vi "Main_Marvin Remake --.vi"() -> ()   [LabVIEW 2017]
uses:
  PCAN_Driver/ControlCAN.llb/DevType.ctl
  Marvin ATP Remake 1.5.18/PCAN_Driver/ControlCAN.llb/CAN Channel.ctl
  PCAN_Driver/ControlCAN.llb/VCI_INIT_CONFIG.ctl
  PCAN_Driver/ControlCAN.llb/InitFlag.ctl
  PCAN_Driver/ControlCAN.llb/Fliter.ctl
  PCAN_Driver/ControlCAN.llb/Mode.ctl
  <vilib>/Utility/miscctls.llb/LVRowAndColumnTypeDef.ctl
  <vilib>/Utility/sysdir.llb/System Directory Type.ctl
  <vilib>/Utility/config.llb/Read Key (String).vi
  <vilib>/Utility/config.llb/Write Key (String).vi
  <vilib>/Utility/cursorutil.llb/Set Cursor (Icon Pict).vi
  PCAN_Driver/ControlCAN.lvlib
  <vilib>/Utility/config.llb/NI_LVConfig.lvlib
panel:
  out "DSP Board S/N":string
  out "POWER Board S/N":string caption="DRIVER Board S/N"
  out "BurnInSpeed":u16
  out "SpeedCommandSpeed":u16
  out "VenableSpeed":u16
  out "CurrentTest":T1(ring)
  out "TesterVersion":string
  out "ClosePanel":bool=TRUE
  out "UUT SN Report":string
  out "Automation":bool
  out "Test Failed":bool
  out "AuxiOFFResult":bool
  out "AuxiONResult":bool
  out "SensCalResult":bool
  out "VisualInspectionResult":bool
  out "BurnResult":bool
  out "BurnSpeed":bool
  out "BurnTemp":bool
  out "BurnDC":bool
  out "TempControlResult":bool
  out "MotorTempResult":bool
  out "StopTimeResult":bool
  out "SpeedResult":bool=TRUE
  out "VenableDirectionResult":bool
  out "VenableResult":bool
  out "ComTestResult":bool=TRUE
  out "UUT SoftwareVer":string
  out "Next SN":i32
  in  "SetSN":bool
  out "Current SN":i32
  out "Cal":dbl
  out "AO[1]Meas":dbl
  out "FullSpeed2 Speed":dbl
  out "FullSpeed2 Current":dbl
  out "FullSpeed1 Current":dbl
  out "FullSpeed1 Speed":dbl
  out "MaxBurnInTempVal":dbl
  in  "Stop Burn-in":bool
  out "VISA Tester":refnum<visa-resource-name>
  out "UUT":u8
  out "CAN Status":bool
  in  "Channel 2":T2 caption="Channel" items=["Channel 1", "Channel 2"]
  out "Config_CANAT":T8 {"DevType" items=["USB-CAN"=3, "USB-CAN2"=4]; "CanIndex" items=["通道1", "通道2"]; "VCI_INIT_CONFIG"."Fliter" items=["接收所有类型"=3, "只接收标准帧"=4, "只接收扩展帧"=7]; "VCI_INIT_CONFIG"."Mode" items=["正常工作", "自测模式（环回）", "仅侦听模式"]; "VCI_INIT_CONFIG"."InitFlag" items=["使用Flash参数", "使用界面设置参数"]}
  out "Array":u64[][](array[numeric]) format="%016x"
  out "Motor Phase Current RMS":dbl
  out "Ambient Temperature":dbl
  out "Speed error":bool
  out "Commutation err":bool
  out "Under voltage/Over voltage":bool
  out "Derated drive temp":bool
  out "Motor Over temperature":bool
  out "Motor Sensor temp Fauilre":bool
  out "Drive Over temperature":bool
  out "Drive Sensor temp Failure":bool
  out "Ambient Over temp":bool
  out "Ambient Sensor temp":bool
  out "DC Voltage":dbl
  out "DC Current":dbl
  out "Power transistor Heat sink Temp.":dbl
  out "Motor Stator Temp.":dbl
  out "Motor Speed RPM":dbl
  out "ECS State":u16
  out "UUT":string="EBAY"
  in  "Logger Path":path
  in  "Report":bool
  in  "Start":bool
  in  "ATR":string[][](table)=[["Test Communication", "-", "-", "-", "-", ""], ["Set S/N", "-", "-", "-", "-", ""], ["Set Board Number", "-", "-", "-", "-", ""], [" ", "", "", "", "", ""], ["Test Communication", "-", "-", "-", "-", ""], ["Get S/N", "-", "-", "-", "", ""], ["Get Board Number", "-", "-", "-", "", ""], ["Get FW", "-", "-", "-", "", ""], ["Enable Motor", "", "", "", "", ""], ["Small position command", "", "", "", "", ""], ["Measure delta", "", "", "", "", ""], ["Velocity command", "", "", "", "", ""]]
  in  "Settings":bool
  in  "Refresh Button":bool
  out "Status":bool
  in  "VISA Marvin":refnum<visa-resource-name>="COM6"
  in  "Serial Com":bool
  in  "Help Button":bool
  out "Pannel User Message":string
  in  "Stop Button":bool
  # "Marvin"
  # "REDLER TECHNOLOGIES LTD"
  # "ver 1.2p"
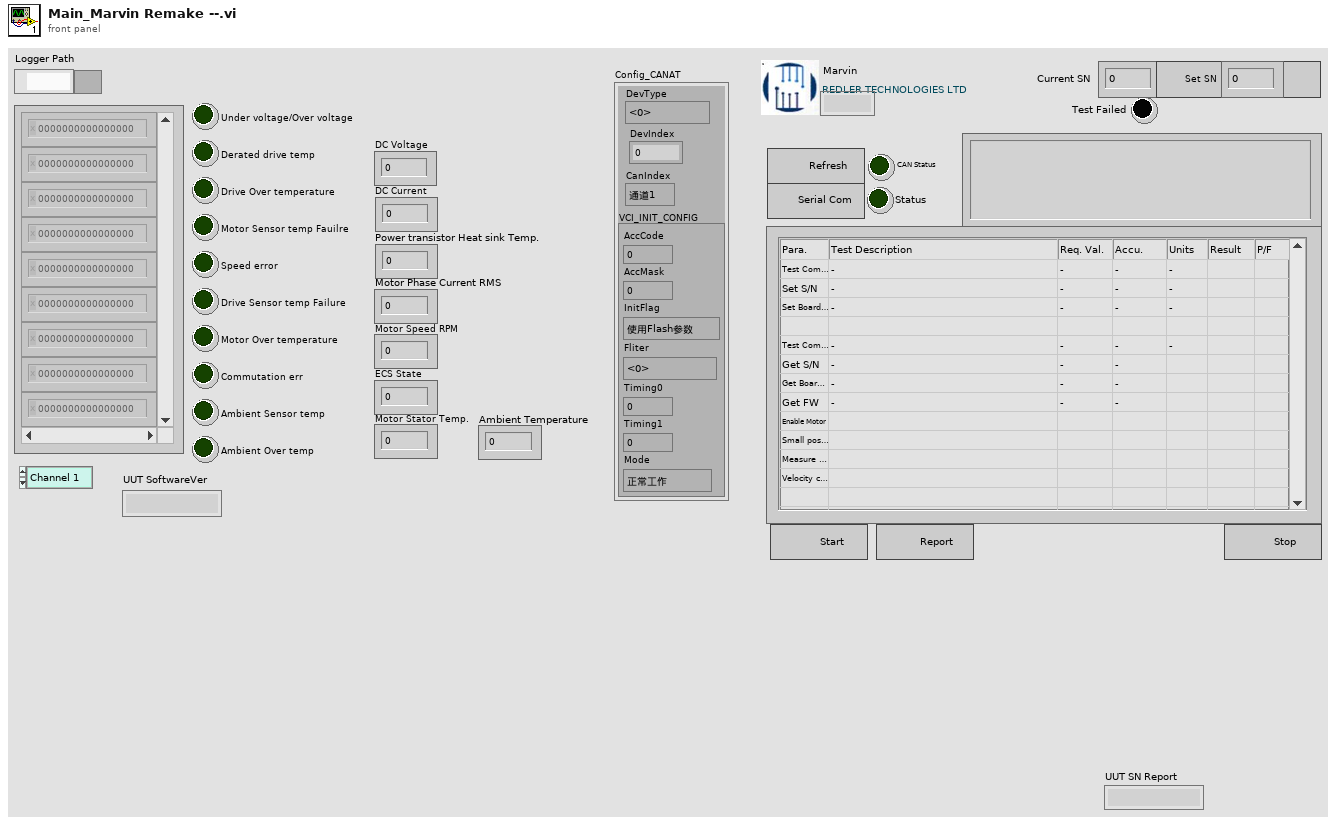
[diagram p1: front panel]
types:
  T1 = enum16{"Auxiliary", "Temp Sens Cal", "Com Test", "Enable Test", "Speed Command", "Stop Time", "Temp Control", "Burn in", "Visual Inspec", "Empty"}
  T2 = typedef "ControlCAN.lvlib/CAN Channel.ctl" = u32
  T3 = typedef "ControlCAN.lvlib/DevType.ctl" = u32
  T4 = typedef "ControlCAN.lvlib/VCI_INIT_CONFIG.ctl" = cluster{"AccCode":u32, "AccMask":u32, "InitFlag":T5, "Fliter":T6, "Timing0":u8, "Timing1":u8, "Mode":T7}
  T5 = typedef "ControlCAN.lvlib/InitFlag.ctl" = u32
  T6 = typedef "ControlCAN.lvlib/Fliter.ctl" = u8
  T7 = typedef "ControlCAN.lvlib/Mode.ctl" = u8
  T8 = cluster{"DevType":T3, "DevIndex":u32, "CanIndex":T2, "VCI_INIT_CONFIG":T4}
  T9 = cluster{"VISA":refnum<visa-resource-name>, "Array Test":enum16{"Auxiliary", "Temp Sens Cal", "Com Test", "Enable Test", "Speed Command", "Stop Time", "Temp Control", "Burn in", "Visual Inspec", "Empty"}[]}
  T10 = cluster{"ID":u32, "MSGTYPE":u8, "LEN":u8, "aDATA":u8[]}[]
  T11 = enum16{"Erase ATR Table", "Stop", "MainProgram", "Initialize"}
  T12 = typedef "NI_LVConfig.lvlib/Config Data RefNum.ctl" = refnum<k1>
  T13 = enum16{"K15", "K16", "K17", "Venable", "Firmeware", "Fan", "Power", "120C", "110C", "100C", "90C", "80C", "70C", "60C", "50C", "40C", "30C", "25C", "20C", "10C", "0C"}
  T14 = enum16{"Stop", "Result", "FullSpeed2", "MD[1]=1", "FullSpeed1", "MD[1]=0"}
  T15 = enum8{"Term1", "Term2", "Current", "Fan", "TempCPU"}
  T16 = enum16{"Stop", "AO[1]=Meas.", "TA[5]", "AO[1]=0", "Start"}
  T17 = enum16{"Stop", "BurnIn", "Ambient Temp", "MotorSpeed", "DC Current Measure", "Start"}
  T18 = enum16{"Auxiliary", "Temp Sens Cal", "Com Test", "Enable Test", "Speed Command", "Stop Time", "Temp Control", "Burn in", "Visual Inspec", "Empty"}[]
  T19 = enum16{"K15", "K16", "K17", "Venable", "Firmeware", "Fan", "Power", "120C", "110C", "100C", "90C", "80C", "70C", "60C", "50C", "40C", "30C", "25C", "20C", "10C", "0C"}[]
  T20 = enum32{"6000", "11500", "15100", "11500-2", "6000-2"}[]
  T21 = enum8{"Enabled", "Disabled", "Disabled and Grayed Out"}
  T22 = typedef "LVRowAndColumnTypeDef.ctl" = cluster{"Row":i32, "Column":i32}
  T23 = enum32{"Invalid", "Standard", "Closed", "Hidden", "Minimized", "Maximized"}
  T24 = cluster{"ID":u32, "MSGTYPE":u8, "LEN":u8, "aDATA":u8[]}
  T25 = enum16{"open", "replace", "create", "open or create", "replace or create", "replace or create with confirmation"}
  T26 = typedef "ControlCAN.lvlib/VCI_CAN_OBJ.ctl" = cluster{"ID":u32, "TimeStamp":u32, "TimeFlag":u8, "SendType":u8, "RemoteFlag":u8, "ExternFlag":u8, "DataLen":u8, "Data":u8[], "Reserved":u8[]}
  T27 = cluster{"Type":enum16{"接收", "发送"}, "Channel":T2, "Time":timestamp, "VCI_CAN_OBJ":T26}[]
  T28 = cluster{"Type":enum16{"接收", "发送"}, "Channel":T2, "Time":timestamp, "VCI_CAN_OBJ":T26}
  T29 = typedef "LVPoint32TypeDef.ctl" = cluster{"Horizontal":i32, "Vertical":i32}
  T30 = enum8{"Term1", "Term2", "Current", "Fan", "TempCPU"}[]
  T31 = typedef "System Directory Type.ctl" = i32
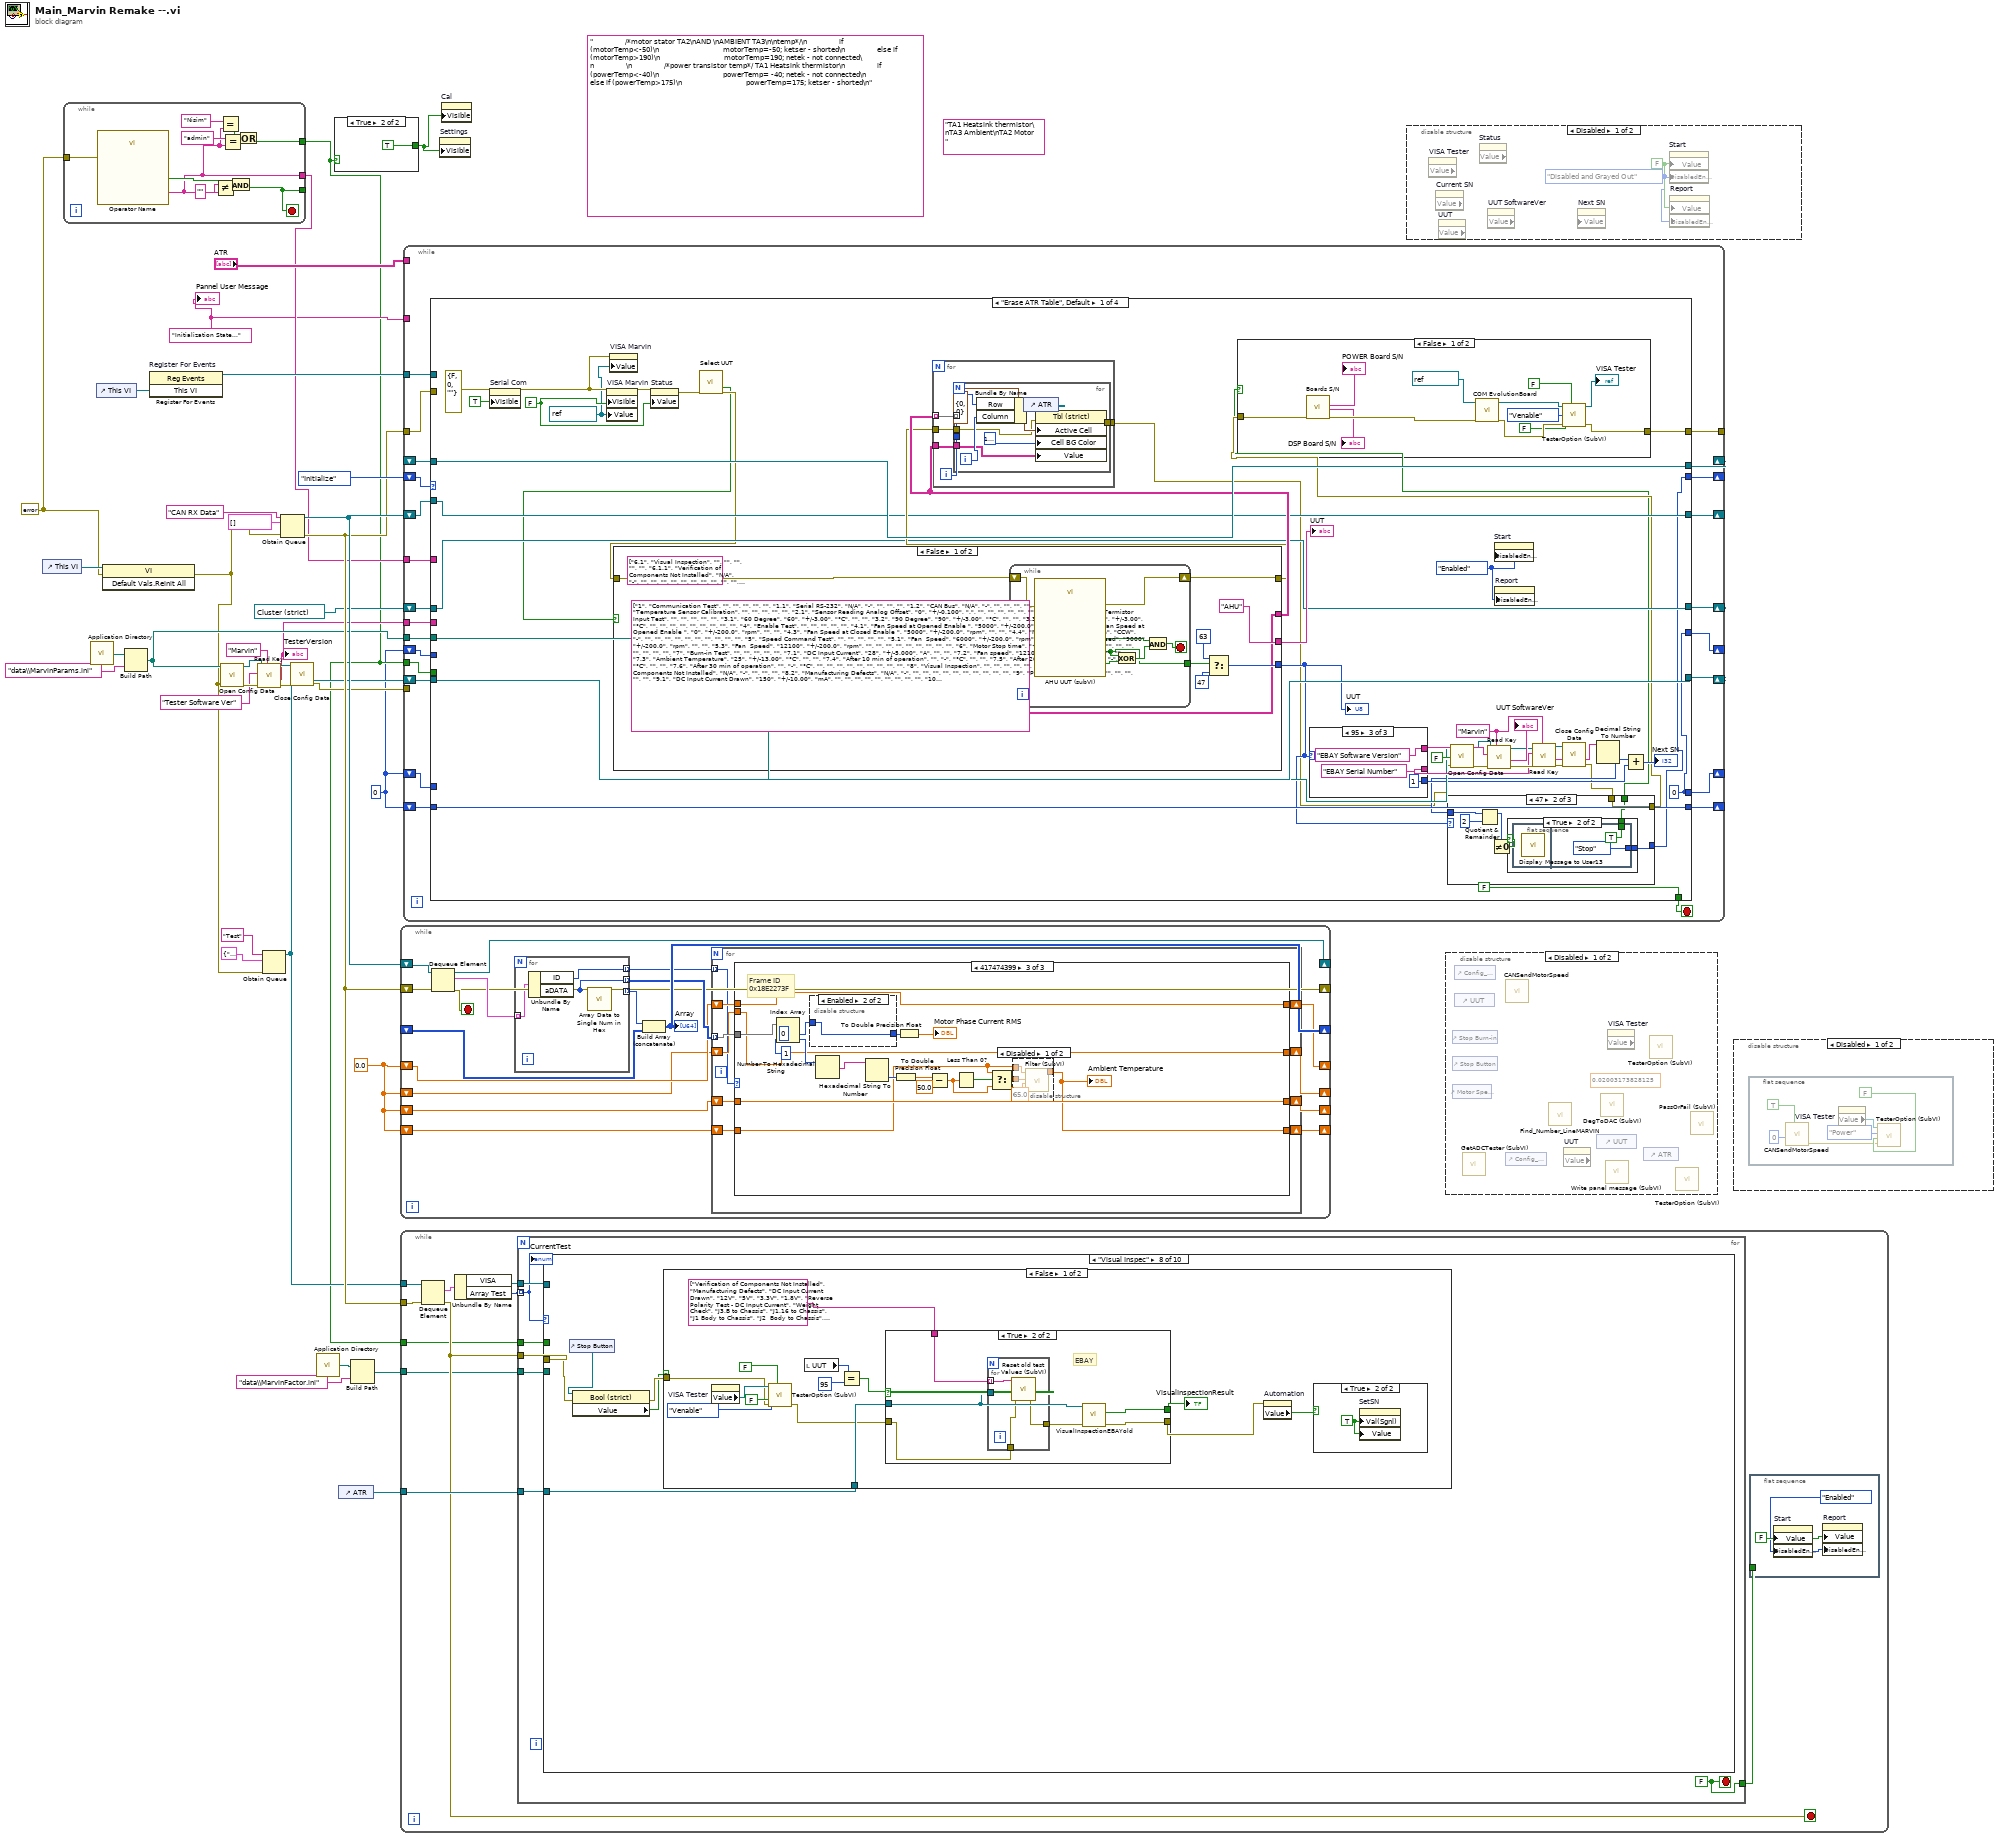
[diagram p0: block diagram]
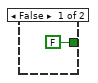
[diagram p2: hidden frame]
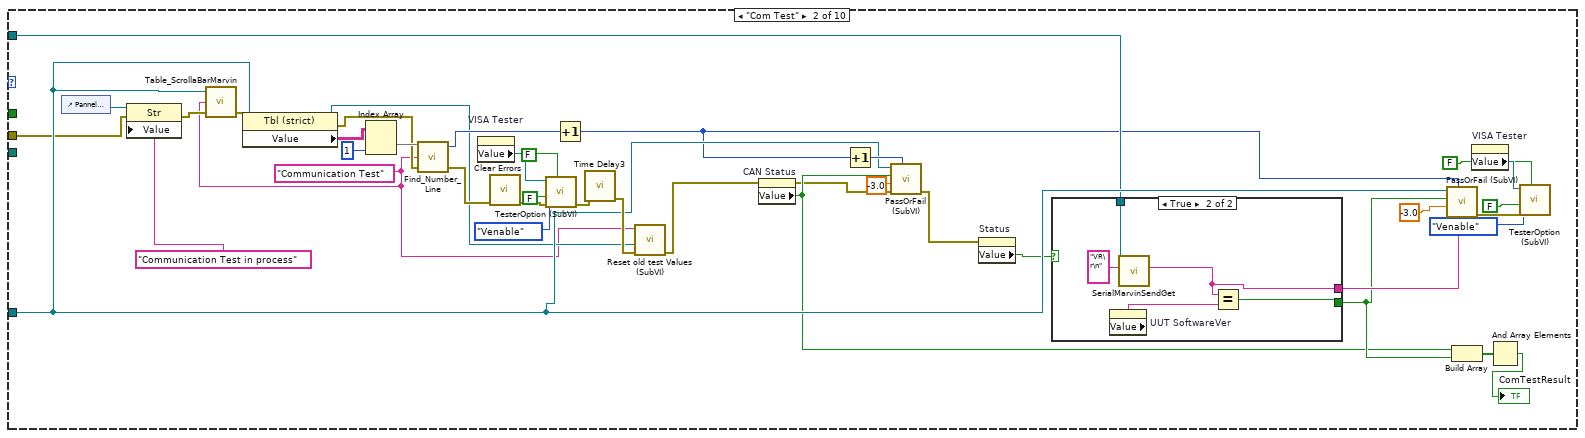
[diagram p7: hidden frame]
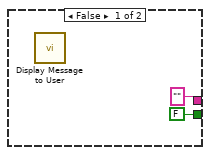
[diagram p8: hidden frame]
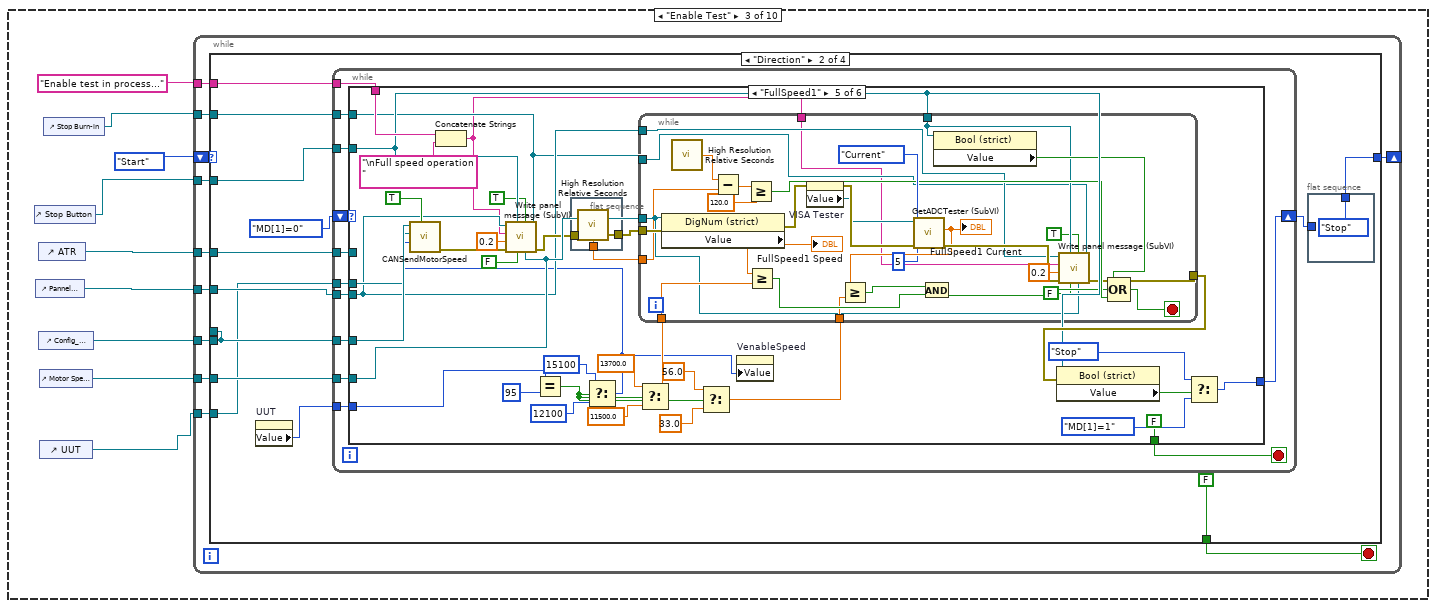
[diagram p9: hidden frame]
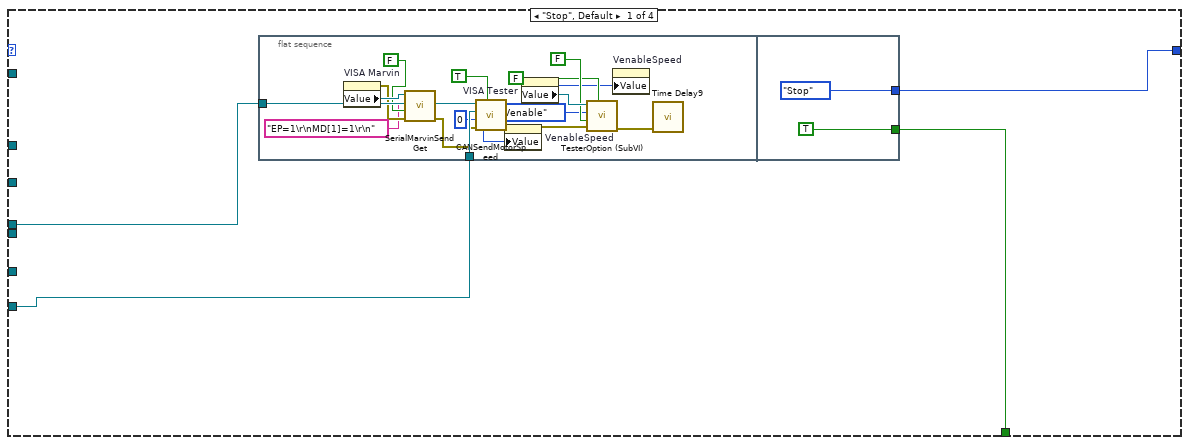
[diagram p10: hidden frame]
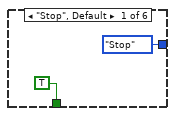
[diagram p11: hidden frame]
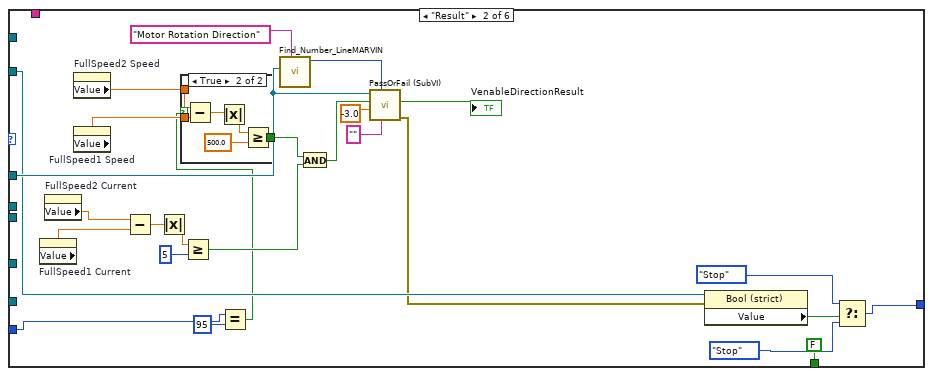
[diagram p12: hidden frame]
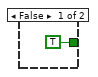
[diagram p13: hidden frame]
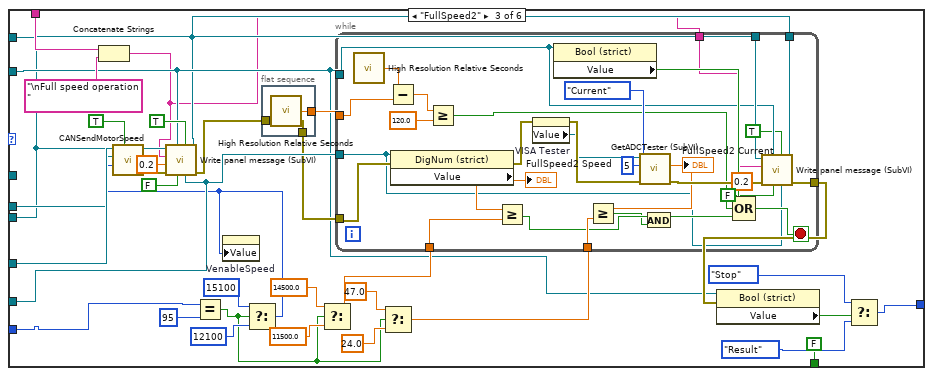
[diagram p14: hidden frame]
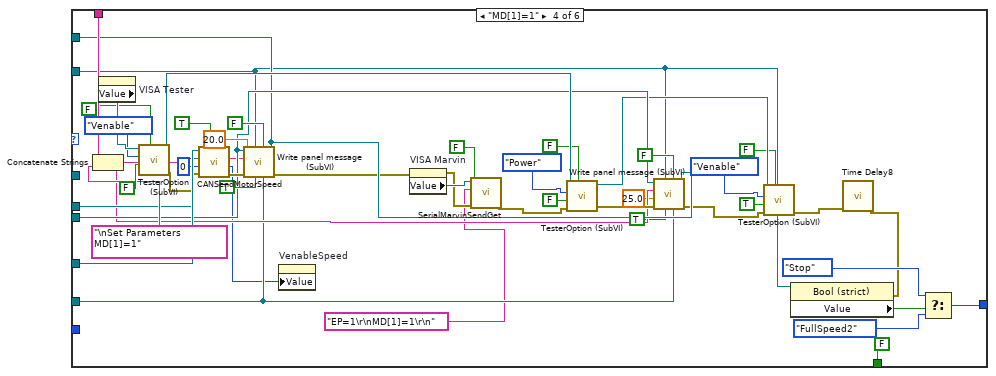
[diagram p15: hidden frame]
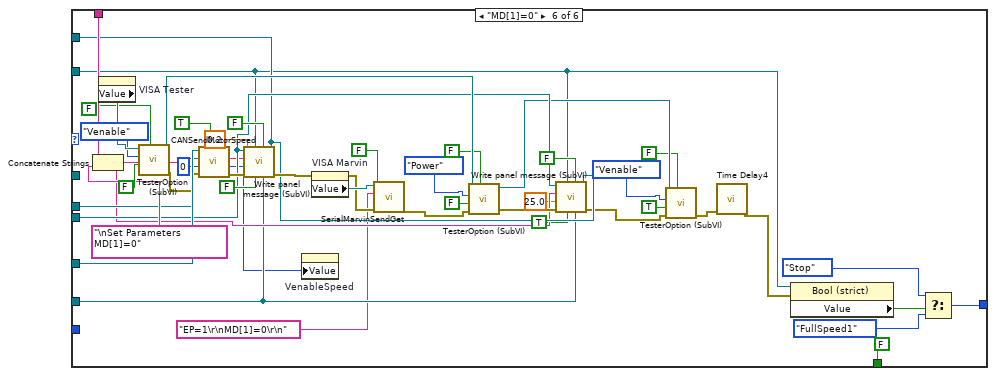
[diagram p16: hidden frame]
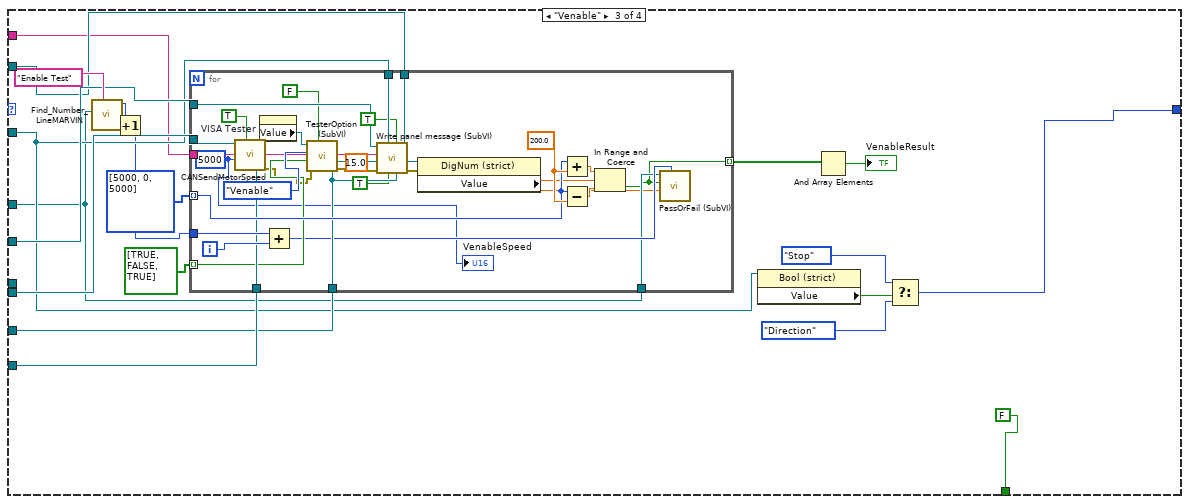
[diagram p17: hidden frame]
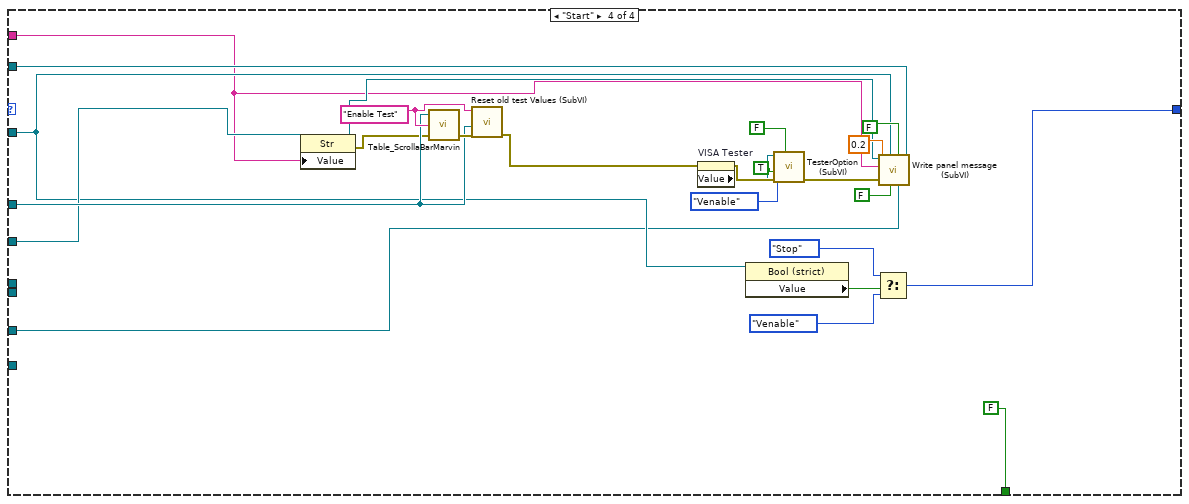
[diagram p18: hidden frame]
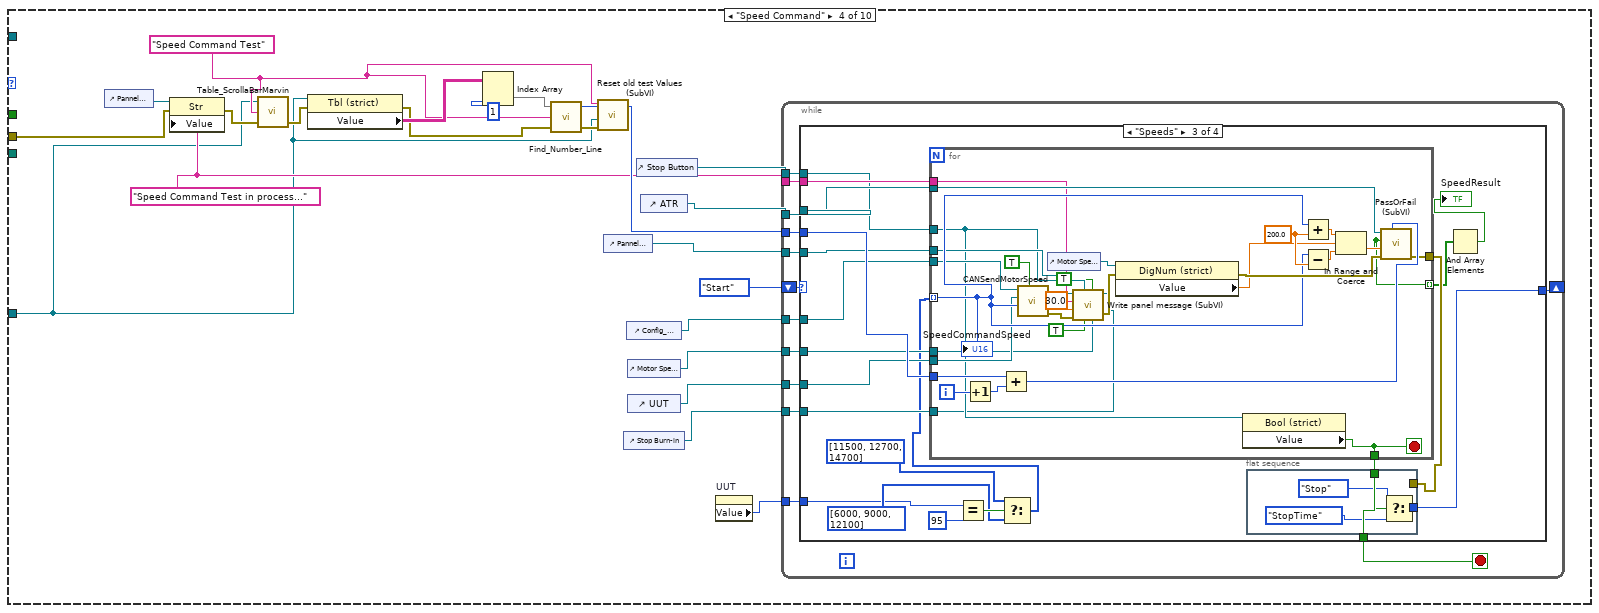
[diagram p19: hidden frame]
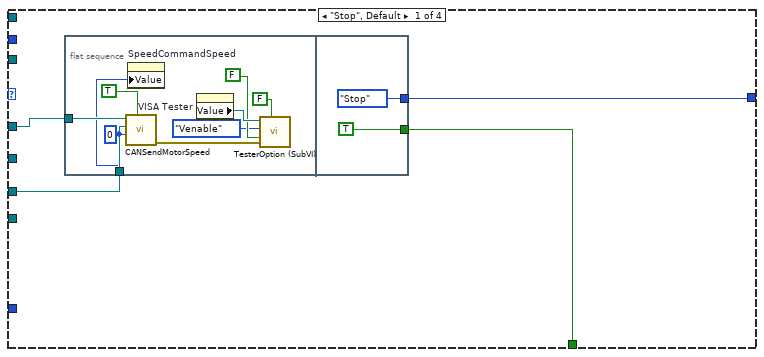
[diagram p20: hidden frame]
diagram:
  (unwired) "TA1 Heatsink thermistor\nTA3 Ambient\nTA2 Motor "
  (unwired) "                /*motor stator TA2\nAND \nAMBIENT TA3\n\ntemp*/\n                if (motorTemp<-50)\n                                motorTemp=-50; ketser - shorted\n                else if (motorTemp>190)\n                                motorTemp=190; netek - not connected\n                \n                /*power transistor temp*/ TA1 Heatsink thermistor\n                if (powerTemp<-40)\n                                powerTemp= -40; netek - not connected\n                else if (powerTemp>175)\n                                powerTemp=175; ketser - shorted\n"
  w19 = "Initialization State..."
  w1 = 0
  w26 = 0.0
  w4 = errorcluster {"status"=FALSE, "code"=0, "source"=""} ("error in (no error)")
  n1 = control-ref of="This VI"() -> (w5:refnum<vi>)
  n2 = while {
    tunnel: [w44] -> _
    tunnel: [w40] -> w21
    tunnel: [w41] -> w2
    tunnel: w4 -> [w37]
    stop <- w44 stop-if-true
    n3 = call "Operator Name"("error in (no error)"=w37) -> ("Operator Name"=w40:string, "OK"=w45:bool)  [unwired: 16 in, 1 out]
    n4 = Not Equal?(x=w40, y="") -> (x != y?=w46:bool)
    n5 = Equal?(x="Nisim", y=w40) -> (x = y?=w38:bool)
    n6 = Equal?(x="admin", y=w40) -> (x = y?=w42:bool)
    n7 = And(x=w45, y=w46) -> (x .and. y?=w44:bool)
    n8 = Or(x=w38, y=w42) -> (x .or. y?=w41:bool)
  }
  n9 = call <vilib>:"Application Directory.vi"() -> ("Application Directory"=w25:path)
  n10 = control-ref of="This VI"() -> (w23:refnum<vi>)
  n11 = invoke class="VI" method="Default Vals.Reinit All"(reference=w5, error in=w4) -> (error out=w3:errorcluster)  [unwired: 1 in, 2 out]
  n12 = Build Path(base path=w25, name or relative path="data\\MarvinParams.ini") -> (appended path=w8:path)
  n13 = register-events "Register For Events"(w23) -> (reference out=w22:refnum<event-registration>)  [unwired: 2 in, 1 out]
  n14 = call <vilib>:"Open Config Data.vi"("error in (no error)"=w3, "configuration file path"=w8) -> ("error out"=w14:errorcluster, "refnum"=w13:T12)  [unwired: 1 in, 7 out]
  n15 = call-poly <vilib>:"Read Key.vi"("section"="Marvin", "error in (no error)"=w14, "key"="Tester Software Ver", "refnum"=w13) -> ("error out"=w11:errorcluster, "value"=w6:string, "refnum out"=w10:T12)  [unwired: 2 in, 3 out]
  "TesterVersion" <- w6
  n16 = Obtain Queue(name (unnamed)="Test", element data type=T9 {"VISA"="COM1", "Array Test"=[]}, error in (no error)=w3) -> (queue out=w30:refnum<queue>)  [unwired: 2 in, 2 out]
  n17 = Obtain Queue(name (unnamed)="CAN RX Data", element data type=T10 [], error in (no error)=w3) -> (queue out=w33:refnum<queue>, error out=w31:errorcluster)  [unwired: 2 in, 1 out]
  n18 = call <vilib>:"Close Config Data.vi"("error in (no error)"=w11, "refnum"=w10) -> ("error out"=w9:errorcluster)  [unwired: 8 in, 1 out]
  n19 = call <vilib>:"Application Directory.vi"() -> ("Application Directory"=w16:path)
  n20 = case shown="True" w2 {
    tunnel: [FALSE TRUE] -> w20
    frame False {
    }
    frame True {
    }
  }
  n21 = control-ref of="ATR"() -> (w18:refnum<vi>)
  n22 = Build Path(base path=w16, name or relative path="data\\MarvinFactor.ini") -> (appended path=w15:path)
  n23 = while {
    shift-right: [w65] -> _
    shift-left: w33 -> [w67]
    shift-right: [w63] -> _
    shift-left: _ -> [w64]
    shift-right: [w59] -> _
    shift-left: w31 -> [w59]
    shift-right: [w57] -> _
    shift-left: w26 -> [w58]
    shift-right: [w56] -> _
    shift-left: w26 -> [w55]
    shift-right: [w54] -> _
    shift-left: w26 -> [w53]
    shift-right: [w52] -> _
    shift-left: w26 -> [w51]
    stop <- w66 stop-if-true
    n24 = Dequeue Element(queue=w67, error in (no error)=w59) -> (queue out=w65:refnum<queue>, element=w60:T10, error out=w66:errorcluster)  [unwired: 1 in, 1 out]
    n25 = for {
      tunnel: [w213] -> w62 mode=indexing
      tunnel: w60 -> [w212] mode=indexing
      tunnel: [w211] -> w61 mode=indexing
      tunnel: [w210] -> w50 mode=indexing
      n26 = Unbundle By Name(w212) -> ("ID"=w210:u32, "aDATA"=w211:u8[])
      n27 = call "Array Data to Single Num in Hex.vi"("aDATA"=w211) -> ("Numeric"=w213:u64)  [unwired: 10 in]
    }
    n28 = Build Array (concatenate)(w62, w64) -> (w63:u64[][])
    "Array" <- w63
    n29 = for {
      tunnel: w61 -> [w77] mode=indexing
      shift-right: [w75] -> w57
      shift-left: w58 -> [w76]
      shift-right: [w74] -> w56
      shift-left: w55 -> [w73]
      shift-right: [w72] -> w54
      shift-left: w53 -> [w71]
      shift-right: [w70] -> w52
      shift-left: w51 -> [w69]
      tunnel: w50 -> [w68] mode=indexing
      n30 = case shown="417474399" w68 {
        tunnel: w77 -> [w114 w162 w200]
        tunnel: w76 -> [w88 w151 w189]
        tunnel: [w87 w151 w189] -> w75
        tunnel: [w84 w150 w188] -> w74
        tunnel: w73 -> [w83 w150 w188]
        tunnel: [w80 w149 w187] -> w72
        tunnel: w71 -> [w79 w149 w187]
        tunnel: [w78 w148 w183] -> w70
        tunnel: w69 -> [w78 w148 w182]
        frame 417408863, Default {
          # "Frame ID\n0x18E1273F"
          n31 = Index Array(array=w114, index #1=0 ("index"), index #2=1 ("index"), index #3=2 ("index"), index #4=3 ("index"), index #5=4 ("index"), index #6=5 ("index"), index #7=6 ("index"), index #8=7 ("index")) -> (element #1=w98:u8, element #2=w100:u8, element #3=w101:u8, element #4=w105:u8, element #5=w108:u8, element #6=w112:u8, element #7=w113:u8, element #8=w111:u8)
          n32 = Number To Hexadecimal String(2:w111) -> (0:w125:string)  [unwired: 1 in]
          n33 = Join Numbers(hi=w113, lo=w112) -> ((hi.lo)=w132:u16)
          n34 = Join Numbers(hi=w101, lo=w100) -> ((hi.lo)=w102:u16)
          n35 = Number To Hexadecimal String(2:w108) -> (0:w109:string)  [unwired: 1 in]
          n36 = Number To Hexadecimal String(2:w132) -> (0:w131:string)  [unwired: 1 in]
          n37 = Number To Hexadecimal String(2:w98) -> (0:w99:string)  [unwired: 1 in]
          n38 = Number To Hexadecimal String(2:w102) -> (0:w103:string)  [unwired: 1 in]
          n39 = Number To Hexadecimal String(2:w105) -> (0:w106:string)  [unwired: 1 in]
          n40 = Hexadecimal String To Number(string=w125) -> (number=w124:u32)  [unwired: 2 in, 1 out]
          n41 = To Double Precision Float(number=w124) -> (double precision float=→"DC Current":dbl)
          n42 = Hexadecimal String To Number(string=w109) -> (number=w110:u32)  [unwired: 2 in, 1 out]
          n43 = Hexadecimal String To Number(string=w131) -> (number=w130:u32)  [unwired: 2 in, 1 out]
          n44 = Hexadecimal String To Number(string=w99) -> (number=w96:u32)  [unwired: 2 in, 1 out]
          n45 = Hexadecimal String To Number(string=w103) -> (number=w104:u32)  [unwired: 2 in, 1 out]
          n46 = Hexadecimal String To Number(string=w106) -> (number=w107:u32)  [unwired: 2 in, 1 out]
          n47 = To Double Precision Float(number=u32 10 ("y")) -> (double precision float=w128:dbl)
          n48 = To Double Precision Float(number=w130) -> (double precision float=w127:dbl)
          n49 = To Double Precision Float(number=w110) -> (double precision float=w93:dbl)
          n50 = To Double Precision Float(number=w104) -> (double precision float=w89:dbl)
          n51 = To Double Precision Float(number=w107) -> (double precision float=w95:dbl)
          n52 = Divide(x=w127, y=w128) -> (x/y=→"DC Voltage":dbl)
          n53 = To Unsigned Word Integer(number=w96) -> (unsigned 16bit integer=→"ECS State":u16)
          n54 = disable-structure shown="Enabled" {
            disable-tunnel: w89 -> [w146 w147]
            disable-tunnel: w88 -> [w145 _]
            disable-tunnel: [w143 w147] -> w87
            frame Disabled {
              n55 = call "Filter (SubVI).vi"("Delta"=5000.0, "NewVal"=w146, "OldVal"=w145) -> ("Val"=w143:dbl)  [unwired: 8 in]
            }
            frame Enabled {
            }
          }
          "Motor Speed RPM" <- w87
          n56 = Subtract(x=w93, y=50.0 ("x")) -> (x-y=w82:dbl)
          n57 = Subtract(x=w95, y=50.0 ("x")) -> (x-y=w85:dbl)
          n58 = Less Than 0?(x=w85) -> (x < 0?=w91:bool)
          n59 = Less Than 0?(x=w82) -> (x < 0?=w90:bool)
          n60 = Select(t=w83, s=w91, f=w85) -> (s? t:f=w86:dbl)
          n61 = Select(t=w79, s=w90, f=w82) -> (s? t:f=w81:dbl)
          n62 = disable-structure shown="Enabled" {
            disable-tunnel: w86 -> [w141 w142]
            disable-tunnel: [w140 w142] -> w84
            disable-tunnel: w83 -> [w139 _]
            frame Disabled {
              n63 = call "Filter (SubVI).vi"("Delta"=130.0, "NewVal"=w141, "OldVal"=w139) -> ("Val"=w140:dbl)  [unwired: 8 in]
            }
            frame Enabled {
            }
          }
          "Motor Stator Temp." <- w84
          n64 = disable-structure shown="Enabled" {
            disable-tunnel: w81 -> [w136 w137]
            disable-tunnel: [w134 w137] -> w80
            disable-tunnel: w79 -> [w133 _]
            frame Disabled {
              n65 = call "Filter (SubVI).vi"("Delta"=100.0, "NewVal"=w136, "OldVal"=w133) -> ("Val"=w134:dbl)  [unwired: 8 in]
            }
            frame Enabled {
            }
          }
          "Power transistor Heat sink Temp." <- w80
        }
        frame 417539935 {
          # "Framde ID\n0x18E3273F"
          n66 = control-ref of="UUT"() -> (w152:refnum<vi>)
          n67 = property on="Property Node" class="DigNum (strict)"(reference=w152) -> ("Value"=w153:u8)  [unwired: 1 in, 2 out]
          n68 = Index Array(array=w162, index #1=0 ("index"), index #2=1 ("index")) -> (element #1=w160:u8, element #2=w155:u8)
          n69 = Number To Boolean Array(number=w160) -> (Boolean array=w159:bool[])
          n70 = Number To Boolean Array(number=w155) -> (Boolean array=w157:bool[])
          n71 = Boolean To (0,1)(Boolean=w157) -> (0, 1=w154:i16[])
          n72 = Boolean To (0,1)(Boolean=w159) -> (0, 1=w158:i16[])
          n73 = case shown="95" w153 {
            tunnel: w154 -> [_ w163]
            frame 0, Default {
            }
            frame 95 {
              n74 = for {
                tunnel: w163 -> [w168] mode=indexing
                i -> [w164]
                stop <- w166 stop-if-true
                n75 = Not Equal To 0?(x=w168) -> (x != 0?=w167:bool)
                n76 = case shown="0, Default" w164 {
                  tunnel: w167 -> [w169 w170]
                  frame 0, Default {
                    "Ambient Sensor temp" <- w169
                  }
                  frame 1 {
                    "Ambient Over temp" <- w170
                  }
                }
                n77 = Equal?(x=w164, y=1.0) -> (x = y?=w166:bool)
              }
            }
          }
          n78 = for {
            tunnel: w158 -> [w172] mode=indexing
            i -> [w173]
            n79 = Not Equal To 0?(x=w172) -> (x != 0?=w171:bool)
            n80 = case shown="1" w173 {
              tunnel: w171 -> [w174 w175 w176 w177 w178 w179 w180 w181]
              frame 0, Default {
                "Drive Sensor temp Failure" <- w174
              }
              frame 1 {
                "Drive Over temperature" <- w175
              }
              frame 2 {
                "Motor Sensor temp Fauilre" <- w176
              }
              frame 3 {
                "Motor Over temperature" <- w177
              }
              frame 4 {
                "Derated drive temp" <- w178
              }
              frame 5 {
                "Under voltage/Over voltage" <- w179
              }
              frame 6 {
                "Commutation err" <- w180
              }
              frame 7 {
                "Speed error" <- w181
              }
            }
          }
        }
        frame 417474399 {
          # "Frame ID\n0x18E2273F"
          n81 = Index Array(array=w200, index #1=0 ("index"), index #2=1 ("index")) -> (element #1=w197:u8, element #2=w194:u8)
          n82 = disable-structure shown="Enabled" {
            disable-tunnel: [w208 w209] -> w198
            disable-tunnel: w197 -> [w207 w209]
            frame Disabled {
              n83 = Number To Hexadecimal String(2:w207) -> (0:w206:string)  [unwired: 1 in]
              n84 = Hexadecimal String To Number(string=w206) -> (number=w208:u32)  [unwired: 2 in, 1 out]
            }
            frame Enabled {
            }
          }
          n85 = Number To Hexadecimal String(2:w194) -> (0:w192:string)  [unwired: 1 in]
          n86 = Hexadecimal String To Number(string=w192) -> (number=w193:u32)  [unwired: 2 in, 1 out]
          n87 = To Double Precision Float(number=w193) -> (double precision float=w191:dbl)
          n88 = To Double Precision Float(number=w198) -> (double precision float=→"Motor Phase Current RMS":dbl)
          n89 = Subtract(x=w191, y=50.0) -> (x-y=w185:dbl)
          n90 = Less Than 0?(x=w185) -> (x < 0?=w186:bool)
          n91 = Select(t=w182, s=w186, f=w185) -> (s? t:f=w184:dbl)
          n92 = disable-structure shown="Disabled" {
            disable-tunnel: w184 -> [w204 w205]
            disable-tunnel: [w202 w205] -> w183
            disable-tunnel: w182 -> [w201 _]
            frame Disabled {
              n93 = call "Filter (SubVI).vi"("Delta"=65.0, "NewVal"=w204, "OldVal"=w201) -> ("Val"=w202:dbl)  [unwired: 8 in]
            }
            frame Enabled {
            }
          }
          "Ambient Temperature" <- w183
        }
      }
    }
  }
  n94 = while {
    tunnel: w18 -> [w223]
    tunnel: w31 -> [w221]
    tunnel: w30 -> [w222]
    tunnel: w15 -> [w215]
    tunnel: w2 -> [w214]
    stop <- w217 stop-if-true
    n95 = Dequeue Element(queue=w222, error in (no error)=w221) -> (element=w220:T9, error out=w217:errorcluster)  [unwired: 1 in, 2 out]
    n96 = Unbundle By Name(w220) -> ("VISA"=w219:refnum<visa-resource-name>, "Array Test"=w218:T18)
    n97 = for {
      tunnel: w218 -> [w229] mode=indexing
      tunnel: w219 -> [w232]
      tunnel: w223 -> [w231]
      tunnel: w217 -> [w230]
      tunnel: [w228] -> w216
      tunnel: w215 -> [w227]
      tunnel: w214 -> [w226]
      stop <- w228 stop-if-true
      w228 = FALSE
      n98 = case shown="\"Visual Inspec\"" w229 {
        tunnel: w232 -> [_ w257 _ _ w846 _ _ _ w1453 w1660]
        tunnel: w231 -> [_ w264 _ w681 w842 w1019 _ w1413 w1460 w1673]
        tunnel: w230 -> [_ w261 _ w696 w852 w1001 _ w1411 w1458 w1672]
        tunnel: w227 -> [_ _ _ _ _ w1003 _ _ _ _]
        tunnel: w226 -> [_ _ _ _ _ _ w1171 _ _ _]
        frame "Empty", Default {
        }
        frame "Com Test" {
          w240 = "Communication Test" ("Test Paragraph")
          n99 = control-ref of="Pannel User Message"() -> (w262:refnum<vi>)
          n100 = property class="Str"(reference=w262, error in=w261, "Value"="Communication Test in process") -> (error out=w260:errorcluster)  [unwired: 1 out]
          n101 = call "Table_ScrollaBarMarvin.vi"("error in"=w260, "Line to focus"=w240, "reference in"=w264) -> ("error out"=w263:errorcluster)  [unwired: 2 out]
          n102 = property class="Tbl (strict)"(reference=w264, error in=w263) -> (reference out=w241:refnum<vi>, error out=w270:errorcluster, "Value"=w271:string[][])
          n103 = Index Array(array=w271, index (col)=1 ("disabled index (col)")) -> (element=w272:string[])  [unwired: 1 in]
          n104 = call "Find_Number_Line.vi"("error in"=w270, "Test Paragraph"=w240, "Row Headers[]"=w272) -> ("error out"=w268:errorcluster, "Line number"=w267:i32)  [unwired: 1 out]
          n105 = property on="VISA Tester" class="VISAName"() -> ("Value"=w251:refnum<visa-resource-name>)  [unwired: 2 in, 2 out]
          n106 = call <vilib>:"Clear Errors.vi"("error in (no error)"=w268) -> ("error out"=w253:errorcluster)  [unwired: 5 in, 1 out]
          n107 = call "TesterOption (SubVI).vi"("2 Options"=FALSE, "error in (no error)"=w253, "On/Off"=FALSE, "Tester Option"=T13."Venable", "VISA Refnum in"=w251) -> ("error out"=w252:errorcluster)  [unwired: 5 in, 1 out]
          n108 = Increment(x=w267) -> (x+1=w233:i32)
          n109 = call "Time Delay3"("error in (no error)"=w252) -> ("error out"=w265:errorcluster)  [unwired: 10 in]
          n110 = call "Reset old test Values (SubVI).vi"("error in"=w265, "Atr in"=w241, "Test Paragraph"=w240) -> ("error out"=w235:errorcluster)  [unwired: 8 in]
          n111 = property on="CAN Status" class="Bool (strict)"(error in=w235) -> (error out=w234:errorcluster, "Value"=w236:bool)  [unwired: 1 in, 1 out]
          n112 = Increment(x=w233) -> (x+1=w266:i32)
          n113 = call "PassOrFail (SubVI).vi"("index (row)"=w266, "error in (no error)"=w234, "Data in"=-3.0, "Pass?Fail"=w236, "Table in"=w264) -> ("error out"=w256:errorcluster)  [unwired: 6 in]
          n114 = property on="Status" class="Bool (strict)"(error in=w256) -> ("Value"=w258:bool)  [unwired: 1 in, 2 out]
          n115 = case shown="True" w258 {
            tunnel: w257 -> [_ w279]
            tunnel: [FALSE w276] -> w238
            tunnel: ["" ("read buffer") w275] -> w255
            frame False {
              n116 = call "Display Message to User"() -> ()  [unwired: 10 in, 2 out]
            }
            frame True {
              n117 = property on="UUT SoftwareVer" class="Str"() -> ("Value"=w277:string)  [unwired: 2 in, 2 out]
              n118 = call "SerialMarvinSendGet.vi"("write buffer"="VR\r\n", "VISA resource name"=w279) -> ("read buffer"=w275:string)  [unwired: 8 in, 1 out]
              n119 = Equal?(x=w275, y=w277) -> (x = y?=w276:bool)
            }
          }
          n120 = call "PassOrFail (SubVI).vi"("String Res"=w255, "index (row)"=w233, "Data in"=-3.0, "Pass?Fail"=w238, "Table in"=w264) -> ("error out"=w247:errorcluster)  [unwired: 6 in]
          n121 = Build Array(w236, w238) -> (w239:bool[])
          n122 = property on="VISA Tester" class="VISAName"() -> ("Value"=w246:refnum<visa-resource-name>)  [unwired: 2 in, 2 out]
          n123 = And Array Elements(Boolean array=w239) -> (logical AND=→"ComTestResult":bool)
          n124 = call "TesterOption (SubVI).vi"("2 Options"=FALSE, "error in (no error)"=w247, "On/Off"=FALSE, "Tester Option"=T13."Venable", "VISA Refnum in"=w246) -> ()  [unwired: 5 in, 2 out]
        }
        frame "Enable Test" {
          n125 = control-ref of="Stop Button"() -> (w282:refnum<vi>)
          n126 = control-ref of="Pannel User Message"() -> (w284:refnum<vi>)
          n127 = control-ref of="ATR"() -> (w283:refnum<vi>)
          n128 = control-ref of="Config_CANAT"() -> (w285:refnum<vi>)
          n129 = control-ref of="Motor Speed RPM"() -> (w286:refnum<vi>)
          n130 = control-ref of="UUT"() -> (w287:refnum<vi>)
          n131 = control-ref of="Stop Burn-in"() -> (w288:refnum<vi>)
          n132 = while {
            shift-right: [w293] -> _
            shift-left: enum16{"Stop", "Direction", "Venable", "Start"}."Start" -> [w299]
            tunnel: w282 -> [w298]
            tunnel: w283 -> [w297]
            tunnel: w284 -> [w296]
            tunnel: w285 -> [w289]
            tunnel: w286 -> [w295]
            tunnel: w287 -> [w290]
            tunnel: w288 -> [w292]
            tunnel: "Enable test in process..." ("Strin") -> [w291]
            stop <- w294 stop-if-true
            n133 = case shown="\"Direction\"" w299 {
              tunnel: w298 -> [_ w331 w613 w660]
              tunnel: w297 -> [_ w326 w611 w667]
              tunnel: w296 -> [_ w329 w615 w666]
              tunnel: w289 -> [_ w332 w618 _]
              tunnel: w295 -> [_ w328 w616 w658]
              tunnel: w290 -> [w300 w322 w617 _]
              tunnel: [w303 FALSE FALSE FALSE] -> w294
              tunnel: [w301 w325 w612 w664] -> w293
              tunnel: w292 -> [_ w330 w614 w659]
              tunnel: w291 -> [_ w327 w610 w657]
              tunnel: w289 -> [w302 _ _ _]
              frame "Stop", Default {
                n134 = flat-sequence {
                  tunnel: w300 -> [w315]
                  tunnel: w302 -> [w314]
                  tunnel: [TRUE] -> w303
                  tunnel: [enum16{"Stop", "Direction", "Venable", "Start"}."Stop"] -> w301
                  frame #0 {
                    w304 = u16 0 ("Motor Speed RPM")
                    n135 = property on="VISA Marvin" class="VISAName"() -> (error out=w308:errorcluster, "Value"=w309:refnum<visa-resource-name>)  [unwired: 2 in, 1 out]
                    n136 = call "SerialMarvinSendGet.vi"("error in (no error)"=w308, "Clear Log"=FALSE, "write buffer"="EP=1\r\nMD[1]=1\r\n", "VISA resource name"=w309) -> ("error out"=w305:errorcluster)  [unwired: 6 in, 1 out]
                    n137 = call "CANSendMotorSpeed.vi"("Remote"=TRUE, "error in (no error)"=w305, "Motor Speed RPM"=w304, "UUT"=w315, "CAN Cluster in"=w314) -> ("error out"=w317:errorcluster)  [unwired: 6 in]
                    n138 = property on="VenableSpeed" class="DigNum (strict)"("Value"=w304) -> ()  [unwired: 2 in, 2 out]
                    n139 = property on="VISA Tester" class="VISAName"() -> ("Value"=w318:refnum<visa-resource-name>)  [unwired: 2 in, 2 out]
                    n140 = call "TesterOption (SubVI).vi"("2 Options"=FALSE, "error in (no error)"=w317, "On/Off"=FALSE, "Tester Option"=T13."Venable", "VISA Refnum in"=w318) -> ("error out"=w310:errorcluster)  [unwired: 5 in, 1 out]
                    n141 = property on="VenableSpeed" class="DigNum (strict)"("Value"=w304) -> ()  [unwired: 2 in, 2 out]
                    n142 = call "Time Delay9"("error in (no error)"=w310) -> ()  [unwired: 10 in, 1 out]
                  }
                  frame #1 {
                  }
                }
              }
              frame "Direction" {
                n143 = property on="UUT" class="DigNum (strict)"() -> ("Value"=w321:u8)  [unwired: 2 in, 2 out]
                n144 = while {
                  shift-right: [w345] -> w324
                  shift-left: T14."MD[1]=0" -> [w346]
                  tunnel: w332 -> [w343]
                  tunnel: w322 -> [w342]
                  tunnel: w331 -> [w341]
                  tunnel: w330 -> [w340]
                  tunnel: w329 -> [w339]
                  tunnel: w328 -> [w338]
                  tunnel: w327 -> [w337]
                  tunnel: w326 -> [w336]
                  tunnel: w321 -> [w335]
                  stop <- w344 stop-if-true
                  n145 = case shown="\"FullSpeed1\"" w346 {
                    tunnel: [T14."Stop" w370 w412 w492 w525 w605] -> w345
                    tunnel: [TRUE FALSE FALSE FALSE FALSE FALSE] -> w344
                    tunnel: w343 -> [_ _ w410 w486 w523 w599]
                    tunnel: w342 -> [_ _ w406 w466 w519 w578]
                    tunnel: w341 -> [_ w357 w386 w457 w502 w568]
                    tunnel: w340 -> [_ _ w384 w467 w500 w579]
                    tunnel: w339 -> [_ _ w385 w468 w501 w580]
                    tunnel: w338 -> [_ _ w402 w455 w516 w574]
                    tunnel: w337 -> [_ _ w397 w476 w514 w588]
                    tunnel: w336 -> [_ w361 _ _ _ _]
                    tunnel: w335 -> [_ w349 w382 _ w495 _]
                    frame "Stop", Default {
                    }
                    frame "Result" {
                      n146 = property on="FullSpeed1 Current" class="DigNum (strict)"() -> ("Value"=w365:dbl)  [unwired: 2 in, 2 out]
                      n147 = property on="FullSpeed2 Current" class="DigNum (strict)"() -> ("Value"=w366:dbl)  [unwired: 2 in, 2 out]
                      n148 = property on="FullSpeed2 Speed" class="DigNum (strict)"() -> ("Value"=w368:dbl)  [unwired: 2 in, 2 out]
                      n149 = property on="FullSpeed1 Speed" class="DigNum (strict)"() -> ("Value"=w367:dbl)  [unwired: 2 in, 2 out]
                      n150 = Subtract(x=w366, y=w365) -> (x-y=w364:dbl)
                      n151 = Absolute Value(x=w364) -> (abs(x)=w353:dbl)
                      n152 = Greater Or Equal?(x=w353, y=u32 5) -> (x >= y?=w359:bool)
                      n153 = Equal?(x=w349, y=u8 95) -> (x = y?=w351:bool)
                      n154 = case shown="True" w351 {
                        tunnel: w368 -> [_ w379]
                        tunnel: w367 -> [_ w378]
                        tunnel: [TRUE w375] -> w360
                        frame False {
                        }
                        frame True {
                          n155 = Subtract(x=w379, y=w378) -> (x-y=w380:dbl)
                          n156 = Absolute Value(x=w380) -> (abs(x)=w377:dbl)
                          n157 = Greater Or Equal?(x=w377, y=500.0) -> (x >= y?=w375:bool)
                        }
                      }
                      n158 = call "Find_Number_LineMARVIN.vi"("Test Paragraph"="Motor Rotation Direction", "TableIn"=w361) -> ("Line number"=w358:i32)  [unwired: 3 in, 3 out]
                      n159 = And(x=w360, y=w359) -> (x .and. y?=w350:bool)
                      "VenableDirectionResult" <- w350
                      n160 = call "PassOrFail (SubVI).vi"("String Res"="", "index (row)"=w358, "Data in"=-3.0, "Pass?Fail"=w350, "Table in"=w361) -> ("error out"=w356:errorcluster)  [unwired: 6 in]
                      n161 = property class="Bool (strict)"(reference=w357, error in=w356) -> ("Value"=w373:bool)  [unwired: 2 out]
                      n162 = Select(t=T14."Stop", s=w373, f=T14."Stop") -> (s? t:f=w370:T14)
                    }
                    frame "FullSpeed2" {
                      n163 = Concatenate Strings(w397, "\nFull speed operation " ("string")) -> (w383:string)
                      n164 = Equal?(x=w382, y=u8 95) -> (x = y?=w392:bool)
                      n165 = Select(t=u16 15100, s=w392, f=u16 12100 ("y")) -> (s? t:f=w381:u16)
                      n166 = call "CANSendMotorSpeed.vi"("Remote"=TRUE, "Motor Speed RPM"=w381, "UUT"=w406, "CAN Cluster in"=w410) -> ("error out"=w404:errorcluster)  [unwired: 7 in]
                      n167 = call "Write panel message (SubVI).vi"("Stop BurnIn"=w384, 4:"rpm"=w402, 5:"rpm"=TRUE ("rpm"), "PrintTime"=FALSE, "Stop"=w386, "error in (no error)"=w404, "Time to wait"=0.2, "Strin"=w383, "String in"=w385) -> ("error out"=w389:errorcluster)  [unwired: 2 in]
                      n168 = property on="VenableSpeed" class="DigNum (strict)"("Value"=w381) -> ()  [unwired: 2 in, 2 out]
                      n169 = flat-sequence {
                        tunnel: w389 -> [w417]
                        tunnel: [w417] -> w388
                        tunnel: [w416] -> w387
                        frame #0 {
                          n170 = call <vilib>:"High Resolution Relative Seconds.vi"() -> ("relative seconds"=w416:dbl)
                        }
                      }
                      n171 = Select(t=14500.0, s=w392, f=11500.0) -> (s? t:f=w391:dbl)
                      n172 = Select(t=47.0, s=w392, f=24.0) -> (s? t:f=w390:dbl)
                      n173 = while {
                        tunnel: w402 -> [w419]
                        tunnel: w388 -> [w447]
                        tunnel: [w427] -> w399
                        tunnel: w391 -> [w440]
                        tunnel: w390 -> [w439]
                        tunnel: w387 -> [w435]
                        tunnel: w386 -> [w425]
                        tunnel: w385 -> [w426]
                        tunnel: w384 -> [w423]
                        tunnel: w383 -> [w422]
                        stop <- w437 stop-if-true
                        n174 = call <vilib>:"High Resolution Relative Seconds.vi"() -> ("relative seconds"=w436:dbl)
                        n175 = Subtract(x=w436, y=w435) -> (x-y=w434:dbl)
                        n176 = property class="DigNum (strict)"(reference=w419, error in=w447) -> (error out=w446:errorcluster, "Value"=w441:dbl)  [unwired: 1 out]
                        "FullSpeed2 Speed" <- w441
                        n177 = Greater Or Equal?(x=w434, y=120.0) -> (x >= y?=w432:bool)
                        n178 = Greater Or Equal?(x=w441, y=w440) -> (x >= y?=w431:bool)
                        n179 = property on="VISA Tester" class="VISAName"(error in=w446) -> (error out=w445:errorcluster, "Value"=w444:refnum<visa-resource-name>)  [unwired: 1 in, 1 out]
                        n180 = property class="Bool (strict)"(reference=w425) -> ("Value"=w430:bool)  [unwired: 1 in, 2 out]
                        n181 = call "GetADCTester (SubVI).vi"("error in (no error)"=w445, "GetADCTester"=T15."Current", "TimeToGet"=5, "VISA Refnum in"=w444) -> ("error out"=w442:errorcluster, "ADCValOutput Single"=w438:dbl)  [unwired: 5 in, 1 out]
                        "FullSpeed2 Current" <- w438
                        n182 = Greater Or Equal?(x=w438, y=w439) -> (x >= y?=w428:bool)
                        n183 = And(x=w431, y=w428) -> (x .and. y?=w429:bool)
                        n184 = Compound Arithmetic op=OR(w430, w432, w429) -> (w437:bool)
                        n185 = call "Write panel message (SubVI).vi"("Stop BurnIn"=w423, 4:"rpm"=w419, 5:"rpm"=TRUE ("rpm"), "PrintTime"=FALSE, "Stop"=w425, "error in (no error)"=w442, "Time to wait"=0.2, "Strin"=w422, "String in"=w426) -> ("error out"=w427:errorcluster)  [unwired: 2 in]
                      }
                      n186 = property class="Bool (strict)"(reference=w386, error in=w399) -> ("Value"=w415:bool)  [unwired: 2 out]
                      n187 = Select(t=T14."Stop", s=w415, f=T14."Result") -> (s? t:f=w412:T14)
                    }
                    frame "MD[1]=1" {
                      w448 = u16 0 ("Motor Speed RPM")
                      n188 = Concatenate Strings(w476, "\nSet Parameters MD[1]=1" ("Strin")) -> (w465:string)
                      n189 = property on="VISA Tester" class="VISAName"() -> ("Value"=w481:refnum<visa-resource-name>)  [unwired: 2 in, 2 out]
                      n190 = call "TesterOption (SubVI).vi"("2 Options"=FALSE, "On/Off"=FALSE, "Tester Option"=T13."Venable", "VISA Refnum in"=w481) -> ("error out"=w482:errorcluster, "VISA Refnum out"=w472:refnum<visa-resource-name>)  [unwired: 6 in]
                      n191 = call "CANSendMotorSpeed.vi"("Remote"=TRUE, "error in (no error)"=w482, "Motor Speed RPM"=w448, "UUT"=w466, "CAN Cluster in"=w486) -> ("error out"=w484:errorcluster)  [unwired: 6 in]
                      n192 = call "Write panel message (SubVI).vi"("Stop BurnIn"=w467, 4:"rpm"=w455, 5:"rpm"=FALSE ("rpm"), "PrintTime"=TRUE, "Stop"=w457, "error in (no error)"=w484, "Time to wait"=20.0, "Strin"=w465, "String in"=w468) -> ("error out"=w454:errorcluster)  [unwired: 2 in]
                      n193 = property on="VenableSpeed" class="DigNum (strict)"("Value"=w448) -> ()  [unwired: 2 in, 2 out]
                      n194 = property on="VISA Marvin" class="VISAName"(error in=w454) -> (error out=w483:errorcluster, "Value"=w488:refnum<visa-resource-name>)  [unwired: 1 in, 1 out]
                      n195 = call "SerialMarvinSendGet.vi"("error in (no error)"=w483, "Clear Log"=FALSE, "write buffer"="EP=1\r\nMD[1]=1\r\n", "VISA resource name"=w488) -> ("error out"=w471:errorcluster)  [unwired: 6 in, 1 out]
                      n196 = call "TesterOption (SubVI).vi"("2 Options"=FALSE, "error in (no error)"=w471, "On/Off"=FALSE, "Tester Option"=T13."Power", "VISA Refnum in"=w472) -> ("error out"=w469:errorcluster, "VISA Refnum out"=w458:refnum<visa-resource-name>)  [unwired: 5 in]
                      n197 = call "Write panel message (SubVI).vi"("Stop BurnIn"=w467, 4:"rpm"=w455, 5:"rpm"=FALSE ("rpm"), "PrintTime"=TRUE, "Stop"=w457, "error in (no error)"=w469, "Time to wait"=25.0, "Strin"=w465, "String in"=w468) -> ("error out"=w459:errorcluster)  [unwired: 2 in]
                      n198 = call "TesterOption (SubVI).vi"("2 Options"=FALSE, "error in (no error)"=w459, "On/Off"=TRUE, "Tester Option"=T13."Venable", "VISA Refnum in"=w458) -> ("error out"=w456:errorcluster)  [unwired: 5 in, 1 out]
                      n199 = call "Time Delay8"("error in (no error)"=w456) -> ("error out"=w452:errorcluster)  [unwired: 10 in]
                      n200 = property class="Bool (strict)"(reference=w457, error in=w452) -> ("Value"=w493:bool)  [unwired: 2 out]
                      n201 = Select(t=T14."Stop", s=w493, f=T14."FullSpeed2") -> (s? t:f=w492:T14)
                    }
                    frame "FullSpeed1" {
                      n202 = Concatenate Strings(w514, "\nFull speed operation " ("string")) -> (w499:string)
                      n203 = Equal?(x=w495, y=u8 95) -> (x = y?=w512:bool)
                      n204 = flat-sequence {
                        tunnel: w505 -> [w530]
                        tunnel: [w530] -> w504
                        tunnel: [w529] -> w503
                        frame #0 {
                          n205 = call <vilib>:"High Resolution Relative Seconds.vi"() -> ("relative seconds"=w529:dbl)
                        }
                      }
                      n206 = Select(t=u16 15100, s=w512, f=u16 12100 ("y")) -> (s? t:f=w494:u16)
                      n207 = call "CANSendMotorSpeed.vi"("Remote"=TRUE, "Motor Speed RPM"=w494, "UUT"=w519, "CAN Cluster in"=w523) -> ("error out"=w517:errorcluster)  [unwired: 7 in]
                      n208 = call "Write panel message (SubVI).vi"("Stop BurnIn"=w500, 4:"rpm"=w516, 5:"rpm"=TRUE ("rpm"), "PrintTime"=FALSE, "Stop"=w502, "error in (no error)"=w517, "Time to wait"=0.2, "Strin"=w499, "String in"=w501) -> ("error out"=w505:errorcluster)  [unwired: 2 in]
                      n209 = Select(t=13700.0, s=w512, f=11500.0) -> (s? t:f=w507:dbl)
                      n210 = Select(t=56.0, s=w512, f=33.0) -> (s? t:f=w506:dbl)
                      n211 = while {
                        tunnel: w516 -> [w532]
                        tunnel: w504 -> [w560]
                        tunnel: [w540] -> w515
                        tunnel: w507 -> [w552]
                        tunnel: w506 -> [w549]
                        tunnel: w503 -> [w547]
                        tunnel: w502 -> [w538]
                        tunnel: w501 -> [w539]
                        tunnel: w500 -> [w536]
                        tunnel: w499 -> [w535]
                        stop <- w554 stop-if-true
                        n212 = property class="DigNum (strict)"(reference=w532, error in=w560) -> (error out=w559:errorcluster, "Value"=w553:dbl)  [unwired: 1 out]
                        "FullSpeed1 Speed" <- w553
                        n213 = call <vilib>:"High Resolution Relative Seconds.vi"() -> ("relative seconds"=w548:dbl)
                        n214 = Subtract(x=w548, y=w547) -> (x-y=w546:dbl)
                        n215 = Greater Or Equal?(x=w546, y=120.0) -> (x >= y?=w544:bool)
                        n216 = Greater Or Equal?(x=w553, y=w552) -> (x >= y?=w551:bool)
                        n217 = property on="VISA Tester" class="VISAName"(error in=w559) -> (error out=w558:errorcluster, "Value"=w557:refnum<visa-resource-name>)  [unwired: 1 in, 1 out]
                        n218 = call "GetADCTester (SubVI).vi"("error in (no error)"=w558, "GetADCTester"=T15."Current", "TimeToGet"=5, "VISA Refnum in"=w557) -> ("error out"=w555:errorcluster, "ADCValOutput Single"=w550:dbl)  [unwired: 5 in, 1 out]
                        "FullSpeed1 Current" <- w550
                        n219 = Greater Or Equal?(x=w550, y=w549) -> (x >= y?=w541:bool)
                        n220 = And(x=w541, y=w551) -> (x .and. y?=w542:bool)
                        n221 = property class="Bool (strict)"(reference=w538) -> ("Value"=w543:bool)  [unwired: 1 in, 2 out]
                        n222 = call "Write panel message (SubVI).vi"("Stop BurnIn"=w536, 4:"rpm"=w532, 5:"rpm"=TRUE ("rpm"), "PrintTime"=FALSE, "Stop"=w538, "error in (no error)"=w555, "Time to wait"=0.2, "Strin"=w535, "String in"=w539) -> ("error out"=w540:errorcluster)  [unwired: 2 in]
                        n223 = Compound Arithmetic op=OR(w543, w542, w544) -> (w554:bool)
                      }
                      n224 = property on="VenableSpeed" class="DigNum (strict)"("Value"=w494) -> ()  [unwired: 2 in, 2 out]
                      n225 = property class="Bool (strict)"(reference=w502, error in=w515) -> ("Value"=w528:bool)  [unwired: 2 out]
                      n226 = Select(t=T14."Stop", s=w528, f=T14."MD[1]=1") -> (s? t:f=w525:T14)
                    }
                    frame "MD[1]=0" {
                      w561 = u16 0 ("Motor Speed RPM")
                      n227 = Concatenate Strings(w588, "\nSet Parameters MD[1]=0" ("Strin")) -> (w577:string)
                      n228 = property on="VISA Tester" class="VISAName"() -> ("Value"=w594:refnum<visa-resource-name>)  [unwired: 2 in, 2 out]
                      n229 = call "TesterOption (SubVI).vi"("2 Options"=FALSE, "On/Off"=FALSE, "Tester Option"=T13."Venable", "VISA Refnum in"=w594) -> ("error out"=w595:errorcluster, "VISA Refnum out"=w584:refnum<visa-resource-name>)  [unwired: 6 in]
                      n230 = call "CANSendMotorSpeed.vi"("Remote"=TRUE, "error in (no error)"=w595, "Motor Speed RPM"=w561, "UUT"=w578, "CAN Cluster in"=w599) -> ("error out"=w597:errorcluster)  [unwired: 6 in]
                      n231 = call "Write panel message (SubVI).vi"("Stop BurnIn"=w579, 4:"rpm"=w574, 5:"rpm"=FALSE ("rpm"), "PrintTime"=FALSE, "Stop"=w568, "error in (no error)"=w597, "Time to wait"=0.2, "Strin"=w577, "String in"=w580) -> ("error out"=w591:errorcluster)  [unwired: 2 in]
                      n232 = property on="VenableSpeed" class="DigNum (strict)"("Value"=w561) -> ()  [unwired: 2 in, 2 out]
                      n233 = property on="VISA Marvin" class="VISAName"(error in=w591) -> (error out=w596:errorcluster, "Value"=w601:refnum<visa-resource-name>)  [unwired: 1 in, 1 out]
                      n234 = call "SerialMarvinSendGet.vi"("error in (no error)"=w596, "Clear Log"=FALSE, "write buffer"="EP=1\r\nMD[1]=0\r\n", "VISA resource name"=w601) -> ("error out"=w583:errorcluster)  [unwired: 6 in, 1 out]
                      n235 = call "TesterOption (SubVI).vi"("2 Options"=FALSE, "error in (no error)"=w583, "On/Off"=FALSE, "Tester Option"=T13."Power", "VISA Refnum in"=w584) -> ("error out"=w581:errorcluster, "VISA Refnum out"=w569:refnum<visa-resource-name>)  [unwired: 5 in]
                      n236 = call "Write panel message (SubVI).vi"("Stop BurnIn"=w579, 4:"rpm"=w574, 5:"rpm"=FALSE ("rpm"), "PrintTime"=TRUE, "Stop"=w568, "error in (no error)"=w581, "Time to wait"=25.0, "Strin"=w577, "String in"=w580) -> ("error out"=w570:errorcluster)  [unwired: 2 in]
                      n237 = call "TesterOption (SubVI).vi"("2 Options"=FALSE, "error in (no error)"=w570, "On/Off"=TRUE, "Tester Option"=T13."Venable", "VISA Refnum in"=w569) -> ("error out"=w567:errorcluster)  [unwired: 5 in, 1 out]
                      n238 = call "Time Delay4"("error in (no error)"=w567) -> ("error out"=w563:errorcluster)  [unwired: 10 in]
                      n239 = property class="Bool (strict)"(reference=w568, error in=w563) -> ("Value"=w606:bool)  [unwired: 2 out]
                      n240 = Select(t=T14."Stop", s=w606, f=T14."FullSpeed1") -> (s? t:f=w605:T14)
                    }
                  }
                }
                n241 = flat-sequence {
                  tunnel: [enum16{"Stop", "Direction", "Venable", "Start"}."Stop"] -> w325
                  tunnel: w324 -> [_]
                  frame #0 {
                  }
                }
              }
              frame "Venable" {
                n242 = call "Find_Number_LineMARVIN.vi"("Test Paragraph"="Enable Test", "TableIn"=w611) -> ("Line number"=w619:i32)  [unwired: 3 in, 3 out]
                n243 = Increment(x=w619) -> (x+1=w607:i32)
                n244 = for {
                  tunnel: u16[] [5000, 0, 5000] -> [w649] mode=indexing
                  tunnel: bool[] [TRUE, FALSE, TRUE] -> [w645] mode=indexing
                  tunnel: w607 -> [w650]
                  tunnel: w618 -> [w648]
                  tunnel: w617 -> [w647]
                  tunnel: w616 -> [w636]
                  tunnel: w615 -> [w640]
                  tunnel: w613 -> [w639]
                  tunnel: w614 -> [w638]
                  tunnel: w611 -> [w632]
                  tunnel: w610 -> [w630]
                  tunnel: [w629] -> w609 mode=indexing
                  i -> [w651]
                  w627 = u16 5000 ("Motor Speed RPM")
                  w653 = 200.0 ("y")
                  n245 = call "CANSendMotorSpeed.vi"("Remote"=TRUE, "Motor Speed RPM"=w627, "UUT"=w647, "CAN Cluster in"=w648) -> ("error out"=w644:errorcluster)  [unwired: 7 in]
                  n246 = property on="VISA Tester" class="VISAName"() -> ("Value"=w643:refnum<visa-resource-name>)  [unwired: 2 in, 2 out]
                  n247 = Add(x=w650, y=w651) -> (x+y=w633:i32)
                  n248 = call "TesterOption (SubVI).vi"("2 Options"=FALSE, "error in (no error)"=w644, "On/Off"=w645, "Tester Option"=T13."Venable", "VISA Refnum in"=w643) -> ("error out"=w642:errorcluster)  [unwired: 5 in, 1 out]
                  n249 = call "Write panel message (SubVI).vi"("Stop BurnIn"=w638, 4:"rpm"=w636, 5:"rpm"=TRUE ("rpm"), "PrintTime"=TRUE, "Stop"=w639, "error in (no error)"=w642, "Time to wait"=15.0, "Strin"=w630, "String in"=w640) -> ("error out"=w641:errorcluster)  [unwired: 2 in]
                  n250 = property class="DigNum (strict)"(reference=w636, error in=w641) -> ("Value"=w631:dbl)  [unwired: 2 out]
                  n251 = Add(x=w649, y=w653) -> (x+y=w655:dbl)
                  n252 = Subtract(x=w649, y=w653) -> (x-y=w654:dbl)
                  n253 = In Range and Coerce(upper limit=w655, x=w631, lower limit=w654) -> (In Range?=w629:bool)  [unwired: 1 out]
                  n254 = call "PassOrFail (SubVI).vi"("index (row)"=w633, "Data in"=w631, "Pass?Fail"=w629, "Table in"=w632) -> ()  [unwired: 7 in, 1 out]
                  "VenableSpeed" <- w627
                }
                n255 = property class="Bool (strict)"(reference=w613) -> ("Value"=w626:bool)  [unwired: 1 in, 2 out]
                n256 = And Array Elements(Boolean array=w609) -> (logical AND=→"VenableResult":bool)
                n257 = Select(t=enum16{"Stop", "Direction", "Venable", "Start"}."Stop", s=w626, f=enum16{"Stop", "Direction", "Venable", "Start"}."Direction") -> (s? t:f=w612:enum16{"Stop", "Direction", "Venable", "Start"})
              }
              frame "Start" {
                w675 = "Enable Test" ("Test Paragraph")
                n258 = property class="Str"(reference=w666, "Value"=w657) -> (reference out=w676:refnum<vi>, error out=w663:errorcluster)  [unwired: 1 in]
                n259 = call "Table_ScrollaBarMarvin.vi"("error in"=w663, "Line to focus"=w675, "reference in"=w667) -> ("error out"=w672:errorcluster)  [unwired: 2 out]
                n260 = call "Reset old test Values (SubVI).vi"("error in"=w672, "Atr in"=w667, "Test Paragraph"=w675) -> ("error out"=w671:errorcluster)  [unwired: 8 in]
                n261 = property on="VISA Tester" class="VISAName"(error in=w671) -> (error out=w670:errorcluster, "Value"=w669:refnum<visa-resource-name>)  [unwired: 1 in, 1 out]
                n262 = property class="Bool (strict)"(reference=w660) -> ("Value"=w680:bool)  [unwired: 1 in, 2 out]
                n263 = call "TesterOption (SubVI).vi"("2 Options"=FALSE, "error in (no error)"=w670, "On/Off"=TRUE, "Tester Option"=T13."Venable", "VISA Refnum in"=w669) -> ("error out"=w668:errorcluster)  [unwired: 5 in, 1 out]
                n264 = Select(t=enum16{"Stop", "Direction", "Venable", "Start"}."Stop", s=w680, f=enum16{"Stop", "Direction", "Venable", "Start"}."Venable") -> (s? t:f=w664:enum16{"Stop", "Direction", "Venable", "Start"})
                n265 = call "Write panel message (SubVI).vi"("Stop BurnIn"=w659, 4:"rpm"=w658, 5:"rpm"=FALSE ("rpm"), "PrintTime"=FALSE, "Stop"=w660, "error in (no error)"=w668, "Time to wait"=0.2, "Strin"=w657, "String in"=w676) -> ()  [unwired: 2 in, 1 out]
              }
            }
          }
        }
        frame "Speed Command" {
          w685 = "Speed Command Test in process..." ("Value")
          w682 = "Speed Command Test" ("Test Paragraph")
          n266 = control-ref of="Pannel User Message"() -> (w697:refnum<vi>)
          n267 = property class="Str"(reference=w697, error in=w696, "Value"=w685) -> (error out=w695:errorcluster)  [unwired: 1 out]
          n268 = call "Table_ScrollaBarMarvin.vi"("error in"=w695, "Line to focus"=w682, "reference in"=w681) -> ("error out"=w698:errorcluster)  [unwired: 2 out]
          n269 = property class="Tbl (strict)"(reference=w681, error in=w698) -> (error out=w700:errorcluster, "Value"=w701:string[][])  [unwired: 1 out]
          n270 = Index Array(array=w701, index (col)=1 ("disabled index (col)")) -> (element=w702:string[])  [unwired: 1 in]
          n271 = call "Find_Number_Line.vi"("error in"=w700, "Test Paragraph"=w682, "Row Headers[]"=w702) -> ("error out"=w683:errorcluster, "Line number"=w686:i32)  [unwired: 1 out]
          n272 = call "Reset old test Values (SubVI).vi"("error in"=w683, "Atr in"=w681, "Test Paragraph"=w682) -> ()  [unwired: 8 in, 1 out]
          n273 = control-ref of="Pannel User Message"() -> (w690:refnum<vi>)
          n274 = control-ref of="Stop Burn-in"() -> (w694:refnum<vi>)
          n275 = control-ref of="Config_CANAT"() -> (w691:refnum<vi>)
          n276 = control-ref of="Motor Speed RPM"() -> (w692:refnum<vi>)
          n277 = control-ref of="UUT"() -> (w693:refnum<vi>)
          n278 = control-ref of="Stop Button"() -> (w688:refnum<vi>)
          n279 = control-ref of="ATR"() -> (w689:refnum<vi>)
          n280 = property on="UUT" class="DigNum (strict)"() -> ("Value"=w684:u8)  [unwired: 2 in, 2 out]
          n281 = while {
            shift-right: [w714] -> _
            shift-left: enum16{"Stop", "StopTime", "Speeds", "Start"}."Start" -> [w715]
            tunnel: w688 -> [w713]
            tunnel: w689 -> [w712]
            tunnel: w690 -> [w711]
            tunnel: w691 -> [w710]
            tunnel: w692 -> [w709]
            tunnel: w693 -> [w708]
            tunnel: w694 -> [w707]
            tunnel: w686 -> [w706]
            tunnel: w685 -> [w705]
            tunnel: w684 -> [w703]
            stop <- w704 stop-if-true
            n282 = case shown="\"Speeds\"" w715 {
              tunnel: [w719 w749 w789 w833] -> w714
              tunnel: w713 -> [_ w744 w793 w831]
              tunnel: w712 -> [_ w734 w797 _]
              tunnel: w711 -> [_ w745 w794 _]
              tunnel: w710 -> [w717 w747 w796 _]
              tunnel: w709 -> [_ w742 w791 _]
              tunnel: w708 -> [w718 w746 w788 _]
              tunnel: w707 -> [_ w743 w792 _]
              tunnel: w706 -> [_ _ w798 _]
              tunnel: w705 -> [_ _ w795 _]
              tunnel: [w716 w748 w790 FALSE ("Value")] -> w704
              tunnel: w703 -> [_ _ w781 _]
              frame "Stop", Default {
                n283 = flat-sequence {
                  tunnel: w718 -> [w723]
                  tunnel: w717 -> [w722]
                  tunnel: [enum16{"Stop", "StopTime", "Speeds", "Start"}."Stop"] -> w719
                  tunnel: [TRUE] -> w716
                  frame #0 {
                    w720 = u16 0 ("Motor Speed RPM")
                    n284 = call "CANSendMotorSpeed.vi"("Remote"=TRUE, "Motor Speed RPM"=w720, "UUT"=w723, "CAN Cluster in"=w722) -> ("error out"=w727:errorcluster)  [unwired: 7 in]
                    n285 = property on="SpeedCommandSpeed" class="DigNum (strict)"("Value"=w720) -> ()  [unwired: 2 in, 2 out]
                    n286 = property on="VISA Tester" class="VISAName"() -> ("Value"=w728:refnum<visa-resource-name>)  [unwired: 2 in, 2 out]
                    n287 = call "TesterOption (SubVI).vi"("2 Options"=FALSE, "error in (no error)"=w727, "On/Off"=FALSE, "Tester Option"=T13."Venable", "VISA Refnum in"=w728) -> ()  [unwired: 5 in, 2 out]
                  }
                  frame #1 {
                  }
                }
              }
              frame "StopTime" {
                w731 = u16 0 ("Motor Speed RPM")
                n288 = call "Table_ScrollaBarMarvin.vi"("Line to focus"="Motor Stop time", "reference in"=w734) -> ("error out"=w735:errorcluster)  [unwired: 1 in, 2 out]
                n289 = property on="SpeedCommandSpeed" class="DigNum (strict)"("Value"=w731) -> ()  [unwired: 2 in, 2 out]
                n290 = call "CANSendMotorSpeed.vi"("Remote"=TRUE, "error in (no error)"=w735, "Motor Speed RPM"=w731, "UUT"=w746, "CAN Cluster in"=w747) -> ("error out"=w752:errorcluster)  [unwired: 6 in]
                n291 = flat-sequence {
                  tunnel: [w778] -> w751
                  tunnel: w752 -> [w777]
                  tunnel: [w777] -> w753
                  frame #0 {
                    n292 = call <vilib>:"High Resolution Relative Seconds.vi"() -> ("relative seconds"=w778:dbl)
                  }
                }
                n293 = while {
                  tunnel: [w773] -> w748
                  tunnel: w745 -> [w771]
                  tunnel: w744 -> [w770]
                  tunnel: w743 -> [w768]
                  tunnel: w742 -> [w767]
                  tunnel: "Stop Time Test in process..." ("Value") -> [w755]
                  tunnel: [w763] -> w732
                  tunnel: w753 -> [w775]
                  tunnel: [w764] -> w740
                  tunnel: w751 -> [w774]
                  tunnel: [w762] -> w736
                  stop <- w754 stop-if-true
                  n294 = call "Write panel message (SubVI).vi"("Stop BurnIn"=w768, 4:"rpm"=w767, 5:"rpm"=TRUE ("rpm"), "PrintTime"=FALSE, "Stop"=w770, "error in (no error)"=w775, "Time to wait"=0.1, "Strin"=w755, "String in"=w771) -> ("error out"=w772:errorcluster)  [unwired: 2 in]
                  n295 = control-ref of="Motor Speed RPM"() -> (w761:refnum<vi>)
                  n296 = property class="DigNum (strict)"(reference=w761, error in=w772) -> (error out=w764:errorcluster, "Value"=w760:dbl)  [unwired: 1 out]
                  n297 = call <vilib>:"High Resolution Relative Seconds.vi"() -> ("relative seconds"=w758:dbl)
                  n298 = property class="Bool (strict)"(reference=w770) -> ("Value"=w773:bool)  [unwired: 1 in, 2 out]
                  n299 = Subtract(x=w758, y=w774) -> (x-y=w762:dbl)
                  n300 = Greater Or Equal?(x=w762, y=50.0) -> (x >= y?=w756:bool)
                  n301 = Less Or Equal?(x=w760, y=0.0) -> (x <= y?=w763:bool)
                  n302 = Compound Arithmetic op=OR(w763, w756, w773) -> (w754:bool)
                }
                "StopTimeResult" <- w732
                n303 = call "Find_Number_LineMARVIN.vi"("Test Paragraph"="Motor Stop time", "TableIn"=w734) -> ("Line number"=w737:i32)  [unwired: 3 in, 3 out]
                n304 = call "PassOrFail (SubVI).vi"("index (row)"=w737, "error in (no error)"=w740, "Data in"=w736, "Pass?Fail"=w732, "Table in"=w734) -> ("error out"=w739:errorcluster)  [unwired: 6 in]
                n305 = flat-sequence {
                  tunnel: [enum16{"Stop", "StopTime", "Speeds", "Start"}."Stop"] -> w749
                  tunnel: w739 -> [_]
                  frame #0 {
                  }
                }
              }
              frame "Speeds" {
                n306 = Equal?(x=w781, y=u8 95) -> (x = y?=w786:bool)
                n307 = Select(t=u16[] [11500, 12700, 14700], s=w786, f=u16[] [6000, 9000, 12100]) -> (s? t:f=w783:u16[])
                n308 = for {
                  tunnel: w783 -> [w824] mode=indexing
                  tunnel: w798 -> [w817]
                  tunnel: w797 -> [w816]
                  tunnel: w788 -> [w815]
                  tunnel: w796 -> [w814]
                  tunnel: w795 -> [w813]
                  tunnel: w794 -> [w812]
                  tunnel: w793 -> [w811]
                  tunnel: w792 -> [w809]
                  tunnel: w791 -> [w807]
                  tunnel: [w805] -> w790
                  tunnel: [w804] -> w782
                  tunnel: [w803] -> w780 mode=indexing
                  i -> [w823]
                  stop <- w805 stop-if-true
                  w825 = 200.0 ("y")
                  n309 = Increment(x=w823) -> (x+1=w822:i32)
                  n310 = Add(x=w817, y=w822) -> (x+y=w818:i32)
                  n311 = call "CANSendMotorSpeed.vi"("Remote"=TRUE, "Motor Speed RPM"=w824, "UUT"=w815, "CAN Cluster in"=w814) -> ("error out"=w829:errorcluster)  [unwired: 7 in]
                  n312 = control-ref of="Motor Speed RPM"() -> (w830:refnum<vi>)
                  n313 = call "Write panel message (SubVI).vi"("Stop BurnIn"=w809, 4:"rpm"=w807, 5:"rpm"=TRUE ("rpm"), "PrintTime"=TRUE, "Stop"=w811, "error in (no error)"=w829, "Time to wait"=30.0 ("Delay Time (sec)"), "Strin"=w813, "String in"=w812) -> ("error out"=w821:errorcluster)  [unwired: 2 in]
                  n314 = property class="DigNum (strict)"(reference=w830, error in=w821) -> (error out=w828:errorcluster, "Value"=w806:dbl)  [unwired: 1 out]
                  n315 = property class="Bool (strict)"(reference=w811) -> ("Value"=w805:bool)  [unwired: 1 in, 2 out]
                  n316 = Add(x=w824, y=w825) -> (x+y=w827:dbl)
                  n317 = Subtract(x=w824, y=w825) -> (x-y=w826:dbl)
                  n318 = In Range and Coerce(upper limit=w827, x=w806, lower limit=w826) -> (In Range?=w803:bool)  [unwired: 1 out]
                  n319 = call "PassOrFail (SubVI).vi"("index (row)"=w818, "error in (no error)"=w828, "Data in"=w806, "Pass?Fail"=w803, "Table in"=w816) -> ("error out"=w804:errorcluster)  [unwired: 6 in]
                  "SpeedCommandSpeed" <- w824
                }
                n320 = flat-sequence {
                  tunnel: w790 -> [w802]
                  tunnel: [w800] -> w789
                  tunnel: w782 -> [_]
                  frame #0 {
                    n321 = Select(t=enum16{"Stop", "StopTime", "Speeds", "Start"}."Stop", s=w802, f=enum16{"Stop", "StopTime", "Speeds", "Start"}."StopTime") -> (s? t:f=w800:enum16{"Stop", "StopTime", "Speeds", "Start"})
                  }
                }
                n322 = And Array Elements(Boolean array=w780) -> (logical AND=→"SpeedResult":bool)
              }
              frame "Start" {
                n323 = property on="VISA Tester" class="VISAName"() -> ("Value"=w841:refnum<visa-resource-name>)  [unwired: 2 in, 2 out]
                n324 = call "TesterOption (SubVI).vi"("2 Options"=FALSE, "On/Off"=TRUE, "Tester Option"=T13."Venable", "VISA Refnum in"=w841) -> ("error out"=w832:errorcluster)  [unwired: 6 in, 1 out]
                n325 = property class="Bool (strict)"(reference=w831, error in=w832) -> ("Value"=w837:bool)  [unwired: 2 out]
                n326 = Select(t=enum16{"Stop", "StopTime", "Speeds", "Start"}."Stop", s=w837, f=enum16{"Stop", "StopTime", "Speeds", "Start"}."Speeds") -> (s? t:f=w833:enum16{"Stop", "StopTime", "Speeds", "Start"})
              }
            }
          }
        }
        frame "Stop Time" {
          w845 = "Motor Temperature test in process..." ("Value")
          w843 = "Motor Termistor Input Test" ("Test Paragraph")
          n327 = control-ref of="Pannel User Message"() -> (w853:refnum<vi>)
          n328 = property class="Str"(reference=w853, error in=w852, "Value"=w845) -> (error out=w851:errorcluster)  [unwired: 1 out]
          n329 = call "Table_ScrollaBarMarvin.vi"("error in"=w851, "Line to focus"=w843, "reference in"=w842) -> ("error out"=w855:errorcluster)  [unwired: 2 out]
          n330 = property class="Tbl (strict)"(reference=w842, error in=w855) -> (reference out=w848:refnum<vi>, error out=w857:errorcluster, "Value"=w858:string[][])
          n331 = Index Array(array=w858, index (col)=1 ("disabled index (col)")) -> (element=w859:string[])  [unwired: 1 in]
          n332 = call "Find_Number_LineMARVIN.vi"("Test Paragraph"=w843, "error in"=w857, "TableIn"=w842, "Row Headers[]"=w859) -> ("error out"=w854:errorcluster, "Line number"=w847:i32)  [unwired: 1 in, 2 out]
          n333 = call "Reset old test Values (SubVI).vi"("error in"=w854, "Atr in"=w842, "Test Paragraph"=w843) -> ("error out"=w844:errorcluster)  [unwired: 8 in]
          n334 = property on="Status" class="Bool (strict)"(error in=w844) -> (error out=w849:errorcluster, "Value"=w850:bool)  [unwired: 1 in, 1 out]
          n335 = case shown="True" w850 {
            selector: w850 -> [w863 _]
            tunnel: w849 -> [w865 _]
            tunnel: w848 -> [w862 _]
            tunnel: w847 -> [w861 w868]
            tunnel: w846 -> [_ w873]
            tunnel: w845 -> [_ w869]
            frame False {
              n336 = flat-sequence {
                tunnel: w865 -> [w866]
                tunnel: [w866] -> w864
                frame #0 {
                  n337 = One Button Dialog(message="Please establish RS connection.") -> ()  [unwired: 1 in, 1 out]
                }
              }
              n338 = Increment(x=w861) -> (x+1=w860:i32)
              n339 = call "PassOrFail (SubVI).vi"("index (row)"=w860, "error in (no error)"=w864, "Pass?Fail"=w863, "Table in"=w862) -> ()  [unwired: 7 in, 1 out]
            }
            frame True {
              n340 = control-ref of="Stop Burn-in"() -> (w875:refnum<vi>)
              n341 = control-ref of="Pannel User Message"() -> (w877:refnum<vi>)
              n342 = control-ref of="Config_CANAT"() -> (w871:refnum<vi>)
              n343 = control-ref of="ATR"() -> (w878:refnum<vi>)
              n344 = control-ref of="Motor Speed RPM"() -> (w879:refnum<vi>)
              n345 = control-ref of="UUT"() -> (w870:refnum<vi>)
              n346 = control-ref of="Stop Button"() -> (w876:refnum<vi>)
              n347 = property on="VISA Tester" class="VISAName"() -> ("Value"=w872:refnum<visa-resource-name>)  [unwired: 2 in, 2 out]
              n348 = while {
                shift-right: [w883] -> _
                shift-left: T16."Start" -> [w893]
                tunnel: w875 -> [w892]
                tunnel: w876 -> [w891]
                tunnel: w877 -> [w890]
                tunnel: w878 -> [w889]
                tunnel: w879 -> [w888]
                tunnel: w873 -> [w887]
                tunnel: w872 -> [w886]
                tunnel: w871 -> [w885]
                tunnel: w870 -> [w884]
                tunnel: w869 -> [w881]
                tunnel: w868 -> [w880]
                stop <- w882 stop-if-true
                n349 = case shown="\"Start\"" w893 {
                  tunnel: w892 -> [_ w916 w975]
                  tunnel: w891 -> [_ w908 w977]
                  tunnel: w890 -> [_ w917 w979]
                  tunnel: w889 -> [_ w906 _]
                  tunnel: w888 -> [_ w915 w974]
                  tunnel: w887 -> [_ w920 _]
                  tunnel: w886 -> [w896 w919 w968]
                  tunnel: w885 -> [_ _ w985]
                  tunnel: w884 -> [_ _ w984]
                  tunnel: [w894 w909 w970] -> w883
                  tunnel: [w895 FALSE FALSE] -> w882
                  tunnel: w881 -> [_ w918 _]
                  tunnel: w880 -> [_ w905 _]
                  frame "Stop", Default {
                    n350 = flat-sequence {
                      tunnel: w896 -> [w897]
                      tunnel: [TRUE] -> w895
                      tunnel: [T16."Stop"] -> w894
                      frame #0 {
                        n351 = call "TesterOption (SubVI).vi"("2 Options"=FALSE, "On/Off"=FALSE, "Tester Option"=T13."Venable", "VISA Refnum in"=w897) -> ()  [unwired: 6 in, 2 out]
                      }
                      frame #1 {
                      }
                    }
                  }
                  frame "TA[5]" {
                    w921 = T19 [enum."60C", enum."90C", enum."120C"] items=["K15", "K16", "K17", "Venable", "Firmeware", "Fan", "Power", "120C", "110C", "100C", "90C", "80C", "70C", "60C", "50C", "40C", "30C", "25C", "20C", "10C", "0C"]
                    n352 = for {
                      tunnel: w921 -> [w945] mode=indexing
                      tunnel: w920 -> [w944]
                      tunnel: w919 -> [w943]
                      tunnel: w918 -> [w942]
                      tunnel: w917 -> [w941]
                      tunnel: w908 -> [w940]
                      tunnel: w916 -> [w939]
                      tunnel: w915 -> [w938]
                      tunnel: dbl[] [60.0, 90.0, 120.0] -> [w928] mode=indexing
                      tunnel: [w927] -> w907
                      tunnel: w906 -> [w934]
                      tunnel: w905 -> [w933]
                      tunnel: [w922] -> w904 mode=indexing
                      i -> [w931]
                      w926 = 3.0 ("y")
                      n353 = for {
                        N: 5 -> [_]
                        tunnel: w945 -> [w947]
                        tunnel: w944 -> [w963]
                        tunnel: w943 -> [w959]
                        tunnel: w942 -> [w957]
                        tunnel: w941 -> [w956]
                        tunnel: w940 -> [w955]
                        tunnel: w939 -> [w953]
                        tunnel: w938 -> [w950]
                        tunnel: [w949] -> w937 mode=indexing
                        tunnel: [w948] -> w935
                        n354 = call "TesterOption (SubVI).vi"("2 Options"=FALSE, "On/Off"=TRUE, "Tester Option"=w947, "VISA Refnum in"=w959) -> ("error out"=w960:errorcluster)  [unwired: 6 in, 1 out]
                        n355 = call "Write panel message (SubVI).vi"("Stop BurnIn"=w953, 4:"rpm"=w950, 5:"rpm"=FALSE ("rpm"), "PrintTime"=FALSE, "Stop"=w955, "error in (no error)"=w960, "Time to wait"=1.0, "Strin"=w957, "String in"=w956) -> ("error out"=w958:errorcluster)  [unwired: 2 in]
                        n356 = call "SerialMarvinSendGet.vi"("error in (no error)"=w958, "write buffer"="TA[2]\r\n", "VISA resource name"=w963) -> ("error out"=w948:errorcluster, "read buffer"=w961:string)  [unwired: 7 in]
                        n357 = Fract/Exp String To Number(string=w961) -> (number=w949:dbl)  [unwired: 3 in, 1 out]
                      }
                      n358 = Increment(x=w931) -> (x+1=w930:i32)
                      n359 = Add Array Elements(numeric array=w937) -> (sum=w936:dbl)
                      n360 = Add(x=w928, y=w926) -> (x+y=w925:dbl)
                      n361 = Subtract(x=w928, y=w926) -> (x-y=w924:dbl)
                      n362 = Divide(x=w936, y=5.0) -> (x/y=w923:dbl)
                      n363 = In Range and Coerce(upper limit=w925, x=w923, lower limit=w924) -> (In Range?=w922:bool)  [unwired: 1 out]
                      n364 = Add(x=w933, y=w930) -> (x+y=w932:i32)
                      n365 = call "PassOrFail (SubVI).vi"("index (row)"=w932, "error in (no error)"=w935, "Data in"=w923, "Pass?Fail"=w922, "Table in"=w934) -> ("error out"=w927:errorcluster)  [unwired: 6 in]
                    }
                    n366 = property class="Bool (strict)"(reference=w908, error in=w907) -> ("Value"=w913:bool)  [unwired: 2 out]
                    n367 = Select(t=T16."Stop", s=w913, f=T16."Stop") -> (s? t:f=w909:T16)
                    n368 = And Array Elements(Boolean array=w904) -> (logical AND=→"MotorTempResult":bool)
                  }
                  frame "Start" {
                    n369 = call "Write panel message (SubVI).vi"("Stop BurnIn"=w975, 4:"rpm"=w974, 5:"rpm"=FALSE ("rpm"), "PrintTime"=FALSE, "Stop"=w977, "Time to wait"=0.1, "Strin"="Motor Temperature test in process...\nInitialization state...", "String in"=w979) -> ("error out"=w980:errorcluster)  [unwired: 3 in]
                    n370 = call "TesterOption (SubVI).vi"("2 Options"=FALSE, "error in (no error)"=w980, "On/Off"=FALSE, "Tester Option"=T13."Venable", "VISA Refnum in"=w968) -> ("error out"=w982:errorcluster)  [unwired: 5 in, 1 out]
                    n371 = call "CANSendMotorSpeed.vi"("Remote"=TRUE, "error in (no error)"=w982, "Motor Speed RPM"=u16 0, "UUT"=w984, "CAN Cluster in"=w985) -> ("error out"=w967:errorcluster)  [unwired: 6 in]
                    n372 = property class="Bool (strict)"(reference=w977, error in=w967) -> ("Value"=w989:bool)  [unwired: 2 out]
                    n373 = Select(t=T16."Stop", s=w989, f=T16."TA[5]") -> (s? t:f=w970:T16)
                  }
                }
              }
            }
          }
        }
        frame "Temp Control" {
          w1007 = "Temperature control test in process..." ("Value")
          w1005 = "Temperature Control Algorithm Test" ("Test Paragraph")
          n374 = control-ref of="Pannel User Message"() -> (w1018:refnum<vi>)
          n375 = call <vilib>:"Open Config Data.vi"("error in (no error)"=w1001, "create file if necessary (T)"=FALSE, "configuration file path"=w1003) -> ("error out"=w1004:errorcluster, "refnum"=w1000:T12)  [unwired: 7 out]
          n376 = property class="Str"(reference=w1018, error in=w1001, "Value"=w1007) -> (error out=w1017:errorcluster)  [unwired: 1 out]
          n377 = call-poly <vilib>:"Read Key.vi"("section"="Marvin", "error in (no error)"=w1004, "default value"="10", "key"="Temp Algorithm", "refnum"=w1000) -> ("error out"=w996:errorcluster, "value"=w994:string, "refnum out"=w995:T12)  [unwired: 1 in, 3 out]
          n378 = Decimal String To Number(string=w994) -> (number=w992:i32)  [unwired: 2 in, 1 out]
          n379 = Less Or Equal To 0?(x=w992) -> (x <= 0?=w993:bool)
          n380 = Select(t=10, s=w993, f=w992) -> (s? t:f=w991:i32)
          n381 = call <vilib>:"Close Config Data.vi"("error in (no error)"=w996, "refnum"=w995) -> ()  [unwired: 8 in, 2 out]
          n382 = control-ref of="Pannel User Message"() -> (w1012:refnum<vi>)
          n383 = control-ref of="Motor Speed RPM"() -> (w1010:refnum<vi>)
          n384 = control-ref of="Stop Button"() -> (w1014:refnum<vi>)
          n385 = control-ref of="ATR"() -> (w1013:refnum<vi>)
          n386 = control-ref of="Config_CANAT"() -> (w1011:refnum<vi>)
          n387 = control-ref of="UUT"() -> (w1009:refnum<vi>)
          n388 = control-ref of="Stop Burn-in"() -> (w1008:refnum<vi>)
          n389 = call "Table_ScrollaBarMarvin.vi"("error in"=w1017, "Line to focus"=w1005, "reference in"=w1019) -> ("error out"=w1016:errorcluster)  [unwired: 2 out]
          n390 = call "Reset old test Values (SubVI).vi"("error in"=w1016, "Atr in"=w1019, "Test Paragraph"=w1005) -> ("error out"=w1006:errorcluster)  [unwired: 8 in]
          n391 = while {
            tunnel: w1006 -> [w1032]
            shift-right: [w1030] -> _
            shift-left: enum16{"Stop", "Algorithm", "Start"}."Start" -> [w1031]
            tunnel: w1014 -> [w1029]
            tunnel: w1013 -> [w1028]
            tunnel: w1012 -> [w1027]
            tunnel: w1011 -> [w1026]
            tunnel: w1010 -> [w1025]
            tunnel: w1009 -> [w1024]
            tunnel: w1008 -> [w1022]
            tunnel: w1007 -> [w1021]
            tunnel: w991 -> [w1020]
            stop <- w1023 stop-if-true
            n392 = case shown="\"Algorithm\"" w1031 {
              tunnel: w1032 -> [_ _ w1169]
              tunnel: [w1033 w1054 w1158] -> w1030
              tunnel: w1029 -> [_ w1065 w1162]
              tunnel: w1028 -> [_ w1061 _]
              tunnel: w1027 -> [_ w1066 _]
              tunnel: w1026 -> [w1036 _ w1143]
              tunnel: w1025 -> [_ w1062 _]
              tunnel: w1024 -> [w1035 _ w1142]
              tunnel: [w1034 FALSE FALSE] -> w1023
              tunnel: w1022 -> [_ w1064 _]
              tunnel: w1021 -> [_ w1063 _]
              tunnel: w1020 -> [_ w1048 _]
              frame "Stop", Default {
                n393 = flat-sequence {
                  tunnel: w1036 -> [w1041]
                  tunnel: w1035 -> [w1039]
                  tunnel: [TRUE] -> w1034
                  tunnel: [enum16{"Stop", "Algorithm", "Start"}."Stop"] -> w1033
                  frame #0 {
                    n394 = call "CANSendMotorSpeed.vi"("Remote"=TRUE, "Motor Speed RPM"=u16 0, "UUT"=w1039, "CAN Cluster in"=w1041) -> ("error out"=w1037:errorcluster)  [unwired: 7 in]
                    n395 = property on="VISA Tester" class="VISAName"() -> ("Value"=w1045:refnum<visa-resource-name>)  [unwired: 2 in, 2 out]
                    n396 = call "TesterOption (SubVI).vi"("2 Options"=FALSE, "error in (no error)"=w1037, "On/Off"=FALSE, "Tester Option"=T13."Venable", "VISA Refnum in"=w1045) -> ()  [unwired: 5 in, 2 out]
                  }
                  frame #1 {
                  }
                  frame #2 {
                  }
                }
              }
              frame "Algorithm" {
                w1049 = T20 [enum."6000", enum."11500", enum."15100", enum."11500-2", enum."6000-2"] items=["6000", "11500", "15100", "11500-2", "6000-2"]
                # "Speed Goal"
                # "Speed Ind"
                # "Temp Goal"
                # "50 Deg"
                n397 = for {
                  tunnel: w1066 -> [w1094]
                  tunnel: w1065 -> [w1093]
                  tunnel: w1064 -> [w1092]
                  tunnel: w1063 -> [w1091]
                  tunnel: w1062 -> [w1090]
                  tunnel: w1061 -> [w1077]
                  tunnel: string[] ["Tair <   67 ± 3 °C", "Tair >= 67 ± 3 °C", "Tair >= 83 ± 3 °C", "Tair <= 80 ± 3 °C", "Tair <= 64 ± 3 °C"] -> [w1075] mode=indexing
                  shift-right: [w1087] -> _
                  shift-left: 1202.0 ("Rt") -> [w1088]
                  tunnel: dbl[] [67.0, 67.0, 83.0, 80.0, 64.0] -> [w1086] mode=indexing
                  tunnel: dbl[] [11500.0, 12700.0, 14700.0, 12700.0, 11500.0] -> [w1085] mode=indexing
                  tunnel: dbl[] [11500.0, 11900.0, 13000.0, 13900.0, 12200.0] -> [w1084] mode=indexing
                  tunnel: [w1073] -> w1055
                  tunnel: [w1072] -> w1051 mode=indexing
                  tunnel: [w1071] -> w1052 mode=indexing
                  tunnel: w1049 -> [w1070] mode=indexing
                  tunnel: w1048 -> [w1069]
                  stop <- w1089 stop-if-true
                  n398 = call <vilib>:"High Resolution Relative Seconds.vi"() -> ("relative seconds"=w1083:dbl)
                  n399 = while {
                    tunnel: w1094 -> [w1123]
                    tunnel: w1093 -> [w1115]
                    tunnel: w1092 -> [w1122]
                    tunnel: w1091 -> [w1101]
                    tunnel: w1090 -> [w1124]
                    shift-right: [w1120] -> w1087
                    shift-left: w1088 -> [w1119]
                    tunnel: w1070 -> [w1121]
                    tunnel: w1086 -> [w1118]
                    tunnel: w1085 -> [w1117]
                    tunnel: w1084 -> [w1116]
                    tunnel: w1083 -> [w1112]
                    tunnel: [w1107] -> w1078
                    tunnel: [w1106] -> w1071
                    tunnel: [w1105] -> w1076
                    tunnel: [w1104] -> w1072
                    tunnel: [w1103] -> w1074
                    tunnel: w1069 -> [w1095]
                    stop <- w1113 stop-if-true
                    n400 = call "DegToDAC (SubVI).vi"("R2"=0.0, "Rt"=w1119) -> ("error out"=w1131:errorcluster, "output array"=w1132:u8[])  [unwired: 8 in]
                    n401 = call <vilib>:"High Resolution Relative Seconds.vi"() -> ("relative seconds"=w1111:dbl)
                    n402 = property on="VISA Tester" class="VISAName"() -> ("Value"=w1134:refnum<visa-resource-name>)  [unwired: 2 in, 2 out]
                    n403 = Byte Array To String(unsigned byte array=w1132) -> (string=w1133:string)
                    n404 = Subtract(x=w1112, y=w1111) -> (x-y=w1110:dbl)
                    n405 = VISA Write(VISA resource name=w1134, write buffer=w1133, error in (no error)=w1131) -> (error out=w1130:errorcluster)  [unwired: 2 out]
                    n406 = Greater Or Equal?(x=w1110, y=120.0) -> (x >= y?=w1108:bool)
                    n407 = call <vilib>:"Clear Errors.vi"("error in (no error)"=w1130) -> ("error out"=w1129:errorcluster)  [unwired: 5 in, 1 out]
                    n408 = control-ref of="Ambient Temperature"() -> (w1102:refnum<vi>)
                    n409 = property class="DigNum (strict)"(reference=w1102) -> ("Value"=w1100:dbl)  [unwired: 1 in, 2 out]
                    n410 = property class="Bool (strict)"(reference=w1115) -> ("Value"=w1114:bool)  [unwired: 1 in, 2 out]
                    n411 = Number To Fractional String(number=w1100, precision (6)=i16 2) -> (F-format string=w1097:string)  [unwired: 2 in]
                    n412 = Concatenate Strings(w1101, "\nAmbient  Temp. [C]: " ("string"), w1097) -> (w1096:string)
                    n413 = call "Write panel message (SubVI).vi"("Stop BurnIn"=w1122, 4:"rpm"=w1124, 5:"rpm"=TRUE ("rpm"), "PrintTime"=TRUE, "Stop"=w1115, "error in (no error)"=w1129, "Time to wait"=5.0, "Strin"=w1096, "String in"=w1123) -> ("error out"=w1128:errorcluster)  [unwired: 2 in]
                    n414 = call "TempAlgoTest (SubVI).vi"("Temp"=w1102, "Speed Ind"=w1116, "Motor Speed RPM"=w1124, "Round"=w1121, "Temp Up In"=w1119, "error in (no error)"=w1128, "String in"=w1123, "Temp Goal"=w1118, "Stop"=w1115, "Speed Goal"=w1117, "Stop BurnIn"=w1122, "AD Resistor Step"=w1095, "Strin"=w1096) -> (14:"Speed Pass/Fail"=w1106:bool, "Temp  Pass/Fail"=w1105:dbl, "Temp Up Out"=w1120:dbl, 17:"Speed Pass/Fail"=w1107:dbl, "Temp Pass/Fail"=w1104:bool, "error out"=w1103:errorcluster)  [unwired: 1 in]
                    n415 = Compound Arithmetic op=OR(w1108, w1106, w1114) -> (w1113:bool)
                  }
                  n416 = property class="Bool (strict)"(reference=w1093) -> ("Value"=w1089:bool)  [unwired: 1 in, 2 out]
                  n417 = call "Find_Number_LineMARVIN.vi"("Test Paragraph"=w1075, "error in"=w1074, "TableIn"=w1077) -> ("error out"=w1079:errorcluster, "Line number"=w1082:i32)  [unwired: 2 in, 2 out]
                  n418 = Increment(x=w1082) -> (x+1=w1081:i32)
                  n419 = call "PassOrFail (SubVI).vi"("index (row)"=w1081, "error in (no error)"=w1079, "Data in"=w1076, "Pass?Fail"=w1072, "Table in"=w1077) -> ("error out"=w1080:errorcluster)  [unwired: 6 in]
                  n420 = call "PassOrFail (SubVI).vi"("index (row)"=w1082, "error in (no error)"=w1080, "Data in"=w1078, "Pass?Fail"=w1071, "Table in"=w1077) -> ("error out"=w1073:errorcluster)  [unwired: 6 in]
                }
                n421 = Build Array (concatenate)(w1052, w1051) -> (w1053:bool[])
                n422 = flat-sequence {
                  tunnel: w1055 -> [_]
                  tunnel: [enum16{"Stop", "Algorithm", "Start"}."Stop"] -> w1054
                  frame #0 {
                  }
                }
                n423 = And Array Elements(Boolean array=w1053) -> (logical AND=→"TempControlResult":bool)
              }
              frame "Start" {
                n424 = call <vilib>:"Clear Errors.vi"("error in (no error)"=w1169) -> ("error out"=w1144:errorcluster)  [unwired: 5 in, 1 out]
                n425 = call "CANSendMotorSpeed.vi"("Remote"=TRUE, "error in (no error)"=w1144, "Motor Speed RPM"=u16 0, "UUT"=w1142, "CAN Cluster in"=w1143) -> ("error out"=w1139:errorcluster)  [unwired: 6 in]
                n426 = call "Time Delay15"("error in (no error)"=w1139) -> ("error out"=w1138:errorcluster)  [unwired: 10 in]
                n427 = call "DegToDAC (SubVI).vi"("error in (no error)"=w1138, "R2"=0.0, "Rt"=1202.0) -> ("error out"=w1149:errorcluster, "output array"=w1150:u8[])  [unwired: 7 in]
                n428 = property on="VISA Tester" class="VISAName"() -> ("Value"=w1152:refnum<visa-resource-name>)  [unwired: 2 in, 2 out]
                n429 = Byte Array To String(unsigned byte array=w1150) -> (string=w1151:string)
                n430 = VISA Write(VISA resource name=w1152, write buffer=w1151, error in (no error)=w1149) -> (error out=w1141:errorcluster)  [unwired: 2 out]
                n431 = call "Time Delay16"("error in (no error)"=w1141) -> ("error out"=w1140:errorcluster)  [unwired: 10 in]
                n432 = property on="VISA Tester" class="VISAName"() -> ("Value"=w1168:refnum<visa-resource-name>)  [unwired: 2 in, 2 out]
                n433 = call "TesterOption (SubVI).vi"("On/Off 2"=TRUE, "Tester Option 2"=T13."Venable", "2 Options"=TRUE, "error in (no error)"=w1140, "On/Off"=TRUE, "Tester Option"=T13."K16", "VISA Refnum in"=w1168) -> ("error out"=w1154:errorcluster)  [unwired: 3 in, 1 out]
                n434 = call "Time Delay12"("error in (no error)"=w1154) -> ("error out"=w1153:errorcluster)  [unwired: 10 in]
                n435 = call "CANSendMotorSpeed.vi"("Remote"=FALSE, "error in (no error)"=w1153, "Motor Speed RPM"=u16 0, "UUT"=w1142, "CAN Cluster in"=w1143) -> ("error out"=w1137:errorcluster)  [unwired: 6 in]
                n436 = call "Time Delay17"("error in (no error)"=w1137) -> ("error out"=w1136:errorcluster)  [unwired: 10 in]
                n437 = property class="Bool (strict)"(reference=w1162, error in=w1136) -> ("Value"=w1161:bool)  [unwired: 2 out]
                n438 = Select(t=enum16{"Stop", "Algorithm", "Start"}."Stop", s=w1161, f=enum16{"Stop", "Algorithm", "Start"}."Algorithm") -> (s? t:f=w1158:enum16{"Stop", "Algorithm", "Start"})
              }
            }
          }
        }
        frame "Burn in" {
          n439 = control-ref of="Stop Button"() -> (w1175:refnum<vi>)
          n440 = control-ref of="Pannel User Message"() -> (w1178:refnum<vi>)
          n441 = control-ref of="ATR"() -> (w1174:refnum<vi>)
          n442 = control-ref of="Config_CANAT"() -> (w1177:refnum<vi>)
          n443 = control-ref of="UUT"() -> (w1176:refnum<vi>)
          n444 = control-ref of="Stop Burn-in"() -> (w1173:refnum<vi>)
          n445 = property on="UUT" class="DigNum (strict)"() -> ("Value"=w1172:u8)  [unwired: 2 in, 2 out]
          n446 = while {
            tunnel: w1178 -> [w1192]
            tunnel: w1174 -> [w1191]
            tunnel: w1177 -> [w1190]
            tunnel: w1176 -> [w1189]
            tunnel: w1175 -> [w1188]
            shift-right: [w1187] -> _
            shift-left: T17."Start" -> [w1194]
            shift-right: [w1193] -> _
            shift-left: _ -> [w1185]
            tunnel: w1173 -> [w1184]
            tunnel: w1172 -> [w1183]
            tunnel: w1171 -> [w1182]
            shift-right: [w1181] -> _
            shift-left: FALSE -> [w1180]
            stop <- w1186 stop-if-true
            n447 = case shown="\"DC Current Measure\"" w1194 {
              tunnel: [w1200 w1236 w1304 w1331 w1361 w1395] -> w1193
              tunnel: w1192 -> [_ w1228 _ _ _ w1394]
              tunnel: w1191 -> [_ w1231 w1277 w1318 w1347 w1381]
              tunnel: w1190 -> [w1196 w1227 _ _ _ w1393]
              tunnel: w1189 -> [w1195 w1224 _ _ _ w1374]
              tunnel: w1188 -> [_ _ w1306 w1333 w1365 w1387]
              tunnel: [w1198 T17."Stop" w1307 w1334 w1366 w1383] -> w1187
              tunnel: [w1199 FALSE FALSE FALSE FALSE FALSE] -> w1186
              tunnel: w1185 -> [w1200 w1236 w1304 w1331 w1361 _]
              tunnel: w1184 -> [_ _ _ _ _ w1377]
              tunnel: w1183 -> [_ w1220 w1271 w1313 w1342 w1373]
              tunnel: w1182 -> [_ w1216 _ _ _ _]
              tunnel: [FALSE ("Stop Burn-in") w1215 FALSE w1311 w1339 FALSE ("Stop Burn-in")] -> w1181
              tunnel: w1180 -> [_ _ w1266 _ _ _]
              frame "Stop", Default {
                n448 = flat-sequence {
                  tunnel: w1196 -> [w1203]
                  tunnel: w1195 -> [w1202]
                  tunnel: [TRUE] -> w1199
                  tunnel: [T17."Stop"] -> w1198
                  frame #0 {
                    w1201 = u16 0 ("Motor Speed RPM")
                    n449 = call "CANSendMotorSpeed.vi"("Remote"=TRUE, "Motor Speed RPM"=w1201, "UUT"=w1202, "CAN Cluster in"=w1203) -> ("error out"=w1205:errorcluster)  [unwired: 7 in]
                    n450 = property on="BurnInSpeed" class="DigNum (strict)"("Value"=w1201) -> ()  [unwired: 2 in, 2 out]
                    n451 = property on="VISA Tester" class="VISAName"() -> ("Value"=w1210:refnum<visa-resource-name>)  [unwired: 2 in, 2 out]
                    n452 = call "TesterOption (SubVI).vi"("2 Options"=FALSE, "error in (no error)"=w1205, "On/Off"=FALSE, "Tester Option"=T13."Venable", "VISA Refnum in"=w1210) -> ("error out"=w1207:errorcluster)  [unwired: 5 in, 1 out]
                    n453 = property on="Stop Burn-in" class="Bool (strict)"(error in=w1207, "Visible"=FALSE) -> ()  [unwired: 1 in, 2 out]
                  }
                  frame #1 {
                  }
                }
              }
              frame "BurnIn" {
                w1215 = FALSE ("Stop Burn-in")
                n454 = control-ref of="Motor Speed RPM"() -> (w1230:refnum<vi>)
                n455 = control-ref of="Stop Button"() -> (w1229:refnum<vi>)
                n456 = property on="Stop Burn-in" class="Bool (strict)"("Visible"=w1216) -> (error out=w1232:errorcluster)  [unwired: 2 in, 1 out]
                n457 = Equal?(x=w1220, y=u8 95) -> (x = y?=w1219:bool)
                n458 = call "Find_Number_LineMARVIN.vi"("Test Paragraph"="After 10 min of operation", "error in"=w1232, "TableIn"=w1231) -> ("error out"=w1234:errorcluster, "Line number"=w1235:i32)  [unwired: 2 in, 2 out]
                n459 = Select(t=u16 14700, s=w1219, f=u16 12100 ("y")) -> (s? t:f=w1222:u16)
                n460 = for {
                  tunnel: w1234 -> [w1253]
                  tunnel: dbl[] [600.0, 600.0, 600.0] -> [w1257] mode=indexing
                  tunnel: w1235 -> [w1262]
                  tunnel: w1231 -> [w1252]
                  tunnel: w1230 -> [w1251]
                  tunnel: w1229 -> [w1250]
                  tunnel: w1228 -> [w1249]
                  tunnel: w1227 -> [w1245]
                  tunnel: w1224 -> [w1244]
                  tunnel: w1222 -> [w1240]
                  tunnel: [w1242] -> w1221
                  tunnel: [w1241] -> w1218 mode=indexing
                  i -> [w1259]
                  n461 = call "CANSendMotorSpeed.vi"("Remote"=TRUE, "error in (no error)"=w1253, "Motor Speed RPM"=w1240, "UUT"=w1244, "CAN Cluster in"=w1245) -> ("error out"=w1247:errorcluster)  [unwired: 6 in]
                  n462 = control-ref of="Stop Burn-in"() -> (w1248:refnum<vi>)
                  n463 = Add(x=w1262, y=w1259) -> (x+y=w1258:i32)
                  n464 = call "Write panel message (SubVI).vi"("Stop BurnIn"=w1248, 4:"rpm"=w1251, 5:"rpm"=TRUE ("rpm"), "PrintTime"=TRUE, "Stop"=w1250, "error in (no error)"=w1247, "Time to wait"=w1257, "Strin"="Burn-in test in process...", "String in"=w1249) -> ("error out"=w1254:errorcluster)  [unwired: 2 in]
                  n465 = control-ref of="Power transistor Heat sink Temp."() -> (w1263:refnum<vi>)
                  n466 = property on="MaxBurnInTempVal" class="DigNum (strict)"() -> ("Value"=w1261:dbl)  [unwired: 2 in, 2 out]
                  n467 = property class="DigNum (strict)"(reference=w1263, error in=w1254) -> (error out=w1243:errorcluster, "Value"=w1260:dbl)  [unwired: 1 out]
                  n468 = property on="BurnInSpeed" class="DigNum (strict)"("Value"=w1240) -> ()  [unwired: 2 in, 2 out]
                  n469 = Less Or Equal?(x=w1260, y=w1261) -> (x <= y?=w1241:bool)
                  n470 = call "PassOrFail (SubVI).vi"("index (row)"=w1258, "error in (no error)"=w1243, "Data in"=w1260, "Pass?Fail"=w1241, "Table in"=w1252) -> ("error out"=w1242:errorcluster)  [unwired: 6 in]
                }
                n471 = And Array Elements(Boolean array=w1218) -> (logical AND=→"BurnResult":bool)
                n472 = property on="Stop Burn-in" class="Bool (strict)"(error in=w1221, "Value"=w1215, "Visible"=w1215) -> ()  [unwired: 1 in, 2 out]
              }
              frame "Ambient Temp" {
                w1282 = 2 ("disabled index (col)")
                n473 = control-ref of="Power transistor Heat sink Temp."() -> (w1292:refnum<vi>)
                n474 = call "Find_Number_LineMARVIN.vi"("Test Paragraph"="Ambient Temperature", "TableIn"=w1277) -> ("error out"=w1303:errorcluster, "Line number"=w1283:i32)  [unwired: 3 in, 2 out]
                n475 = Equal?(x=w1271, y=u8 95) -> (x = y?=w1272:bool)
                n476 = property class="DigNum (strict)"(reference=w1292, error in=w1303) -> (error out=w1294:errorcluster, "Value"=w1284:dbl)  [unwired: 1 out]
                n477 = Select(t=25.0 ("y"), s=w1272, f=25.0 ("y")) -> (s? t:f=w1293:dbl)
                n478 = Select(t=13.0 ("y"), s=w1272, f=13.0) -> (s? t:f=w1295:dbl)
                n479 = Add(x=w1293, y=w1295) -> (x+y=w1302:dbl)
                n480 = Subtract(x=w1293, y=w1295) -> (x-y=w1301:dbl)
                n481 = In Range and Coerce(upper limit=w1302, x=w1284, lower limit=w1301) -> (In Range?=w1268:bool)  [unwired: 1 out]
                "BurnTemp" <- w1268
                n482 = call "PassOrFail (SubVI).vi"("index (row)"=w1283, "error in (no error)"=w1294, "Data in"=w1284, "Pass?Fail"=w1268, "Table in"=w1277) -> ("error out"=w1274:errorcluster)  [unwired: 6 in]
                n483 = property class="Tbl (strict)"(reference=w1277, error in=w1274) -> (reference out=w1276:refnum<vi>, error out=w1291:errorcluster, "Value"=w1290:string[][])
                n484 = Add(x=w1284, y=25.0) -> (x+y=w1275:dbl)
                "MaxBurnInTempVal" <- w1275
                n485 = Number To Fractional String(number=w1275, precision (6)=i16 0) -> (F-format string=w1289:string)  [unwired: 2 in]
                n486 = Concatenate Strings("< " ("string"), w1289) -> (w1278:string)
                n487 = Increment(x=w1283) -> (x+1=w1281:i32)
                n488 = Increment(x=w1281) -> (x+1=w1280:i32)
                n489 = Increment(x=w1280) -> (x+1=w1279:i32)
                n490 = Replace Array Subset(array=w1290, new element #1=w1278, index (row) #1=w1281, index (col) #1=w1282, new element #2=w1278, index (row) #2=w1280, index (col) #2=w1282, new element #3=w1278, index (row) #3=w1279, index (col) #3=w1282) -> (w1288:string[][])
                n491 = Not(x=w1268) -> (.not. x?=w1267:bool)
                n492 = property class="Tbl (strict)"(reference=w1276, error in=w1291, "Value"=w1288) -> (error out=w1273:errorcluster)  [unwired: 1 out]
                n493 = property class="Bool (strict)"(reference=w1306, error in=w1273) -> ("Value"=w1269:bool)  [unwired: 2 out]
                n494 = Compound Arithmetic op=OR(w1267, w1266, w1269) -> (w1270:bool)
                n495 = Select(t=T17."Stop", s=w1270, f=T17."BurnIn") -> (s? t:f=w1307:T17)
              }
              frame "MotorSpeed" {
                n496 = control-ref of="Motor Speed RPM"() -> (w1316:refnum<vi>)
                n497 = Equal?(x=w1313, y=u8 95) -> (x = y?=w1314:bool)
                n498 = call "Find_Number_LineMARVIN.vi"("Test Paragraph"="Fan speed", "TableIn"=w1318) -> ("error out"=w1330:errorcluster, "Line number"=w1321:i32)  [unwired: 3 in, 2 out]
                n499 = property class="DigNum (strict)"(reference=w1316, error in=w1330) -> (error out=w1319:errorcluster, "Value"=w1320:dbl)  [unwired: 1 out]
                n500 = Select(t=14700.0 ("y"), s=w1314, f=12100.0 ("y")) -> (s? t:f=w1317:dbl)
                n501 = Select(t=200.0 ("y"), s=w1314, f=200.0) -> (s? t:f=w1322:dbl)
                n502 = Add(x=w1317, y=w1322) -> (x+y=w1329:dbl)
                n503 = Subtract(x=w1317, y=w1322) -> (x-y=w1328:dbl)
                n504 = In Range and Coerce(upper limit=w1329, x=w1320, lower limit=w1328) -> (In Range?=w1312:bool)  [unwired: 1 out]
                "BurnSpeed" <- w1312
                n505 = call "PassOrFail (SubVI).vi"("index (row)"=w1321, "error in (no error)"=w1319, "Data in"=w1320, "Pass?Fail"=w1312, "Table in"=w1318) -> ("error out"=w1315:errorcluster)  [unwired: 6 in]
                n506 = property class="Bool (strict)"(reference=w1333, error in=w1315) -> ("Value"=w1337:bool)  [unwired: 2 out]
                n507 = Select(t=T17."Stop", s=w1337, f=T17."Ambient Temp") -> (s? t:f=w1334:T17)
                n508 = Not(x=w1312) -> (.not. x?=w1311:bool)
              }
              frame "DC Current Measure" {
                n509 = property on="VISA Tester" class="VISAName"() -> (error out=w1359:errorcluster, "Value"=w1363:refnum<visa-resource-name>)  [unwired: 2 in, 1 out]
                n510 = call "GetADCTester (SubVI).vi"("error in (no error)"=w1359, "GetADCTester"=T15."Current", "TimeToGet"=10, "VISA Refnum in"=w1363) -> ("error out"=w1360:errorcluster, "ADCValOutput Single"=w1346:dbl)  [unwired: 5 in, 1 out]
                n511 = Equal?(x=w1342, y=u8 95) -> (x = y?=w1343:bool)
                n512 = call "Find_Number_LineMARVIN.vi"("Test Paragraph"="DC Input Current", "error in"=w1360, "TableIn"=w1347) -> ("error out"=w1358:errorcluster, "Line number"=w1348:i32)  [unwired: 2 in, 2 out]
                n513 = Select(t=45.0 ("y"), s=w1343, f=28.0 ("y")) -> (s? t:f=w1350:dbl)
                n514 = Select(t=5.0 ("y"), s=w1343, f=3.0) -> (s? t:f=w1349:dbl)
                n515 = Add(x=w1350, y=w1349) -> (x+y=w1357:dbl)
                n516 = Subtract(x=w1350, y=w1349) -> (x-y=w1356:dbl)
                n517 = In Range and Coerce(upper limit=w1357, x=w1346, lower limit=w1356) -> (In Range?=w1341:bool)  [unwired: 1 out]
                "BurnDC" <- w1341
                n518 = call "PassOrFail (SubVI).vi"("index (row)"=w1348, "error in (no error)"=w1358, "Data in"=w1346, "Pass?Fail"=w1341, "Table in"=w1347) -> ("error out"=w1345:errorcluster)  [unwired: 6 in]
                n519 = property class="Bool (strict)"(reference=w1365, error in=w1345) -> ("Value"=w1340:bool)  [unwired: 2 out]
                n520 = Not(x=w1341) -> (.not. x?=w1339:bool)
                n521 = Select(t=T17."Stop", s=w1340, f=T17."MotorSpeed") -> (s? t:f=w1366:T17)
              }
              frame "Start" {
                w1369 = "Burn-in Test" ("Line to focus")
                w1371 = "Burn-in test in process...\nFull Speed Operation" ("Value")
                n522 = Equal?(x=w1373, y=u8 95) -> (x = y?=w1375:bool)
                n523 = property class="Str"(reference=w1394, "Value"=w1371) -> (reference out=w1391:refnum<vi>, error out=w1376:errorcluster)  [unwired: 1 in]
                n524 = call "Find_Number_LineMARVIN.vi"("Test Paragraph"=w1369, "error in"=w1376, "TableIn"=w1381) -> ("error out"=w1401:errorcluster, "Line number"=w1402:i32)  [unwired: 2 in, 2 out]
                n525 = Select(t=u16 14700 ("y"), s=w1375, f=u16 12100 ("y")) -> (s? t:f=w1408:u16)
                "BurnInSpeed" <- w1408
                n526 = call "Table_ScrollaBarMarvin.vi"("error in"=w1401, "Line to focus"=w1369, "reference in"=w1381) -> ("error out"=w1403:errorcluster)  [unwired: 2 out]
                n527 = call "Reset old test Values (SubVI).vi"("error in"=w1403, "Atr in"=w1381, "Test Paragraph"=w1369) -> ("error out"=w1404:errorcluster)  [unwired: 8 in]
                n528 = Increment(x=w1402) -> (x+1=w1395:i32)
                n529 = property on="VISA Tester" class="VISAName"(error in=w1404) -> (error out=w1405:errorcluster, "Value"=w1406:refnum<visa-resource-name>)  [unwired: 1 in, 1 out]
                n530 = call "TesterOption (SubVI).vi"("2 Options"=FALSE, "error in (no error)"=w1405, "On/Off"=TRUE, "Tester Option"=T13."Venable", "VISA Refnum in"=w1406) -> ("error out"=w1407:errorcluster)  [unwired: 5 in, 1 out]
                n531 = call "CANSendMotorSpeed.vi"("Remote"=TRUE, "error in (no error)"=w1407, "Motor Speed RPM"=w1408, "UUT"=w1374, "CAN Cluster in"=w1393) -> ("error out"=w1392:errorcluster)  [unwired: 6 in]
                n532 = control-ref of="Motor Speed RPM"() -> (w1380:refnum<vi>)
                n533 = call "Write panel message (SubVI).vi"("Stop BurnIn"=w1377, 4:"rpm"=w1380, 5:"rpm"=TRUE ("rpm"), "PrintTime"=TRUE, "Stop"=w1387, "error in (no error)"=w1392, "Time to wait"=50.0, "Strin"=w1371, "String in"=w1391) -> ("error out"=w1379:errorcluster)  [unwired: 2 in]
                n534 = property class="Bool (strict)"(reference=w1387, error in=w1379) -> ("Value"=w1386:bool)  [unwired: 2 out]
                n535 = Select(t=T17."Stop", s=w1386, f=T17."DC Current Measure") -> (s? t:f=w1383:T17)
              }
            }
          }
        }
        frame "Visual Inspec" {
          n536 = control-ref of="Stop Button"() -> (w1412:refnum<vi>)
          n537 = property class="Bool (strict)"(reference=w1412, error in=w1411) -> (error out=w1410:errorcluster, "Value"=w1409:bool)  [unwired: 1 out]
          n538 = case shown="False" w1409 {
            tunnel: w1413 -> [w1427 _]
            tunnel: w1410 -> [w1414 _]
            frame False {
              n539 = property on="VISA Tester" class="VISAName"() -> ("Value"=w1426:refnum<visa-resource-name>)  [unwired: 2 in, 2 out]
              n540 = call "TesterOption (SubVI).vi"("2 Options"=FALSE, "error in (no error)"=w1414, "On/Off"=FALSE, "Tester Option"=T13."Venable", "VISA Refnum in"=w1426) -> ("error out"=w1422:errorcluster)  [unwired: 5 in, 1 out]
              n541 = local read "UUT"() -> (w1418:u8)
              n542 = Equal?(x=w1418, y=u8 95) -> (x = y?=w1419:bool)
              n543 = case shown="True" w1419 {
                tunnel: w1427 -> [w1431 w1441]
                tunnel: w1422 -> [w1430 w1440]
                tunnel: [w1432 w1443] -> w1421
                tunnel: [w1433 w1442] -> w1417
                tunnel: string[] ["Verification of Components Not Installed", "Manufacturing Defects", "DC Input Current Drawn", "12V", "5V", "3.3V", "1.8V", "Reverse Polarity Test - DC Input Current", "Weight Check", "J3.B to Chassis", "J1.16 to Chassis", "J1 Body to Chassis", "J2  Body to Chassis", "J3  Body to Chassis", "J1.17 to J1.18", "Sealing Test", "Mounting Holes Test - Jig Fit"] ("deleted portion 3") -> [w1428 w1438]
                frame False {
                  # "AHU"
                  n544 = for {
                    tunnel: w1428 -> [w1437] mode=indexing
                    tunnel: w1431 -> [w1436]
                    tunnel: w1430 -> [w1435]
                    tunnel: [w1434] -> w1429
                    n545 = call "Reset old test Values (SubVI).vi"("error in"=w1435, "Atr in"=w1436, "Test Paragraph"=w1437) -> ("error out"=w1434:errorcluster)  [unwired: 8 in]
                  }
                  n546 = call "VisualInspectionAHUold.vi"("error in (no error)"=w1429, "TableRef"=w1431) -> ("error out"=w1433:errorcluster, "VisualInspectionResult"=w1432:bool)  [unwired: 8 in]
                }
                frame True {
                  # "EBAY"
                  n547 = for {
                    tunnel: w1441 -> [w1447]
                    tunnel: w1440 -> [w1446]
                    tunnel: [w1445] -> w1439
                    tunnel: w1438 -> [w1444] mode=indexing
                    n548 = call "Reset old test Values (SubVI).vi"("error in"=w1446, "Atr in"=w1447, "Test Paragraph"=w1444) -> ("error out"=w1445:errorcluster)  [unwired: 8 in]
                  }
                  n549 = call "VisualInspectionEBAYold.vi"("error in (no error)"=w1439, "TableRef"=w1441) -> ("error out"=w1442:errorcluster, "VisualInspectionResult"=w1443:bool)  [unwired: 8 in]
                }
              }
              "VisualInspectionResult" <- w1421
              n550 = property on="Automation" class="Bool (strict)"(error in=w1417) -> ("Value"=w1416:bool)  [unwired: 1 in, 2 out]
              n551 = case shown="True" w1416 {
                frame False {
                }
                frame True {
                  w1448 = TRUE ("Value (Signaling)")
                  n552 = property on="SetSN" class="Bool (strict)"("Val(Sgnl)"=w1448, "Value"=w1448) -> ()  [unwired: 2 in, 2 out]
                }
              }
            }
            frame True {
            }
          }
        }
        frame "Temp Sens Cal" {
          w1452 = "Temperature sensor calibration test in process..." ("Value")
          w1450 = "Temperature Sensor Calibration" ("Test Paragraph")
          n553 = control-ref of="Pannel User Message"() -> (w1459:refnum<vi>)
          n554 = property class="Str"(reference=w1459, error in=w1458, "Value"=w1452) -> (error out=w1457:errorcluster)  [unwired: 1 out]
          n555 = call "Table_ScrollaBarMarvin.vi"("error in"=w1457, "Line to focus"=w1450, "reference in"=w1460) -> ("error out"=w1462:errorcluster)  [unwired: 2 out]
          n556 = property class="Tbl (strict)"(reference=w1460, error in=w1462) -> (reference out=w1449:refnum<vi>, error out=w1464:errorcluster, "Value"=w1465:string[][])
          n557 = Index Array(array=w1465, index (col)=1 ("disabled index (col)")) -> (element=w1466:string[])  [unwired: 1 in]
          n558 = call "Find_Number_Line.vi"("error in"=w1464, "Test Paragraph"=w1450, "Row Headers[]"=w1466) -> ("error out"=w1461:errorcluster, "Line number"=w1454:i32)  [unwired: 1 out]
          n559 = property on="Status" class="Bool (strict)"(error in=w1461) -> (error out=w1455:errorcluster, "Value"=w1456:bool)  [unwired: 1 in, 1 out]
          n560 = call "Reset old test Values (SubVI).vi"("error in"=w1455, "Atr in"=w1449, "Test Paragraph"=w1450) -> ("error out"=w1451:errorcluster)  [unwired: 8 in]
          n561 = case shown="True" w1456 {
            selector: w1456 -> [w1470 _]
            tunnel: w1451 -> [w1472 _]
            tunnel: w1449 -> [w1469 _]
            tunnel: w1454 -> [w1468 _]
            tunnel: w1453 -> [_ w1479]
            tunnel: w1452 -> [_ w1475]
            frame False {
              n562 = flat-sequence {
                tunnel: w1472 -> [w1473]
                tunnel: [w1473] -> w1471
                frame #0 {
                  n563 = One Button Dialog(message="Please establish RS connection.") -> ()  [unwired: 1 in, 1 out]
                }
              }
              n564 = Increment(x=w1468) -> (x+1=w1467:i32)
              n565 = call "PassOrFail (SubVI).vi"("index (row)"=w1467, "error in (no error)"=w1471, "Pass?Fail"=w1470, "Table in"=w1469) -> ()  [unwired: 7 in, 1 out]
            }
            frame True {
              n566 = control-ref of="Stop Burn-in"() -> (w1481:refnum<vi>)
              n567 = control-ref of="Pannel User Message"() -> (w1483:refnum<vi>)
              n568 = control-ref of="Config_CANAT"() -> (w1477:refnum<vi>)
              n569 = control-ref of="ATR"() -> (w1484:refnum<vi>)
              n570 = control-ref of="Motor Speed RPM"() -> (w1485:refnum<vi>)
              n571 = control-ref of="UUT"() -> (w1476:refnum<vi>)
              n572 = control-ref of="Stop Button"() -> (w1482:refnum<vi>)
              n573 = property on="VISA Tester" class="VISAName"() -> ("Value"=w1478:refnum<visa-resource-name>)  [unwired: 2 in, 2 out]
              n574 = while {
                shift-right: [w1488] -> _
                shift-left: T16."Start" -> [w1498]
                tunnel: w1481 -> [w1497]
                tunnel: w1482 -> [w1496]
                tunnel: w1483 -> [w1495]
                tunnel: w1484 -> [w1494]
                tunnel: w1485 -> [w1493]
                tunnel: w1479 -> [w1492]
                tunnel: w1478 -> [w1491]
                tunnel: w1477 -> [w1490]
                tunnel: w1476 -> [w1489]
                tunnel: w1475 -> [w1486]
                stop <- w1487 stop-if-true
                n575 = case shown="\"Stop\", Default" w1498 {
                  tunnel: w1497 -> [_ w1533 w1560 w1615 w1645]
                  tunnel: w1496 -> [_ w1534 w1552 w1601 w1647]
                  tunnel: w1495 -> [_ w1531 w1561 w1613 w1649]
                  tunnel: w1494 -> [_ w1511 _ _ _]
                  tunnel: w1493 -> [_ w1535 w1559 w1616 w1644]
                  tunnel: w1492 -> [_ w1544 w1564 w1625 w1641]
                  tunnel: w1491 -> [w1501 w1540 w1563 w1621 w1629]
                  tunnel: w1490 -> [_ _ _ _ w1655]
                  tunnel: w1489 -> [_ _ _ _ w1654]
                  tunnel: [w1499 w1520 w1553 w1604 w1632] -> w1488
                  tunnel: [w1500 FALSE FALSE FALSE FALSE] -> w1487
                  tunnel: w1486 -> [_ _ w1562 _ _]
                  frame "Stop", Default {
                    n576 = flat-sequence {
                      tunnel: w1501 -> [w1502]
                      tunnel: [TRUE] -> w1500
                      tunnel: [T16."Stop"] -> w1499
                      frame #0 {
                        n577 = call "TesterOption (SubVI).vi"("2 Options"=FALSE, "On/Off"=FALSE, "Tester Option"=T13."Venable", "VISA Refnum in"=w1502) -> ()  [unwired: 6 in, 2 out]
                      }
                      frame #1 {
                      }
                    }
                  }
                  frame "AO[1]=Meas." {
                    n578 = property on="AO[1]Meas" class="DigNum (strict)"() -> ("Value"=w1514:dbl)  [unwired: 2 in, 2 out]
                    n579 = Number To Fractional String(number=w1514) -> (F-format string=w1522:string)  [unwired: 3 in]
                    n580 = Search and Replace String(input string="EP=1\r\nAO[1]=0\r\n" ("write buffer"), search string="0", replace string=w1522) -> (result string=w1521:string)  [unwired: 5 in, 3 out]
                    n581 = call "SerialMarvinSendGet.vi"("Clear Log"=FALSE, "write buffer"=w1521, "VISA resource name"=w1544) -> ("error out"=w1539:errorcluster)  [unwired: 7 in, 1 out]
                    n582 = call "TesterOption (SubVI).vi"("2 Options"=FALSE, "error in (no error)"=w1539, "On/Off"=FALSE, "Tester Option"=T13."Power", "VISA Refnum in"=w1540) -> ("error out"=w1538:errorcluster, "VISA Refnum out"=w1525:refnum<visa-resource-name>)  [unwired: 5 in]
                    n583 = call "Write panel message (SubVI).vi"("Stop BurnIn"=w1533, 4:"rpm"=w1535, 5:"rpm"=FALSE ("rpm"), "PrintTime"=TRUE, "Stop"=w1534, "error in (no error)"=w1538, "Time to wait"=20.0, "Strin"="Temperature sensor calibration test in process...\nSet Parameters...", "String in"=w1531) -> ("error out"=w1526:errorcluster)  [unwired: 2 in]
                    n584 = call "TesterOption (SubVI).vi"("2 Options"=FALSE, "error in (no error)"=w1526, "On/Off"=FALSE, "Tester Option"=T13."Venable", "VISA Refnum in"=w1525) -> ("error out"=w1519:errorcluster)  [unwired: 5 in, 1 out]
                    n585 = flat-sequence {
                      tunnel: [T16."Stop"] -> w1520
                      tunnel: w1512 -> [_]
                      frame #0 {
                      }
                    }
                    n586 = In Range and Coerce(upper limit=0.1, x=w1514, lower limit=-0.1) -> (In Range?=w1509:bool)  [unwired: 1 out]
                    "SensCalResult" <- w1509
                    n587 = call "Find_Number_LineMARVIN.vi"("Test Paragraph"="Sensor Reading Analog Offset", "error in"=w1519, "TableIn"=w1511) -> ("error out"=w1513:errorcluster, "Line number"=w1517:i32)  [unwired: 2 in, 2 out]
                    n588 = call "PassOrFail (SubVI).vi"("Test#"="2", "index (row)"=w1517, "error in (no error)"=w1513, "Data in"=w1514, "Pass?Fail"=w1509, "Table in"=w1511) -> ("error out"=w1512:errorcluster)  [unwired: 5 in]
                  }
                  frame "TA[5]" {
                    w1565 = T19 [enum."50C", enum."80C", enum."100C", enum."120C"] items=["K15", "K16", "K17", "Venable", "Firmeware", "Fan", "Power", "120C", "110C", "100C", "90C", "80C", "70C", "60C", "50C", "40C", "30C", "25C", "20C", "10C", "0C"]
                    n589 = for {
                      tunnel: w1565 -> [w1580] mode=indexing
                      tunnel: w1564 -> [w1579]
                      tunnel: w1563 -> [w1578]
                      tunnel: w1562 -> [w1577]
                      tunnel: w1561 -> [w1576]
                      tunnel: w1552 -> [w1575]
                      tunnel: w1560 -> [w1574]
                      tunnel: w1559 -> [w1573]
                      tunnel: dbl[] [0.59774, 0.65238, 0.68545, 0.71584] -> [w1568] mode=indexing
                      tunnel: [w1567] -> w1548 mode=indexing
                      tunnel: [w1566] -> w1551
                      n590 = for {
                        N: 5 -> [_]
                        tunnel: w1580 -> [w1598]
                        tunnel: w1579 -> [w1597]
                        tunnel: w1578 -> [w1593]
                        tunnel: w1577 -> [w1591]
                        tunnel: w1576 -> [w1590]
                        tunnel: w1575 -> [w1589]
                        tunnel: w1574 -> [w1587]
                        tunnel: w1573 -> [w1584]
                        tunnel: [w1583] -> w1572 mode=indexing
                        tunnel: [w1582] -> w1566
                        n591 = call "TesterOption (SubVI).vi"("2 Options"=FALSE, "On/Off"=TRUE, "Tester Option"=w1598, "VISA Refnum in"=w1593) -> ("error out"=w1594:errorcluster)  [unwired: 6 in, 1 out]
                        n592 = call "Write panel message (SubVI).vi"("Stop BurnIn"=w1587, 4:"rpm"=w1584, 5:"rpm"=FALSE ("rpm"), "PrintTime"=FALSE, "Stop"=w1589, "error in (no error)"=w1594, "Time to wait"=1.0, "Strin"=w1591, "String in"=w1590) -> ("error out"=w1592:errorcluster)  [unwired: 2 in]
                        n593 = call "SerialMarvinSendGet.vi"("error in (no error)"=w1592, "write buffer"="TA[5]\r\n", "VISA resource name"=w1597) -> ("error out"=w1582:errorcluster, "read buffer"=w1595:string)  [unwired: 7 in]
                        n594 = Fract/Exp String To Number(string=w1595) -> (number=w1583:dbl)  [unwired: 3 in, 1 out]
                      }
                      n595 = Add Array Elements(numeric array=w1572) -> (sum=w1571:dbl)
                      n596 = Divide(x=w1571, y=5.0) -> (x/y=w1569:dbl)
                      n597 = Subtract(x=w1569, y=w1568) -> (x-y=w1567:dbl)
                    }
                    n598 = property class="Bool (strict)"(reference=w1552, error in=w1551) -> ("Value"=w1557:bool)  [unwired: 2 out]
                    n599 = Select(t=T16."Stop", s=w1557, f=T16."AO[1]=Meas.") -> (s? t:f=w1553:T16)
                    n600 = Array Size(array=w1548) -> (size(s)=w1547:i32)
                    n601 = Add Array Elements(numeric array=w1548) -> (sum=w1550:dbl)
                    n602 = Divide(x=w1550, y=w1547) -> (x/y=→"AO[1]Meas":dbl)
                  }
                  frame "AO[1]=0" {
                    n603 = call "SerialMarvinSendGet.vi"("write buffer"="EP=1\r\nAO[1]=0\r\n", "VISA resource name"=w1625) -> ("error out"=w1620:errorcluster)  [unwired: 8 in, 1 out]
                    n604 = call "TesterOption (SubVI).vi"("2 Options"=FALSE, "error in (no error)"=w1620, "On/Off"=FALSE, "Tester Option"=T13."Power", "VISA Refnum in"=w1621) -> ("error out"=w1619:errorcluster, "VISA Refnum out"=w1607:refnum<visa-resource-name>)  [unwired: 5 in]
                    n605 = call "Write panel message (SubVI).vi"("Stop BurnIn"=w1615, 4:"rpm"=w1616, 5:"rpm"=FALSE ("rpm"), "PrintTime"=TRUE, "Stop"=w1601, "error in (no error)"=w1619, "Time to wait"=20.0, "Strin"="Temperature sensor calibration test in process...\nSet Parameters...", "String in"=w1613) -> ("error out"=w1608:errorcluster)  [unwired: 2 in]
                    n606 = call "TesterOption (SubVI).vi"("2 Options"=FALSE, "error in (no error)"=w1608, "On/Off"=FALSE, "Tester Option"=T13."Venable", "VISA Refnum in"=w1607) -> ("error out"=w1602:errorcluster)  [unwired: 5 in, 1 out]
                    n607 = property class="Bool (strict)"(reference=w1601, error in=w1602) -> ("Value"=w1606:bool)  [unwired: 2 out]
                    n608 = Select(t=T16."Stop", s=w1606, f=T16."TA[5]") -> (s? t:f=w1604:T16)
                  }
                  frame "Start" {
                    n609 = call "Write panel message (SubVI).vi"("Stop BurnIn"=w1645, 4:"rpm"=w1644, 5:"rpm"=FALSE ("rpm"), "PrintTime"=FALSE, "Stop"=w1647, "Time to wait"=0.1, "Strin"="Temperature sensor calibration test in process...\nInitialization state...", "String in"=w1649) -> ("error out"=w1650:errorcluster)  [unwired: 3 in]
                    n610 = call "TesterOption (SubVI).vi"("2 Options"=FALSE, "error in (no error)"=w1650, "On/Off"=FALSE, "Tester Option"=T13."Venable", "VISA Refnum in"=w1629) -> ("error out"=w1652:errorcluster)  [unwired: 5 in, 1 out]
                    n611 = call "CANSendMotorSpeed.vi"("Remote"=TRUE, "error in (no error)"=w1652, "Motor Speed RPM"=u16 0, "UUT"=w1654, "CAN Cluster in"=w1655) -> ("error out"=w1639:errorcluster)  [unwired: 6 in]
                    n612 = call "SerialMarvinSendGet.vi"("error in (no error)"=w1639, "write buffer"="AO[1]\r\n", "VISA resource name"=w1641) -> ("error out"=w1628:errorcluster, "read buffer"=w1638:string)  [unwired: 7 in]
                    n613 = Equal?(x=w1638, y="0.0") -> (x = y?=w1630:bool)
                    n614 = property class="Bool (strict)"(reference=w1647, error in=w1628) -> ("Value"=w1659:bool)  [unwired: 2 out]
                    n615 = Select(t=T16."TA[5]", s=w1630, f=T16."AO[1]=0") -> (s? t:f=w1634:T16)
                    n616 = Select(t=T16."Stop", s=w1659, f=w1634) -> (s? t:f=w1632:T16)
                  }
                }
              }
            }
          }
        }
        frame "Auxiliary" {
          w1664 = "Auxiliary test in process..." ("Value")
          w1676 = "Auxiliary Fan Test" ("Test Paragraph")
          n617 = control-ref of="Pannel User Message"() -> (w1675:refnum<vi>)
          n618 = property class="Str"(reference=w1675, error in=w1672, "Value"=w1664) -> (error out=w1674:errorcluster)  [unwired: 1 out]
          n619 = call "Table_ScrollaBarMarvin.vi"("error in"=w1674, "Line to focus"=w1676, "reference in"=w1673) -> ("error out"=w1682:errorcluster)  [unwired: 2 out]
          n620 = property class="Tbl (strict)"(reference=w1673, error in=w1682) -> (reference out=w1671:refnum<vi>, error out=w1681:errorcluster, "Value"=w1680:string[][])
          n621 = Index Array(array=w1680, index (col)=1 ("disabled index (col)")) -> (element=w1679:string[])  [unwired: 1 in]
          n622 = call "Find_Number_Line.vi"("error in"=w1681, "Test Paragraph"=w1676, "Row Headers[]"=w1679) -> ("error out"=w1677:errorcluster, "Line number"=w1662:i32)  [unwired: 1 out]
          n623 = call "Reset old test Values (SubVI).vi"("error in"=w1677, "Atr in"=w1671, "Test Paragraph"=w1676) -> ("error out"=w1669:errorcluster)  [unwired: 8 in]
          n624 = property on="VISA Tester" class="VISAName"() -> ("Value"=w1663:refnum<visa-resource-name>)  [unwired: 2 in, 2 out]
          n625 = control-ref of="Stop Burn-in"() -> (w1666:refnum<vi>)
          n626 = control-ref of="Stop Button"() -> (w1667:refnum<vi>)
          n627 = control-ref of="Pannel User Message"() -> (w1668:refnum<vi>)
          n628 = control-ref of="ATR"() -> (w1661:refnum<vi>)
          n629 = control-ref of="Config_CANAT"() -> ()  [unwired: 1 out]
          n630 = control-ref of="Motor Speed RPM"() -> (w1665:refnum<vi>)
          n631 = while {
            shift-right: [w1688] -> _
            shift-left: enum16{"Stop", "CoolingON", "HotGunON", "Start"}."Start" -> [w1695]
            tunnel: w1669 -> [w1686]
            tunnel: w1668 -> [w1694]
            tunnel: w1667 -> [w1693]
            tunnel: w1666 -> [w1692]
            tunnel: w1665 -> [w1691]
            tunnel: w1664 -> [w1690]
            tunnel: w1663 -> [w1689]
            tunnel: w1662 -> [w1685]
            tunnel: w1661 -> [w1684]
            tunnel: w1660 -> [w1683]
            stop <- w1687 stop-if-true
            n632 = case shown="\"Start\"" w1695 {
              tunnel: w1694 -> [_ w1740 w1835 w1887]
              tunnel: w1693 -> [_ w1735 w1830 w1885]
              tunnel: w1692 -> [_ w1739 w1834 w1886]
              tunnel: w1691 -> [_ w1738 w1833 w1883]
              tunnel: w1690 -> [_ w1729 w1824 w1884]
              tunnel: w1689 -> [_ w1730 w1825 w1881]
              tunnel: [w1697 w1732 w1827 w1876] -> w1688
              tunnel: [w1696 FALSE FALSE FALSE] -> w1687
              tunnel: w1686 -> [_ w1728 w1823 _]
              tunnel: w1685 -> [_ w1723 w1818 w1877]
              tunnel: w1684 -> [_ w1719 w1815 w1879]
              tunnel: w1683 -> [_ _ _ w1888]
              frame "Stop", Default {
                n633 = flat-sequence {
                  tunnel: [enum16{"Stop", "CoolingON", "HotGunON", "Start"}."Stop"] -> w1697
                  tunnel: [TRUE] -> w1696
                  frame #0 {
                    n634 = property on="VISA Tester" class="VISAName"() -> ("Value"=w1701:refnum<visa-resource-name>)  [unwired: 2 in, 2 out]
                    n635 = call "TesterOption (SubVI).vi"("2 Options"=FALSE, "On/Off"=FALSE, "Tester Option"=T13."Venable", "VISA Refnum in"=w1701) -> ()  [unwired: 6 in, 2 out]
                  }
                  frame #1 {
                  }
                }
              }
              frame "CoolingON" {
                n636 = while {
                  tunnel: w1740 -> [w1775]
                  tunnel: w1739 -> [w1774]
                  tunnel: w1738 -> [w1770]
                  tunnel: [w1767] -> w1708
                  tunnel: w1735 -> [w1758]
                  tunnel: w1730 -> [w1744]
                  tunnel: w1729 -> [w1762]
                  tunnel: w1728 -> [w1759]
                  shift-right: [w1751] -> _
                  shift-left: 0.0 -> [w1752]
                  shift-right: [w1747] -> w1707
                  shift-left: 0.0 ("Value") -> [w1749]
                  tunnel: [w1742] -> w1711
                  stop <- w1756 stop-if-true
                  n637 = control-ref of="Power transistor Heat sink Temp."() -> (w1768:refnum<vi>)
                  n638 = property class="DigNum (strict)"(reference=w1768, error in=w1759) -> (error out=w1765:errorcluster, "Value"=w1747:dbl)  [unwired: 1 out]
                  n639 = Equal?(x=w1747, y=w1749) -> (x = y?=w1748:bool)
                  n640 = Number To Fractional String(number=w1747, precision (6)=i16 2) -> (F-format string=w1761:string)  [unwired: 2 in]
                  n641 = case shown="True" w1748 {
                    tunnel: w1752 -> [_ w1795]
                    tunnel: [0.0 w1793] -> w1751
                    tunnel: [FALSE w1792] -> w1750
                    frame False {
                    }
                    frame True {
                      n642 = Increment(x=w1795) -> (x+1=w1793:dbl)
                      n643 = Greater Or Equal?(x=w1793, y=300.0) -> (x >= y?=w1792:bool)
                    }
                  }
                  n644 = Concatenate Strings(w1762, "\nPCB Temperature [C]: " ("string"), w1761) -> (w1760:string)
                  n645 = call "Write panel message (SubVI).vi"("Stop BurnIn"=w1774, 4:"rpm"=w1770, 5:"rpm"=FALSE ("rpm"), "PrintTime"=FALSE, "Stop"=w1758, "error in (no error)"=w1765, "Time to wait"=0.2, "Strin"=w1760, "String in"=w1775) -> ("error out"=w1764:errorcluster)  [unwired: 2 in]
                  n646 = property class="Bool (strict)"(reference=w1758) -> ("Value"=w1757:bool)  [unwired: 1 in, 2 out]
                  n647 = Less Or Equal?(x=w1747, y=52.0) -> (x <= y?=w1746:bool)
                  n648 = call "GetADCTester (SubVI).vi"("error in (no error)"=w1764, "GetADCTester"=T15."Fan", "VISA Refnum in"=w1744) -> ("error out"=w1767:errorcluster, "ADCValOutput Single"=w1754:dbl)  [unwired: 6 in, 1 out]
                  n649 = Greater?(x=w1754, y=u32 2400) -> (0:w1743:bool)
                  n650 = case shown="True" w1746 {
                    tunnel: [w1782 w1789] -> w1745
                    tunnel: w1746 -> [w1782 w1789]
                    tunnel: w1744 -> [w1780 w1787]
                    tunnel: [w1776 w1783] -> w1742
                    frame False {
                      n651 = call "Time Delay11"() -> ("error out"=w1779:errorcluster)  [unwired: 11 in]
                      n652 = call "GetADCTester (SubVI).vi"("error in (no error)"=w1779, "GetADCTester"=T15."Fan", "VISA Refnum in"=w1780) -> ("ADCValOutput Single"=w1778:dbl)  [unwired: 6 in, 2 out]
                      n653 = Greater?(x=w1778, y=2400.0) -> (0:w1776:bool)
                    }
                    frame True {
                      n654 = call "Time Delay10"() -> ("error out"=w1786:errorcluster)  [unwired: 11 in]
                      n655 = call "GetADCTester (SubVI).vi"("error in (no error)"=w1786, "GetADCTester"=T15."Fan", "VISA Refnum in"=w1787) -> ("ADCValOutput Single"=w1785:dbl)  [unwired: 6 in, 2 out]
                      n656 = Greater?(x=w1785, y=2400.0) -> (0:w1783:bool)
                    }
                  }
                  n657 = Compound Arithmetic op=OR(w1743, w1757, w1745, w1750) -> (w1756:bool)
                }
                n658 = In Range and Coerce(upper limit=58.0, x=w1707, lower limit=52.0) -> (In Range?=w1710:bool)  [unwired: 1 out]
                n659 = Build Array(w1711, w1710) -> (w1712:bool[])
                n660 = And Array Elements(Boolean array=w1712) -> (logical AND=→"AuxiOFFResult":bool)
                n661 = Add(x=w1723, y=3) -> (x+y=w1721:i32)
                n662 = call "PassOrFail (SubVI).vi"("index (row)"=w1721, "error in (no error)"=w1708, "Data in"=w1707, "Pass?Fail"=w1710, "Table in"=w1719) -> ("error out"=w1725:errorcluster)  [unwired: 6 in]
                n663 = Select(t="OFF", s=w1711, f="ON") -> (s? t:f=w1715:string)
                n664 = Increment(x=w1721) -> (x+1=w1720:i32)
                n665 = call "PassOrFail (SubVI).vi"("String Res"=w1715, "index (row)"=w1720, "error in (no error)"=w1725, "Data in"=-3.0, "Pass?Fail"=w1711, "Table in"=w1719) -> ("error out"=w1724:errorcluster)  [unwired: 5 in]
                n666 = call "TesterOption (SubVI).vi"("2 Options"=FALSE, "error in (no error)"=w1724, "On/Off"=FALSE, "Tester Option"=T13."Venable" ("Tester Option 2"), "VISA Refnum in"=w1730) -> ("error out"=w1705:errorcluster)  [unwired: 5 in, 1 out]
                n667 = call "Time Delay14"("error in (no error)"=w1705) -> ("error out"=w1704:errorcluster)  [unwired: 10 in]
                n668 = property class="Bool (strict)"(reference=w1735, error in=w1704) -> ("Value"=w1741:bool)  [unwired: 2 out]
                n669 = Select(t=enum16{"Stop", "CoolingON", "HotGunON", "Start"}."Stop", s=w1741, f=enum16{"Stop", "CoolingON", "HotGunON", "Start"}."Stop") -> (s? t:f=w1732:enum16{"Stop", "CoolingON", "HotGunON", "Start"})
              }
              frame "HotGunON" {
                n670 = while {
                  tunnel: w1835 -> [w1868]
                  tunnel: w1834 -> [w1867]
                  tunnel: w1833 -> [w1863]
                  tunnel: [w1859] -> w1805
                  tunnel: w1830 -> [w1850]
                  tunnel: w1825 -> [w1860]
                  tunnel: w1824 -> [w1854]
                  tunnel: w1823 -> [w1851]
                  shift-right: [w1843] -> _
                  shift-left: 0.0 -> [w1844]
                  shift-right: [w1840] -> _
                  shift-left: 0.0 ("Value") -> [w1841]
                  tunnel: [w1838] -> w1803
                  stop <- w1848 stop-if-true
                  n671 = control-ref of="Power transistor Heat sink Temp."() -> (w1861:refnum<vi>)
                  n672 = property class="DigNum (strict)"(reference=w1861, error in=w1851) -> (error out=w1857:errorcluster, "Value"=w1840:dbl)  [unwired: 1 out]
                  n673 = Equal?(x=w1840, y=w1841) -> (x = y?=w1839:bool)
                  n674 = Number To Fractional String(number=w1840, precision (6)=i16 2) -> (F-format string=w1853:string)  [unwired: 2 in]
                  n675 = case shown="True" w1839 {
                    tunnel: w1844 -> [_ w1874]
                    tunnel: [0.0 w1872] -> w1843
                    tunnel: [FALSE w1871] -> w1842
                    frame False {
                    }
                    frame True {
                      n676 = Increment(x=w1874) -> (x+1=w1872:dbl)
                      n677 = Greater Or Equal?(x=w1872, y=300.0) -> (x >= y?=w1871:bool)
                    }
                  }
                  n678 = Concatenate Strings(w1854, "\nPCB Temperature [C]: " ("string"), w1853) -> (w1852:string)
                  n679 = call "Write panel message (SubVI).vi"("Stop BurnIn"=w1867, 4:"rpm"=w1863, 5:"rpm"=FALSE ("rpm"), "PrintTime"=FALSE, "Stop"=w1850, "error in (no error)"=w1857, "Time to wait"=0.2, "Strin"=w1852, "String in"=w1868) -> ("error out"=w1856:errorcluster)  [unwired: 2 in]
                  n680 = property class="Bool (strict)"(reference=w1850) -> ("Value"=w1849:bool)  [unwired: 1 in, 2 out]
                  n681 = call "GetADCTester (SubVI).vi"("error in (no error)"=w1856, "GetADCTester"=T15."Fan", "VISA Refnum in"=w1860) -> ("error out"=w1859:errorcluster, "ADCValOutput Single"=w1846:dbl)  [unwired: 6 in, 1 out]
                  n682 = Greater Or Equal?(x=w1840, y=61.0) -> (x >= y?=w1837:bool)
                  n683 = Less?(x=w1846, y=u32 100) -> (x < y?=w1838:bool)
                  n684 = Compound Arithmetic op=OR(w1838, w1849, w1837, w1842) -> (w1848:bool)
                }
                n685 = control-ref of="Power transistor Heat sink Temp."() -> (w1808:refnum<vi>)
                n686 = property class="DigNum (strict)"(reference=w1808, error in=w1805) -> (error out=w1807:errorcluster, "Value"=w1806:dbl)  [unwired: 1 out]
                n687 = In Range and Coerce(upper limit=62.0, x=w1806, lower limit=58.0) -> (In Range?=w1802:bool)  [unwired: 1 out]
                n688 = Build Array(w1803, w1802) -> (w1804:bool[])
                n689 = Increment(x=w1818) -> (x+1=w1817:i32)
                n690 = call "PassOrFail (SubVI).vi"("index (row)"=w1817, "error in (no error)"=w1807, "Data in"=w1806, "Pass?Fail"=w1802, "Table in"=w1815) -> ("error out"=w1820:errorcluster)  [unwired: 6 in]
                n691 = And Array Elements(Boolean array=w1804) -> (logical AND=→"AuxiONResult":bool)
                n692 = Increment(x=w1817) -> (x+1=w1816:i32)
                n693 = Select(t="ON", s=w1803, f="OFF") -> (s? t:f=w1813:string)
                n694 = call "PassOrFail (SubVI).vi"("String Res"=w1813, "index (row)"=w1816, "error in (no error)"=w1820, "Data in"=-3.0, "Pass?Fail"=w1803, "Table in"=w1815) -> ("error out"=w1819:errorcluster)  [unwired: 5 in]
                n695 = call "TesterOption (SubVI).vi"("On/Off 2"=FALSE, "Tester Option 2"=T13."Venable", "2 Options"=TRUE, "error in (no error)"=w1819, "On/Off"=FALSE, "Tester Option"=T13."Fan", "VISA Refnum in"=w1825) -> ("error out"=w1797:errorcluster)  [unwired: 3 in, 1 out]
                n696 = call "Time Delay13"("error in (no error)"=w1797) -> ("error out"=w1796:errorcluster)  [unwired: 10 in]
                n697 = property class="Bool (strict)"(reference=w1830, error in=w1796) -> ("Value"=w1836:bool)  [unwired: 2 out]
                n698 = Select(t=enum16{"Stop", "CoolingON", "HotGunON", "Start"}."Stop", s=w1836, f=enum16{"Stop", "CoolingON", "HotGunON", "Start"}."CoolingON") -> (s? t:f=w1827:enum16{"Stop", "CoolingON", "HotGunON", "Start"})
              }
              frame "Start" {
                n699 = call "Write panel message (SubVI).vi"("Stop BurnIn"=w1886, 4:"rpm"=w1883, 5:"rpm"=FALSE ("rpm"), "PrintTime"=FALSE, "Stop"=w1885, "Time to wait"=1.0, "Strin"=w1884, "String in"=w1887) -> ("error out"=w1894:errorcluster)  [unwired: 3 in]
                n700 = call "TesterOption (SubVI).vi"("2 Options"=FALSE, "error in (no error)"=w1894, "On/Off"=FALSE, "Tester Option"=T13."Venable", "VISA Refnum in"=w1881) -> ("error out"=w1889:errorcluster)  [unwired: 5 in, 1 out]
                n701 = while {
                  tunnel: w1889 -> [w1915]
                  tunnel: w1888 -> [w1914]
                  tunnel: w1887 -> [w1913]
                  tunnel: w1886 -> [w1912]
                  tunnel: w1885 -> [w1911]
                  tunnel: w1884 -> [w1910]
                  tunnel: w1883 -> [w1909]
                  shift-right: [w1906] -> _
                  shift-left: enum16{"Wait", "OFF", "ON", "Start"}."Start" -> [w1908]
                  tunnel: w1881 -> [w1907]
                  shift-right: [w1904] -> _
                  shift-left: 0 -> [w1905]
                  tunnel: w1879 -> [w1902]
                  shift-right: [w1901] -> w1875
                  shift-left: TRUE -> [w1900]
                  tunnel: w1877 -> [w1899]
                  stop <- w1903 stop-if-true
                  n702 = case shown="\"Start\"" w1908 {
                    tunnel: w1915 -> [_ w1962 _ w2025]
                    tunnel: w1914 -> [w1930 w1961 _ w2024]
                    tunnel: w1913 -> [_ w1959 _ w2022]
                    tunnel: w1912 -> [_ w1958 _ w2021]
                    tunnel: w1911 -> [_ w1937 _ w2005]
                    tunnel: w1910 -> [_ w1957 _ w2020]
                    tunnel: w1909 -> [_ w1956 _ w2019]
                    tunnel: w1907 -> [_ w1949 _ w2012]
                    tunnel: [w1933 w1939 enum16{"Wait", "OFF", "ON", "Start"}."OFF" w2002] -> w1906
                    tunnel: w1905 -> [w1934 w1947 _ w2010]
                    tunnel: [w1934 w1946 0 w2009] -> w1904
                    tunnel: [w1932 FALSE FALSE FALSE] -> w1903
                    tunnel: w1902 -> [w1918 _ w1998 _]
                    tunnel: [FALSE w1943 TRUE w2006] -> w1901
                    tunnel: w1900 -> [w1921 _ w1999 _]
                    tunnel: w1899 -> [w1920 _ w1997 _]
                    frame "Wait", Default {
                      n703 = call "SerialMarvinSendGet.vi"("write buffer"="EP=1\r\nAU=0\r\n", "VISA resource name"=w1930) -> ("error out"=w1929:errorcluster)  [unwired: 8 in, 1 out]
                      n704 = call "Time Delay19"("error in (no error)"=w1929) -> ("error out"=w1917:errorcluster)  [unwired: 10 in]
                      n705 = Not(x=w1921) -> (.not. x?=w1923:bool)
                      n706 = Select(t="OFF", s=w1923, f="ON") -> (s? t:f=w1922:string)
                      n707 = Add(x=2, y=w1920) -> (x+y=w1927:i32)
                      n708 = call "PassOrFail (SubVI).vi"("String Res"=w1922, "index (row)"=w1927, "error in (no error)"=w1917, "Data in"=-3.0, "Pass?Fail"=w1923, "Table in"=w1918) -> ("error out"=w1916:errorcluster)  [unwired: 5 in]
                      n709 = flat-sequence {
                        tunnel: [enum16{"Wait", "OFF", "ON", "Start"}."Wait"] -> w1933
                        tunnel: [TRUE] -> w1932
                        tunnel: w1916 -> [_]
                        frame #0 {
                        }
                      }
                    }
                    frame "OFF" {
                      n710 = call "SerialMarvinSendGet.vi"("error in (no error)"=w1962, "write buffer"="EP=1\r\nAU=0\r\n", "VISA resource name"=w1961) -> ("error out"=w1951:errorcluster)  [unwired: 7 in, 1 out]
                      n711 = call "Time Delay"("error in (no error)"=w1951) -> ("error out"=w1945:errorcluster)  [unwired: 10 in]
                      n712 = call "GetADCTester (SubVI).vi"("error in (no error)"=w1945, "GetADCTester"=T15."Fan", "TimeToGet"=5, "VISA Refnum in"=w1949) -> ("error out"=w1950:errorcluster, "ADCValOutput Single"=w1953:dbl)  [unwired: 5 in, 1 out]
                      n713 = Greater?(x=w1953, y=2400.0) -> (0:w1948:bool)
                      n714 = case shown="True" w1948 {
                        tunnel: w1959 -> [_ w1981]
                        tunnel: w1958 -> [_ w1980]
                        tunnel: w1937 -> [_ w1979]
                        tunnel: w1957 -> [_ w1978]
                        tunnel: w1956 -> [_ w1977]
                        tunnel: w1950 -> [w1964 w1976]
                        tunnel: [w1965 w1974] -> w1938
                        tunnel: w1947 -> [w1969 _]
                        tunnel: [w1970 0] -> w1946
                        tunnel: [w1964 w1972] -> w1940
                        tunnel: [w1963 FALSE] -> w1943
                        frame False {
                          n715 = Increment(x=w1969) -> (x+1=w1970:i32)
                          n716 = Greater Or Equal?(x=w1969, y=10) -> (x >= y?=w1963:bool)
                          n717 = Select(t=enum16{"Wait", "OFF", "ON", "Start"}."Wait", s=w1963, f=enum16{"Wait", "OFF", "ON", "Start"}."OFF") -> (s? t:f=w1965:enum16{"Wait", "OFF", "ON", "Start"})
                        }
                        frame True {
                          n718 = call "Write panel message (SubVI).vi"("Stop BurnIn"=w1980, 4:"rpm"=w1977, 5:"rpm"=FALSE ("rpm"), "PrintTime"=TRUE, "Stop"=w1979, "error in (no error)"=w1976, "Time to wait"=5.0, "Strin"=w1978, "String in"=w1981) -> ("error out"=w1975:errorcluster)  [unwired: 2 in]
                          n719 = flat-sequence {
                            tunnel: w1975 -> [w1985]
                            tunnel: [enum16{"Wait", "OFF", "ON", "Start"}."Wait"] -> w1974
                            tunnel: [w1985] -> w1972
                            frame #0 {
                            }
                          }
                        }
                      }
                      n720 = property class="Bool (strict)"(reference=w1937, error in=w1940) -> ("Value"=w1942:bool)  [unwired: 2 out]
                      n721 = Select(t=enum16{"Wait", "OFF", "ON", "Start"}."Wait", s=w1942, f=w1938) -> (s? t:f=w1939:enum16{"Wait", "OFF", "ON", "Start"})
                    }
                    frame "ON" {
                      n722 = Not(x=w1999) -> (.not. x?=w1992:bool)
                      n723 = Select(t="ON", s=w1992, f="OFF") -> (s? t:f=w1991:string)
                      n724 = Increment(x=w1997) -> (x+1=w1996:i32)
                      n725 = call "PassOrFail (SubVI).vi"("String Res"=w1991, "index (row)"=w1996, "Data in"=-3.0, "Pass?Fail"=w1992, "Table in"=w1998) -> ()  [unwired: 6 in, 1 out]
                    }
                    frame "Start" {
                      n726 = call "SerialMarvinSendGet.vi"("error in (no error)"=w2025, "write buffer"="EP=1\r\nAU=1\r\n", "VISA resource name"=w2024) -> ("error out"=w2014:errorcluster)  [unwired: 7 in, 1 out]
                      n727 = call "Time Delay18"("error in (no error)"=w2014) -> ("error out"=w2008:errorcluster)  [unwired: 10 in]
                      n728 = call "GetADCTester (SubVI).vi"("error in (no error)"=w2008, "GetADCTester"=T15."Fan", "TimeToGet"=5, "VISA Refnum in"=w2012) -> ("error out"=w2013:errorcluster, "ADCValOutput Single"=w2016:dbl)  [unwired: 5 in, 1 out]
                      n729 = Less?(x=w2016, y=100.0) -> (x < y?=w2011:bool)
                      n730 = case shown="False" w2011 {
                        tunnel: w2022 -> [_ w2044]
                        tunnel: w2021 -> [_ w2043]
                        tunnel: w2005 -> [_ w2042]
                        tunnel: w2020 -> [_ w2041]
                        tunnel: w2019 -> [_ w2040]
                        tunnel: w2013 -> [w2027 w2039]
                        tunnel: [w2028 w2037] -> w2003
                        tunnel: w2010 -> [w2032 _]
                        tunnel: [w2033 0] -> w2009
                        tunnel: [w2027 w2035] -> w2000
                        tunnel: [w2026 FALSE] -> w2006
                        frame False {
                          n731 = Increment(x=w2032) -> (x+1=w2033:i32)
                          n732 = Greater Or Equal?(x=w2032, y=5) -> (x >= y?=w2026:bool)
                          n733 = Select(t=enum16{"Wait", "OFF", "ON", "Start"}."ON", s=w2026, f=enum16{"Wait", "OFF", "ON", "Start"}."Start") -> (s? t:f=w2028:enum16{"Wait", "OFF", "ON", "Start"})
                        }
                        frame True {
                          n734 = call "Write panel message (SubVI).vi"("Stop BurnIn"=w2043, 4:"rpm"=w2040, 5:"rpm"=FALSE ("rpm"), "PrintTime"=TRUE, "Stop"=w2042, "error in (no error)"=w2039, "Time to wait"=60.0, "Strin"=w2041, "String in"=w2044) -> ("error out"=w2038:errorcluster)  [unwired: 2 in]
                          n735 = flat-sequence {
                            tunnel: w2038 -> [w2048]
                            tunnel: [enum16{"Wait", "OFF", "ON", "Start"}."ON"] -> w2037
                            tunnel: [w2048] -> w2035
                            frame #0 {
                            }
                          }
                        }
                      }
                      n736 = property class="Bool (strict)"(reference=w2005, error in=w2000) -> ("Value"=w2004:bool)  [unwired: 2 out]
                      n737 = Select(t=enum16{"Wait", "OFF", "ON", "Start"}."Wait", s=w2004, f=w2003) -> (s? t:f=w2002:enum16{"Wait", "OFF", "ON", "Start"})
                    }
                  }
                }
                n738 = flat-sequence {
                  tunnel: [enum16{"Stop", "CoolingON", "HotGunON", "Start"}."Stop"] -> w1876
                  tunnel: w1875 -> [_]
                  frame #0 {
                  }
                }
              }
            }
          }
        }
      }
      "CurrentTest" <- w229
    }
    n739 = flat-sequence {
      tunnel: w216 -> [_]
      frame #0 {
        w224 = T21."Enabled" ("Disabled")
        w225 = FALSE ("Start")
        n740 = property on="Start" class="Bool (strict)"("Value"=w225, "DisabledEnum"=w224) -> ()  [unwired: 2 in, 2 out]
        n741 = property on="Report" class="Bool (strict)"("Value"=w225, "DisabledEnum"=w224) -> ()  [unwired: 2 in, 2 out]
      }
    }
  }
  n742 = while {
    shift-right: [w2054] -> _
    shift-left: T11."Initialize" -> [w2073]
    shift-right: [w2070] -> _
    shift-left: _ -> [w2069]
    shift-right: [w2068] -> _
    shift-left: w33 -> [w2066]
    shift-right: [w2067] -> _
    shift-left: refnum<vi> refnum ("Config_CANAT") -> [w2065]
    shift-right: [w2063] -> _
    shift-left: w30 -> [w2064]
    tunnel: "ATR" -> [_]
    tunnel: w22 -> [w2062]
    tunnel: w21 -> [w2061]
    shift-right: [w2059] -> _
    shift-left: w1 -> [w2060]
    tunnel: w8 -> [w2058]
    tunnel: w2 -> [w2057]
    tunnel: w19 -> [_]
    tunnel: w31 -> [w2072]
    tunnel: [w2071] -> _
    tunnel: w9 -> [_]
    tunnel: w6 -> [w2055]
    shift-right: [w2052] -> _
    shift-left: w1 -> [w2053]
    shift-right: [w2050] -> _
    shift-left: w1 -> [w2051]
    stop <- w2056 stop-if-true
    n743 = case shown="\"Erase ATR Table\", Default" w2073 {
      tunnel: [w2080 w2223 w2298 T11."Erase ATR Table"] -> w2054
      tunnel: [FALSE w2209 FALSE FALSE] -> w2056
      tunnel: [w2076 w2214 w2292 w3250] -> w2071
      tunnel: w2072 -> [_ w2234 w2296 _]
      tunnel: [w2116 refnum<visa-resource-name> refnum ("VISA resource name") w2293 w3254] -> w2070
      tunnel: w2069 -> [w2116 w2242 w2294 _]
      tunnel: [w2107 w2203 w2288 w3248] -> w2068
      tunnel: [w2106 refnum<vi> refnum ("Config_CANAT") w2289 w3251] -> w2067
      tunnel: w2066 -> [w2107 w2244 w2291 w3248]
      tunnel: w2065 -> [w2106 w2226 w2290 _]
      tunnel: w2064 -> [w2105 w2237 w2287 w3247]
      tunnel: [w2105 w2202 w2286 w3247] -> w2063
      tunnel: w2062 -> [_ _ w2285 _]
      tunnel: w2061 -> [_ _ w2284 _]
      tunnel: w2060 -> [w2102 w2228 w2283 w3244]
      tunnel: [w2102 w2228 w2282 w3244] -> w2059
      tunnel: w2058 -> [w2092 _ w2281 _]
      tunnel: w2057 -> [_ _ w2280 _]
      tunnel: w2055 -> [_ _ w2279 _]
      tunnel: w2053 -> [_ _ w2278 _]
      tunnel: [w2074 w2201 w2277 w3235] -> w2052
      tunnel: w2051 -> [_ _ w2276 _]
      tunnel: [w2074 w2201 w2275 w3235] -> w2050
      frame "Erase ATR Table", Default {
        w2074 = 0
        w2084 = T21."Enabled" ("Disabled")
        w2096 = "Marvin" ("section")
        w2103 = refnum<visa-resource-name> "COM4" ("VISA resource name")
        w2112 = FALSE ("Visible")
        n744 = property on="Serial Com" class="Bool"(error in=errorcluster {"status"=FALSE, "code"=0, "source"=""} ("error out"), "Visible"=TRUE) -> (error out=w2104:errorcluster)  [unwired: 1 in, 1 out]
        n745 = property on="VISA Marvin" class="VISAName"(error in=w2104, "Visible"=w2112, "Value"=w2103) -> (error out=w2114:errorcluster)  [unwired: 1 in, 1 out]
        n746 = property on="VISA Marvin" class="VISAName"(error in=w2104, "Value"=w2103) -> ()  [unwired: 1 in, 2 out]
        n747 = property on="Status" class="Bool (strict)"(error in=w2114, "Value"=w2112) -> (error out=w2087:errorcluster)  [unwired: 1 in, 1 out]
        n748 = call "Select UUT"("error in (no error)"=w2087) -> ("EBAY"=w2085:bool, "error out"=w2086:errorcluster)  [unwired: 17 in]
        n749 = case shown="False" w2085 {
          tunnel: [string[][] [["1", "Communication Test", "", "", "", "", ""], ["1.1", "Serial RS-232", "N/A", "-", "", "", ""], ["1.2", "CAN Bus", "N/A", "-", "", "", ""], ["", "", "", "", "", "", ""], ["2", "Temperature Sensor Calibration", "", "", "", "", ""], ["2.1", "Sensor Reading Analog Offset", "0", "+/-0.100", ".", "", ""], ["", "", "", "", "", "", ""], ["3", "Motor Termistor Input Test", "", "", "", "", ""], ["3.1", "60 Degree", "60", "+/-3.00", "°C", "", ""], ["3.2", "90 Degree", "90", "+/-3.00", "°C", "", ""], ["3.3", "120 Degree", "120", "+/-3.00", "°C", "", ""], ["", "", "", "", "", "", ""], ["4", "Enable Test", "", "", "", "", ""], ["4.1", "Fan Speed at Opened Enable ", "5000", "+/-200.0", "rpm", "", ""], ["4.2", "Fan Speed at Opened Enable ", "0", "+/-200.0", "rpm", "", ""], ["4.3", "Fan Speed at Closed Enable ", "5000", "+/-200.0", "rpm", "", ""], ["4.4", "Motor Rotation Direction", "CCW", "-", "", "", ""], ["", "", "", "", "", "", ""], ["5", "Speed Command Test", "", "", "", "", ""], ["5.1", "Fan  Speed", "6000", "+/-200.0", "rpm", "", ""], ["5.2", "Fan  Speed", "9000", "+/-200.0", "rpm", "", ""], ["5.3", "Fan  Speed", "12100", "+/-200.0", "rpm", "", ""], ["", "", "", "", "", "", ""], ["6", "Motor Stop time", "< 50", "-", "sec", "", ""], ["", "", "", "", "", "", ""], ["7", "Burn-in Test", "", "", "", "", ""], ["7.1", "DC Input Current", "28", "+/-5.000", "A", "", ""], ["7.2", "Fan speed", "12100", "+/-200.0", "rpm", "", ""], ["7.3", "Ambient Temperature", "25", "+/-13.00", "°C", "", ""], ["7.4", "After 10 min of operation", "", "-", "°C", "", ""], ["7.5", "After 20 min of operation", "", "-", "°C", "", ""], ["7.6", "After 30 min of operation", "", "-", "°C", "", ""], ["", "", "", "", "", "", ""], ["8", "Visual Inspection", "", "", "", "", ""], ["8.1", "Verification of Components Not Installed", "N/A", "-", "", "", ""], ["8.2", "Manufacturing Defects", "N/A", "-", "", "", ""], ["", "", "", "", "", "", ""], ["9", "Power Supply Testing", "", "", "", "", ""], ["9.1", "DC Input Current Drawn", "150", "+/-10.00", "mA", "", ""], ["", "", "", "", "", "", ""], ["10", "Power Supply Voltages", "", "", "", "", ""], ["10.1", "12V", "12.0", "+/-0.500", "V", "", ""], ["10.2", "5V", "5.0", "+/-0.200", "V", "", ""], ["10.3", "3.3V", "3.3", "+/-0.100", "V", "", ""], ["10.4", "1.8V", "1.8", "+/-0.100", "V", "", ""], ["", "", "", "", "", "", ""], ["11", "Reverse Polarity Test - DC Input Current", "< 1", "-", "mA", "", ""], ["", "", "", "", "", "", ""], ["12", "Functional Test Procedure", "", "", "", "", ""], ["12.1", "Weight Check", "3800", "+/-100.0", "gr", "", ""], ["", "", "", "", "", "", ""], ["13", "Insulation Resistance Test", "", "", "", "", ""], ["13.1", "J3.B to Chassis", "> 1M", "-", "ohms", "", ""], ["13.2", "J1.16 to Chassis", "> 100K", "-", "ohms", "", ""], ["", "", "", "", "", "", ""], ["14", "Bonding Resistance", "", "", "", "", ""], ["14.1", "J1 Body to Chassis", "< 2m", "-", "ohms", "", ""], ["14.2", "J2  Body to Chassis", "< 2m", "-", "ohms", "", ""], ["14.3", "J3  Body to Chassis", "< 2m", "-", "ohms", "", ""], ["", "", "", "", "", "", ""], ["15", "CANbus Resistance Test", "", "", "", "", ""], ["15.1", "J1.17 to J1.18", "> 10K", "-", "ohms", "", ""], ["", "", "", "", "", "", ""], ["16", "Sealing Test", "N/A", "-", "", "", ""], ["", "", "", "", "", "", ""], ["17", "Mounting Holes Test - Jig Fit", "214", "-", "mm", "", ""]] ("ArrAHU 2") string[][] [["1", "Communication Test", "", "", "", "", ""], ["1.1", "Serial RS-232", "N/A", "-", "", "", ""], ["1.2", "CAN Bus", "N/A", "-", "", "", ""], ["", "", "", "", "", "", ""], ["2", "Auxiliary Fan Test", "", "", "", "", ""], ["2.1", "Fan status-ON", "ON", "-", "-", "", ""], ["2.2", "Fan status-OFF", "OFF", "-", "-", "", ""], ["", "", "", "", "", "", ""], ["3", "Temperature Sensor Calibration", "", "", "", "", ""], ["3.1", "Sensor Reading Analog Offset", "0", "+/-0.100", ".", "", ""], ["", "", "", "", "", "", ""], ["4", "Motor Termistor Input Test", "", "", "", "", ""], ["4.1", "60 Degree", "60", "+/-3.00", "°C", "", ""], ["4.2", "90 Degree", "90", "+/-3.00", "°C", "", ""], ["4.3", "120 Degree", "120", "+/-3.00", "°C", "", ""], ["", "", "", "", "", "", ""], ["5", "Enable Test", "", "", "", "", ""], ["5.1", "Fan Speed at Opened Enable ", "5000", "+/-200.0", "rpm", "", ""], ["5.2", "Fan Speed at Opened Enable ", "0", "+/-200.0", "rpm", "", ""], ["5.3", "Fan Speed at Closed Enable ", "5000", "+/-200.0", "rpm", "", ""], ["5.4", "Motor Rotation Direction", "CCW", "-", "", "", ""], ["", "", "", "", "", "", ""], ["6", "Speed Command Test", "", "", "", "", ""], ["6.1", "Fan  Speed", "11500", "+/-200.0", "rpm", "", ""], ["6.2", "Fan  Speed", "12700", "+/-200.0", "rpm", "", ""], ["6.3", "Fan  Speed", "14700", "+/-200.0", "rpm", "", ""], ["", "", "", "", "", "", ""], ["7", "Motor Stop time", "< 50", "-", "sec", "", ""], ["", "", "", "", "", "", ""], ["8", "Temperature Control Algorithm Test", "", "", "", "", ""], ["8.1", "Tair <   67 ± 3 °C", "11500", "+/-200.0", "rpm", "", ""], ["8.2", "Measured Temp.", "", "", "°C", "", ""], ["8.3", "Tair >= 67 ± 3 °C", "12700", "+/-200.0", "rpm", "", ""], ["8.4", "Transition Temp.", "", "", "°C", "", ""], ["8.5", "Tair >= 83 ± 3 °C", "14700", "+/-400.0", "rpm", "", ""], ["8.6", "Transition Temp.", "", "", "°C", "", ""], ["8.7", "Tair <= 80 ± 3 °C", "12700", "+/-200.0", "rpm", "", ""], ["8.8", "Transition Temp.", "", "", "°C", "", ""], ["8.9", "Tair <= 64 ± 3 °C", "11500", "+/-200.0", "rpm", "", ""], ["8.10", "Transition Temp.", "", "", "°C", "", ""], ["", "", "", "", "", "", ""], ["9", "Burn-in Test", "", "", "", "", ""], ["9.1", "DC Input Current", "45", "+/-5.000", "A", "", ""], ["9.2", "Fan speed", "14700", "+/-200.0", "rpm", "", ""], ["9.3", "Ambient Temperature", "25", "+/-13.00", "°C", "", ""], ["9.4", "After 10 min of operation", "", "-", "°C", "", ""], ["9.5", "After 20 min of operation", "", "-", "°C", "", ""], ["9.6", "After 30 min of operation", "", "-", "°C", "", ""], ["", "", "", "", "", "", ""], ["10", "Visual Inspection", "", "", "", "", ""], ["10.1", "Verification of Components Not Installed", "N/A", "-", "", "", ""], ["10.2", "Manufacturing Defects", "N/A", "-", "", "", ""], ["", "", "", "", "", "", ""], ["11", "Power Supply Testing", "", "", "", "", ""], ["11.1", "DC Input Current Drawn", "150", "+/-10.00", "mA", "", ""], ["", "", "", "", "", "", ""], ["12", "Power Supply Voltages", "", "", "", "", ""], ["12.1", "12V", "12.0", "+/-0.500", "V", "", ""], ["12.2", "5V", "5.0", "+/-0.200", "V", "", ""], ["12.3", "3.3V", "3.3", "+/-0.100", "V", "", ""], ["12.4", "1.8V", "1.8", "+/-0.100", "V", "", ""], ["", "", "", "", "", "", ""], ["13", "Reverse Polarity Test - DC Input Current", "< 1", "-", "mA", "", ""], ["", "", "", "", "", "", ""], ["14", "Functional Test Procedure", "", "", "", "", ""], ["14.1", "Weight Check", "4180", "+/-100.0", "gr", "", ""], ["", "", "", "", "", "", ""], ["15", "Insulation Resistance Test", "", "", "", "", ""], ["15.1", "J3.B to Chassis", "> 1M", "-", "ohms", "", ""], ["15.2", "J1.16 to Chassis", "> 100K", "-", "ohms", "", ""], ["", "", "", "", "", "", ""], ["16", "Bonding Resistance", "", "", "", "", ""], ["16.1", "J1 Body to Chassis", "< 2m", "-", "ohms", "", ""], ["16.2", "J2  Body to Chassis", "< 2m", "-", "ohms", "", ""], ["16.3", "J3  Body to Chassis", "< 2m", "-", "ohms", "", ""], ["", "", "", "", "", "", ""], ["17", "CANbus Resistance Test", "", "", "", "", ""], ["17.1", "J1.17 to J1.18", "> 10K", "-", "ohms", "", ""], ["", "", "", "", "", "", ""], ["18", "Sealing Test", "N/A", "-", "", "", ""], ["", "", "", "", "", "", ""], ["19", "Mounting Holes Test - Jig Fit", "214", "-", "mm", "", ""]] ("ArrEbay 3")] -> w2110
          tunnel: ["AHU" "EBAY"] -> w2109
          tunnel: [w2173 w2185] -> w2108
          tunnel: w2086 -> [w2174 w2185]
          tunnel: [w2169 u8 95] -> w2081
          frame False {
            (unwired) string[][] [["6.1", "Visual Inspection", "", "", "", "", ""], ["6.1.1", "Verification of Components Not Installed", "N/A", "-", "", "", ""], ["", "", "", "", "", "", ""], ["6.1.2", "Manufacturing Defects", "N/A", "-", "", "", ""], ["", "", "", "", "", "", ""], ["6.2", "Power Supply Testing", "", "", "", "", ""], ["6.2.1", "Input Current Drawn", "", "", "", "", ""], ["6.2.1.1", "DC Input Current", "< 150", "-", "mA", "", ""], ["", "", "", "", "", "", ""], ["6.2.2", "Power Supply Voltages", "", "", "", "", ""], ["6.2.2.1", "12V", "12.0", "+/-0.500", "V", "", ""], ["6.2.2.2", "5V", "5.0", "+/-0.200", "V", "", ""], ["6.2.2.3", "3.3V", "3.3", "+/-0.100", "V", "", ""], ["6.2.2.4", "1.8V", "1.8", "+/-0.100", "V", "", ""], ["", "", "", "", "", "", ""], ["7", "Functional Test Procedure", "", "", "", "", ""], ["7.1", "Weight Check", "3800", "+/-100.0", "gr", "", ""], ["", "", "", "", "", "", ""], ["7.2", "Insulation Resistance Test", "", "", "", "", ""], ["7.2.1", "J3.B to Chassis", "> 1M", "-", "W", "", ""], ["7.2.2", "J1.16 to Chassis", "> 100K", "-", "W", "", ""], ["", "", "", "", "", "", ""], ["7.2", "Bonding Resistance", "", "", "", "", ""], ["7.2.3", "J1 Body to Chassis", "< 2m", "-", "W", "", ""], ["7.2.4", "J2  Body to Chassis", "< 2m", "-", "W", "", ""], ["7.2.5", "J3  Body to Chassis", "< 2m", "-", "W", "", ""], ["", "", "", "", "", "", ""], ["7.2.1", "CANbus Resistance Test", "", "", "", "", ""], ["7.2.1.1", "J1.17 to J1.18", "> 10K", "-", "W", "", ""], ["", "", "", "", "", "", ""], ["7.3", "Sealing Test", "N/A", "-", "", "", ""], ["", "", "", "", "", "", ""], ["7.4", "Communication Test", "", "", "", "", ""], ["7.4.1", "Serial RS-232", "N/A", "-", "", "", ""], ["7.4.2", "CAN Bus", "N/A", "-", "", "", ""], ["", "", "", "", "", "", ""], ["7.5", "Performances Tests", "", "", "", "", ""], ["7.5.1", "Reverse Polarity Test", "", "", "", "", ""], ["7.5.1.1", "DC Input Current", "< 1", "-", "mA", "", ""], ["", "", "", "", "", "", ""], ["7.5.2", "Enable Test", "", "", "", "", ""], ["7.5.2.1", "Fan Speed at Opened Enable ", "5000", "+/-200.0", "rpm", "", ""], ["7.5.2.2", "Fan Speed at Opened Enable ", "0", "+/-200.0", "rpm", "", ""], ["7.5.2.3", "Fan Speed at Closed Enable ", "5000", "+/-200.0", "rpm", "", ""], ["7.5.2.4", "Motor Rotation Direction", "Counter-clockwise (Inlet)", "-", "", "", ""], ["", "", "", "", "", "", ""], ["7.5.3", "Stop Time Test ", "", "", "", "", ""], ["7.5.3.1", "Motor Stop time", "< 50", "-", "sec", "", ""], ["", "", "", "", "", "", ""], ["7.5.4", "Speed Command Test", "", "", "", "", ""], ["7.5.4.1", "Fan Speed", "6000", "+/-200.0", "rpm", "", ""], ["7.5.4.2", "Fan Speed", "9000", "+/-200.0", "rpm", "", ""], ["7.5.4.3", "Fan Speed", "12100", "+/-200.0", "rpm", "", ""], ["", "", "", "", "", "", ""], ["7.5.5", "Temperature Sensor Calibration Test", "", "", "", "", ""], ["7.5.5.1", "Sensor Reading Analog Offset", "0", "+/-0.100", ".", "", ""], ["", "", "", "", "", "", ""], ["7.5.6", "Burn-in Test", "", "", "", "", ""], ["7.5.6.1", "DC Input Current", "28", "+/-3.000", "A", "", ""], ["7.5.6.2", "Fan Speed", "12100", "+/-200.000", "rpm", "", ""], ["7.5.6.3", "Ambient Temperature", "25", "+/-13.00", "C", "", ""], ["7.5.6.4", "After 10 min of operation", "", "", "C", "", ""], ["7.5.6.5", "After 20 min of operation", "", "", "C", "", ""], ["7.5.6.6", "After 30 min of operation", "", "", "C", "", ""], ["", "", "", "", "", "", ""], ["9", "Motor Temp Test", "", "", "", "", ""], ["9.1", "60 C", "60", "+/-3.000", "C", "", ""], ["9.2", "90 C", "90", "+/-3.000", "C", "", ""], ["9.3", "120 C", "120", "+/-3.000", "C", "", ""]] ("data")
            n750 = while {
              shift-right: [w2181] -> w2173
              shift-left: w2174 -> [w2182]
              tunnel: [w2176] -> w2172
              stop <- w2180 stop-if-true
              n751 = call "AHU UUT (subVI).vi"("error in (no error)"=w2182) -> ("AHU 47"=w2177:bool, "AHU 63"=w2176:bool, "OK"=w2179:bool, "error out"=w2181:errorcluster)  [unwired: 15 in]
              n752 = Exclusive Or(1:w2177, 2:w2176) -> (0:w2178:bool)
              n753 = And(x=w2179, y=w2178) -> (x .and. y?=w2180:bool)
            }
            n754 = Select(t=u8 63, s=w2172, f=u8 47) -> (s? t:f=w2169:u8)
          }
          frame True {
            (unwired) string[][] [["1", "Communication Test", "", "", "", "", ""], ["1.1", "Serial RS-232", "N/A", "-", "", "", ""], ["1.2", "CAN Bus", "N/A", "-", "", "", ""], ["", "", "", "", "", "", ""], ["2", "Temperature Sensor Calibration", "", "", "", "", ""], ["2.1", "Sensor Reading Analog Offset", "0", "+/-0.100", ".", "", ""], ["", "", "", "", "", "", ""], ["3", "Motor Termistor Input Test", "", "", "", "", ""], ["3.1", "60 Degree", "60", "+/-3.00", "°C", "", ""], ["3.2", "90 Degree", "90", "+/-3.00", "°C", "", ""], ["3.3", "120 Degree", "120", "+/-3.00", "°C", "", ""], ["", "", "", "", "", "", ""], ["4", "Enable Test", "", "", "", "", ""], ["4.1", "Fan Speed at Opened Enable ", "5000", "+/-200.0", "rpm", "", ""], ["4.2", "Fan Speed at Opened Enable ", "0", "+/-200.0", "rpm", "", ""], ["4.3", "Fan Speed at Closed Enable ", "5000", "+/-200.0", "rpm", "", ""], ["4.4", "Motor Rotation Direction", "CCW", "-", "", "", ""], ["", "", "", "", "", "", ""], ["5", "Speed Command Test", "", "", "", "", ""], ["5.1", "Fan Speed", "11500", "+/-200.0", "rpm", "", ""], ["5.2", "Fan Speed", "12700", "+/-200.0", "rpm", "", ""], ["5.3", "Fan Speed", "14700", "+/-200.0", "rpm", "", ""], ["", "", "", "", "", "", ""], ["6", "Motor Stop time", "< 50", "-", "sec", "", ""], ["", "", "", "", "", "", ""], ["7", "Temperature Control Algorithm Test", "", "", "", "", ""], ["7.1", "Tair <   67 ± 3 °C", "11500", "+/-200.0", "rpm", "", ""], ["7.2", "Measured Temp.", "", "", "°C", "", ""], ["7.3", "Tair >= 67 ± 3 °C", "12700", "+/-200.0", "rpm", "", ""], ["7.4", "Transition Temp.", "", "", "°C", "", ""], ["7.5", "Tair >= 83 ± 3 °C", "14700", "+/-400.0", "rpm", "", ""], ["7.6", "Transition Temp.", "", "", "°C", "", ""], ["7.7", "Tair <= 80 ± 3 °C", "12700", "+/-200.0", "rpm", "", ""], ["7.8", "Transition Temp.", "", "", "°C", "", ""], ["7.9", "Tair <= 64 ± 3 °C", "11500", "+/-200.0", "rpm", "", ""], ["7.10", "Transition Temp.", "", "", "°C", "", ""], ["", "", "", "", "", "", ""], ["8", "Burn-in Test", "", "", "", "", ""], ["8.1", "DC Input Current", "50", "+/-5.000", "A", "", ""], ["8.2", "Fan Speed", "14700", "+/-200.0", "rpm", "", ""], ["8.3", "Ambient Temperature", "25", "+/-13.00", "°C", "", ""], ["8.4", "After 10 min of operation", "", "-", "°C", "", ""], ["8.5", "After 20 min of operation", "", "-", "°C", "", ""], ["8.6", "After 30 min of operation", "", "-", "°C", "", ""], ["", "", "", "", "", "", ""], ["9", "Auxiliary Fan Test", "", "", "", "", ""], ["9.1", "Fan status-ON", "ON", "-", "-", "", ""], ["9.2", "Fan status-OFF", "OFF", "-", "-", "", ""], ["", "", "", "", "", "", ""], ["10", "Visual Inspection", "", "", "", "", ""], ["10.1", "Verification of Components Not Installed", "N/A", "-", "", "", ""], ["10.2", "Manufacturing Defects", "N/A", "-", "", "", ""], ["", "", "", "", "", "", ""], ["11", "Power Supply Testing", "", "", "", "", ""], ["11.1", "DC Input Current Drawn", "150", "+/-10.00", "mA", "", ""], ["", "", "", "", "", "", ""], ["12", "Power Supply Voltages", "", "", "", "", ""], ["12.1", "12V", "12.0", "+/-0.500", "V", "", ""], ["12.2", "5V", "5.0", "+/-0.200", "V", "", ""], ["12.3", "3.3V", "3.3", "+/-0.100", "V", "", ""], ["12.4", "1.8V", "1.8", "+/-0.100", "V", "", ""], ["", "", "", "", "", "", ""], ["13", "Reverse Polarity Test - DC Input Current", "< 1", "-", "mA", "", ""], ["", "", "", "", "", "", ""], ["14", "Functional Test Procedure", "", "", "", "", ""], ["14.1", "Weight Check", "4180", "+/-100.0", "gr", "", ""], ["", "", "", "", "", "", ""], ["15", "Insulation Resistance Test", "", "", "", "", ""], ["15.1", "J3.B to Chassis", "> 1M", "-", "ohms", "", ""], ["15.2", "J1.16 to Chassis", "> 100K", "-", "ohms", "", ""], ["", "", "", "", "", "", ""], ["16", "Bonding Resistance", "", "", "", "", ""], ["16.1", "J1 Body to Chassis", "< 2m", "-", "ohms", "", ""], ["16.2", "J2  Body to Chassis", "< 2m", "-", "ohms", "", ""], ["16.3", "J3  Body to Chassis", "< 2m", "-", "ohms", "", ""], ["", "", "", "", "", "", ""], ["17", "CANbus Resistance Test", "", "", "", "", ""], ["17.1", "J1.17 to J1.18", "> 10K", "-", "ohms", "", ""], ["", "", "", "", "", "", ""], ["18", "Sealing Test", "N/A", "-", "", "", ""], ["", "", "", "", "", "", ""], ["19", "Mounting Holes Test - Jig Fit", "214", "-", "mm", "", ""]] ("ArrEbay 2")
          }
        }
        "UUT" <- w2109
        "UUT" <- w2081
        n755 = for {
          tunnel: w2110 -> [w2191] mode=indexing
          tunnel: w2108 -> [w2189]
          tunnel: [w2188] -> w2078
          tunnel: w2110 -> [w2187]
          i -> [w2190]
          n756 = for {
            tunnel: w2191 -> [_] mode=indexing
            tunnel: w2190 -> [w2197]
            tunnel: w2189 -> [w2194]
            tunnel: [w2193] -> w2188
            tunnel: w2187 -> [w2192]
            i -> [w2198]
            n757 = Bundle By Name(cluster=T22 {"Row"=0, "Column"=0} ("Active Cell:Active Cell"), "Row"=w2197, "Column"=w2198) -> (w2196:T22)
            n758 = control-ref of="ATR"() -> (w2195:refnum<vi>)
            n759 = property class="Tbl (strict)"(reference=w2195, error in=w2194, "Active Cell"=w2196, "Cell BG Color"=u32 16777226, "Value"=w2192) -> (error out=w2193:errorcluster)  [unwired: 1 out]
          }
        }
        n760 = case shown="95" w2081 {
          tunnel: ["AHU Software Version" ("key") "AHU Software Version" ("key") "EBAY Software Version" ("key")] -> w2098
          tunnel: ["AHU R Serial Number" ("key") "AHU L Serial Number" ("key") "EBAY Serial Number" ("key")] -> w2099
          tunnel: [2 2 1] -> w2083
          frame 63, Default {
          }
          frame 47 {
          }
          frame 95 {
          }
        }
        n761 = call <vilib>:"Open Config Data.vi"("error in (no error)"=w2078, "create file if necessary (T)"=FALSE, "configuration file path"=w2092) -> ("error out"=w2093:errorcluster, "refnum"=w2094:T12)  [unwired: 7 out]
        n762 = call-poly <vilib>:"Read Key.vi"("section"=w2096, "error in (no error)"=w2093, "key"=w2098, "refnum"=w2094) -> ("error out"=w2100:errorcluster, "value"=→"UUT SoftwareVer":string, "refnum out"=w2097:T12)  [unwired: 2 in, 3 out]
        n763 = property on="Start" class="Bool (strict)"("DisabledEnum"=w2084) -> ()  [unwired: 2 in, 2 out]
        n764 = property on="Report" class="Bool (strict)"("DisabledEnum"=w2084) -> ()  [unwired: 2 in, 2 out]
        n765 = call-poly <vilib>:"Read Key.vi"("section"=w2096, "error in (no error)"=w2100, "key"=w2099, "refnum"=w2097) -> ("error out"=w2090:errorcluster, "value"=w2088:string, "refnum out"=w2089:T12)  [unwired: 2 in, 3 out]
        n766 = call <vilib>:"Close Config Data.vi"("error in (no error)"=w2090, "refnum"=w2089) -> ("error out"=w2079:errorcluster)  [unwired: 8 in, 1 out]
        n767 = Decimal String To Number(string=w2088) -> (number=w2082:i32)  [unwired: 2 in, 1 out]
        n768 = case shown="47" w2081 {
          tunnel: w2082 -> [w2136 w2149 _]
          tunnel: [w2132 w2145 T11."MainProgram"] -> w2080
          tunnel: w2079 -> [w2131 w2144 w2157]
          tunnel: [w2131 w2144 w2157] -> w2077
          tunnel: [w2130 w2143 FALSE] -> w2075
          frame 63, Default {
            n769 = Quotient & Remainder(x=w2136, y=2) -> (x-y*floor(x/y)=w2134:i32)  [unwired: 1 out]
            n770 = Equal To 0?(x=w2134) -> (x = 0?=w2133:bool)
            n771 = case shown="True" w2133 {
              tunnel: [T11."MainProgram" w2140] -> w2132
              tunnel: [FALSE w2139] -> w2130
              frame False {
              }
              frame True {
                n772 = flat-sequence {
                  tunnel: [T11."Stop"] -> w2140
                  tunnel: [TRUE] -> w2139
                  frame #0 {
                    n773 = call "Display Message to User11"() -> ()  [unwired: 10 in, 2 out]
                  }
                  frame #1 {
                  }
                }
              }
            }
          }
          frame 47 {
            n774 = Quotient & Remainder(x=w2149, y=2) -> (x-y*floor(x/y)=w2147:i32)  [unwired: 1 out]
            n775 = Not Equal To 0?(x=w2147) -> (x != 0?=w2146:bool)
            n776 = case shown="True" w2146 {
              tunnel: [T11."MainProgram" w2153] -> w2145
              tunnel: [FALSE w2152] -> w2143
              frame False {
              }
              frame True {
                n777 = flat-sequence {
                  tunnel: [T11."Stop"] -> w2153
                  tunnel: [TRUE] -> w2152
                  frame #0 {
                    n778 = call "Display Message to User13"() -> ()  [unwired: 10 in, 2 out]
                  }
                  frame #1 {
                  }
                }
              }
            }
          }
          frame 95 {
          }
        }
        n779 = case shown="False" w2075 {
          tunnel: w2077 -> [w2121 w2129]
          tunnel: [w2120 w2129] -> w2076
          frame False {
            n780 = call "Boards S/N"("error in (no error)"=w2121) -> ("POWER Board S/N"=→"POWER Board S/N":string, "DSP Board S/N"=→"DSP Board S/N":string, "error out"=w2119:errorcluster)  [unwired: 15 in, 1 out]
            n781 = call "COM EvolutionBoard.vi"("error in (no error)"=w2119, "VISA resource name 2"=refnum<visa-resource-name> "COM1" ("VISA resource name")) -> ("error out"=w2127:errorcluster, "VISA resource name out"=w2126:refnum<visa-resource-name>)  [unwired: 8 in]
            n782 = call "TesterOption (SubVI).vi"("2 Options"=FALSE, "error in (no error)"=w2127, "On/Off"=FALSE, "Tester Option"=T13."Venable", "VISA Refnum in"=w2126) -> ("error out"=w2120:errorcluster, "VISA Refnum out"=→"VISA Tester":refnum<visa-resource-name>)  [unwired: 5 in]
          }
          frame True {
          }
        }
        n783 = Add(x=w2082, y=w2083) -> (x+y=→"Next SN":i32)
      }
      frame "Stop" {
        w2201 = 0
        n784 = flat-sequence {
          tunnel: w2234 -> [w2272]
          tunnel: [w2271] -> w2227
          frame #0 {
            n785 = control-ref of="Pannel User Message"() -> (w2274:refnum<vi>)
            n786 = property class="Str"(reference=w2274, error in=w2272, "Value"="Program Stopped...\r\nPlease turn OFF All Power sinks") -> (error out=w2271:errorcluster)  [unwired: 1 out]
          }
        }
        n787 = control-ref of="VISA Tester"() -> (w2235:refnum<vi>)
        n788 = property class="VISAName"(reference=w2235, error in=w2227) -> ("Value"=w2233:refnum<visa-resource-name>)  [unwired: 2 out]
        n789 = disable-structure shown="Enabled" {
          disable-tunnel: w2227 -> [w2259 w2260]
          disable-tunnel: w2226 -> [w2257 _]
          disable-tunnel: [w2256 w2260] -> w2213
          frame Disabled {
            n790 = call "Clear CAN Buffer.vi"("error in (no error)"=w2259, "Cluster in"=w2257) -> ("error out"=w2258:errorcluster)  [unwired: 8 in, 1 out]
            n791 = call "Close CAN Device.vi"("error in (no error)"=w2258, "Cluster in"=w2257) -> ("error out"=w2256:errorcluster)  [unwired: 8 in, 1 out]
          }
          frame Enabled {
          }
        }
        n792 = VISA Close(VISA resource name=w2242, error in (no error)=w2227) -> (error out=w2236:errorcluster)
        n793 = property on="Stop Button" class="Bool (strict)"() -> ("Value"=w2205:bool)  [unwired: 2 in, 2 out]
        n794 = call "TesterOption (SubVI).vi"("2 Options"=FALSE, "On/Off"=FALSE, "Tester Option"=T13."Power", "VISA Refnum in"=w2233) -> ("error out"=w2222:errorcluster, "VISA Refnum out"=w2232:refnum<visa-resource-name>)  [unwired: 6 in]
        n795 = property on="ClosePanel" class="Bool (strict)"() -> ("Value"=w2206:bool)  [unwired: 2 in, 2 out]
        n796 = VISA Close(VISA resource name=w2232, error in (no error)=w2222) -> (error out=w2219:errorcluster)
        n797 = Or(x=w2206, y=w2205) -> (x .or. y?=w2204:bool)
        n798 = Flush Queue(queue=w2237, error in (no error)=w2236) -> (queue out=w2239:refnum<queue>, error out=w2238:errorcluster)  [unwired: 1 out]
        n799 = Flush Queue(queue=w2244, error in (no error)=w2236) -> (queue out=w2243:refnum<queue>, error out=w2245:errorcluster)  [unwired: 1 out]
        n800 = case shown="False" w2204 {
          tunnel: w2245 -> [w2247 w2255]
          tunnel: w2243 -> [w2249 w2251]
          tunnel: w2239 -> [w2248 w2250]
          tunnel: w2238 -> [w2246 w2254]
          tunnel: [w2247 w2253] -> w2221
          tunnel: [w2246 w2252] -> w2220
          tunnel: [w2249 w2251] -> w2203
          tunnel: [w2248 w2250] -> w2202
          frame False {
          }
          frame True {
            n801 = Release Queue(queue=w2250, error in (no error)=w2254) -> (error out=w2252:errorcluster)  [unwired: 1 in, 2 out]
            n802 = Release Queue(queue=w2251, error in (no error)=w2255) -> (error out=w2253:errorcluster)  [unwired: 1 in, 2 out]
          }
        }
        n803 = Merge Errors(w2221, w2220, w2219, w2213) -> (w2218:errorcluster)
        n804 = property on="Refresh Button" class="Bool (strict)"() -> ("Value"=w2207:bool)  [unwired: 2 in, 2 out]
        n805 = call <vilib>:"Clear Errors.vi"("error in (no error)"=w2218) -> ("error out"=w2217:errorcluster)  [unwired: 5 in, 1 out]
        n806 = property on="Stop Button" class="Bool (strict)"() -> ("Value"=w2211:bool)  [unwired: 2 in, 2 out]
        n807 = property on="ClosePanel" class="Bool (strict)"(error in=w2217) -> (error out=w2215:errorcluster, "Value"=w2216:bool)  [unwired: 1 in, 1 out]
        n808 = Not(x=w2207) -> (.not. x?=w2208:bool)
        n809 = Select(t=T11."Initialize", s=w2207, f=T11."Stop") -> (s? t:f=w2223:T11)
        n810 = Not(x=w2211) -> (.not. x?=w2210:bool)
        n811 = Compound Arithmetic op=AND(w2216, w2210, w2208) -> (w2212:bool)
        n812 = case shown="False" w2212 {
          tunnel: w2215 -> [w2263 w2267]
          tunnel: [w2263 w2267] -> w2214
          tunnel: [w2262 w2266] -> w2209
          tunnel: w2207 -> [w2261 _]
          frame False {
            n813 = case shown="False" w2261 {
              tunnel: [TRUE FALSE] -> w2262
              frame False {
              }
              frame True {
              }
            }
          }
          frame True {
            n814 = flat-sequence {
              tunnel: [TRUE] -> w2266
              frame #0 {
              }
              frame #1 {
                n815 = control-ref of="This VI"() -> (w2270:refnum<vi>)
                n816 = property class="VI"(reference=w2270, "FP.State"=T23."Closed" ("Front Panel Window:State")) -> ()  [unwired: 1 in, 2 out]
              }
            }
          }
        }
      }
      frame "MainProgram" {
        n817 = event shown="[0] Timeout" {
          selector: w2285 -> [_ _ _ _ _ _ _ _ _ _ _ _ _]
          dyn-events: _ -> [_ _ _ _ _ _ _ _ _ _ _ _ _]
          timeout: 70 -> [_ _ _ _ _ _ _ _ _ _ _ _ _]
          tunnel: [T11."MainProgram" T11."MainProgram" T11."MainProgram" T11."MainProgram" T11."MainProgram" T11."Stop" T11."MainProgram" w2975 T11."MainProgram" T11."MainProgram" T11."MainProgram" T11."Stop" T11."MainProgram"] -> w2298
          tunnel: [w2305 w2451 w2523 w2532 w2543 w2563 w2590 w3023 w3094 w3109 w3121 w3209 w3217] -> w2292
          tunnel: w2296 -> [w2330 w2451 w2522 w2534 w2543 w2563 w2597 w3023 w3095 w3108 w3117 w3209 w3222]
          tunnel: [w2338 w2445 w2524 w2533 w2544 w2561 w2586 w2980 w3092 w3106 w3122 w3207 w3215] -> w2293
          tunnel: w2294 -> [w2338 w2445 w2524 w2533 w2544 w2561 w2586 w2980 w3092 w3106 _ w3207 w3215]
          tunnel: w2291 -> [w2332 w2457 w2518 w2529 w2540 w2560 w2595 w3007 w3091 w3105 w3125 w3206 w3220]
          tunnel: w2290 -> [w2328 w2456 w2519 w2530 w2541 w2559 w2568 w3006 w3090 w3104 w3124 w3205 w3213]
          tunnel: [w2329 w2456 w2519 w2530 w2541 w2559 w2568 w3006 w3090 w3104 w3124 w3205 w3213] -> w2289
          tunnel: [w2331 w2457 w2518 w2529 w2540 w2560 w2595 w3007 w3091 w3105 w3125 w3206 w3220] -> w2288
          tunnel: w2287 -> [w2326 w2455 w2517 w2528 w2539 w2558 w2594 w3005 w3089 w3103 w3123 w3204 w3219]
          tunnel: [w2326 w2455 w2517 w2528 w2539 w2558 w2589 w3005 w3089 w3103 w3123 w3204 w3219] -> w2286
          tunnel: w2284 -> [_ _ _ _ _ _ _ w2951 _ _ _ _ _]
          tunnel: w2283 -> [w2327 w2454 w2516 w2527 w2538 w2556 w2584 w2984 w3088 w3102 w3119 w3203 w3218]
          tunnel: [w2327 w2454 w2516 w2527 w2538 w2556 w2584 w2983 w3088 w3102 w3119 w3203 w3218] -> w2282
          tunnel: w2281 -> [_ w2452 _ _ _ _ _ w2982 _ _ _ _ _]
          tunnel: w2280 -> [_ w2444 _ _ _ _ _ _ _ _ _ _ _]
          tunnel: w2279 -> [_ _ _ _ _ _ _ _ w3087 _ _ _ _]
          tunnel: w2278 -> [w2302 w2425 w2515 w2526 w2537 w2553 w2567 w2953 w3085 w3101 w3114 w3202 w3211]
          tunnel: [w2301 w2425 w2515 w2526 w2537 w2553 w2567 w2953 w3085 w3101 w3114 w3202 w3211] -> w2277
          tunnel: w2276 -> [w2300 w2424 w2514 w2525 w2536 w2552 w2566 w2940 w3084 w3100 w3113 w3201 w3210]
          tunnel: [w2299 w2424 w2514 w2525 w2536 w2552 w2566 w2940 w3084 w3100 w3113 w3201 w3210] -> w2275
          event Timeout {
            n818 = event-data() -> ()  [unwired: 1 in, 3 out]
            n819 = property on="UUT" class="DigNum (strict)"() -> ("Value"=w2303:u8)  [unwired: 2 in, 2 out]
            n820 = property class="Clust (strict)"(reference=w2328, error in=w2330) -> (reference out=w2329:refnum<vi>, error out=w2304:errorcluster, "Value"=w2335:T8)
            n821 = case shown="95" w2303 {
              tunnel: w2304 -> [_ w2343]
              tunnel: w2302 -> [_ w2342]
              tunnel: [0 w2341] -> w2301
              frame 0, Default {
              }
              frame 95 {
                n822 = case shown="12" w2342 {
                  selector: w2342 -> [w2345 _]
                  tunnel: w2343 -> [_ w2349]
                  tunnel: [w2344 0] -> w2341
                  frame 0, Default {
                    n823 = Increment(x=w2345) -> (x+1=w2344:i32)
                  }
                  frame 12 {
                    n824 = property on="CurrentTest" class="Enum (strict)"() -> ("Value"=w2350:T1)  [unwired: 2 in, 2 out]
                    n825 = case shown="\"Temp Sens Cal\"" w2350 {
                      tunnel: [TRUE TRUE TRUE TRUE TRUE TRUE FALSE TRUE TRUE TRUE] -> w2348
                      tunnel: [u16 0 u16 0 u16 0 w2359 w2361 u16 0 u16 0 w2367 u16 0 u16 0] -> w2347
                      frame "Auxiliary", Default {
                      }
                      frame "Temp Sens Cal" {
                      }
                      frame "Com Test" {
                      }
                      frame "Enable Test" {
                        n826 = property on="VenableSpeed" class="DigNum (strict)"() -> ("Value"=w2359:u16)  [unwired: 2 in, 2 out]
                      }
                      frame "Speed Command" {
                        n827 = property on="SpeedCommandSpeed" class="DigNum (strict)"() -> ("Value"=w2361:u16)  [unwired: 2 in, 2 out]
                      }
                      frame "Stop Time" {
                      }
                      frame "Temp Control" {
                      }
                      frame "Burn in" {
                        n828 = property on="BurnInSpeed" class="DigNum (strict)"() -> ("Value"=w2367:u16)  [unwired: 2 in, 2 out]
                      }
                      frame "Visual Inspec" {
                      }
                      frame "Empty" {
                      }
                    }
                    n829 = control-ref of="Config_CANAT"() -> (w2352:refnum<vi>)
                    n830 = control-ref of="UUT"() -> (w2351:refnum<vi>)
                    n831 = call "CANSendMotorSpeed.vi"("Remote"=w2348, "error in (no error)"=w2349, "Motor Speed RPM"=w2347, "UUT"=w2351, "CAN Cluster in"=w2352) -> ()  [unwired: 6 in, 1 out]
                  }
                }
              }
            }
            n832 = Unbundle By Name(w2335) -> ("DevType"=w2336:T3, "CanIndex"=w2334:T2)
            n833 = property on="ClosePanel" class="Bool (strict)"("Value"=FALSE ("ClosePanel")) -> ()  [unwired: 2 in, 2 out]
            n834 = call "VCI_Receive.vi"("CANIndex"=w2334, "DevIndex"=u32 0, "DevType"=w2336) -> ("Recieve"=w2333:T26[])  [unwired: 3 in, 5 out]
            n835 = Empty Array?(array=w2333) -> (empty?=w2321:bool)
            n836 = case shown="True" w2321 {
              tunnel: w2334 -> [w2386 _]
              tunnel: w2329 -> [w2384 _]
              tunnel: w2332 -> [w2383 w2423]
              tunnel: w2304 -> [w2382 w2422]
              tunnel: w2333 -> [w2387 _]
              tunnel: [w2377 w2422] -> w2305
              tunnel: [w2376 w2423] -> w2331
              tunnel: [TRUE w2417] -> w2319
              tunnel: w2300 -> [_ w2421]
              tunnel: [0 w2420] -> w2299
              frame False {
                n837 = call "Demo_MakeDispBuff.vi"("Channel"=w2386, "Type"=enum16{"接收", "发送"}."接收", "OBJs"=w2387) -> ("Buffer"=w2385:T27)
                n838 = for {
                  N: 3 -> [_]
                  tunnel: w2385 -> [w2401]
                  tunnel: w2384 -> [w2400]
                  tunnel: w2383 -> [w2391]
                  tunnel: w2382 -> [w2390]
                  tunnel: [w2393] -> w2380 mode=indexing
                  tunnel: [w2391] -> w2379
                  tunnel: [w2390] -> w2378
                  i -> [w2389]
                  n839 = property class="Clust (strict)"(reference=w2400) -> ("Value"=w2398:T8)  [unwired: 1 in, 2 out]
                  n840 = Index Array(array=w2401, index=w2389) -> (element=w2394:T28)
                  n841 = Unbundle By Name(w2394) -> ("Channel"=w2396:T2, "VCI_CAN_OBJ"=w2399:T26)  [unwired: 2 out]
                  n842 = Unbundle By Name(w2398) -> ("CanIndex"=w2397:T2)
                  n843 = Equal?(x=w2397, y=w2396) -> (x = y?=w2395:bool)
                  n844 = case shown="True" w2395 {
                    tunnel: w2399 -> [_ w2412]
                    tunnel: [w2402 w2408] -> w2393
                    tunnel: T24 {"ID"=0, "MSGTYPE"=0, "LEN"=0, "aDATA"=[]} ("Msg") -> [w2402 w2407]
                    frame False {
                    }
                    frame True {
                      n845 = Unbundle By Name(w2412) -> ("ID"=w2406:u32, "DataLen"=w2411:u8, "Data"=w2409:u8[])
                      n846 = Bundle By Name(cluster=w2407, "ID"=w2406, "MSGTYPE"=u8 0, "LEN"=w2411, "aDATA"=w2409) -> (w2408:T24)
                      n847 = Unbundle By Name(w2408) -> ("ID"=w2404:u32)
                      n848 = Split Number(x=w2404) -> (lo(x)=w2405:u16)  [unwired: 1 out]
                      n849 = Split Number(x=w2405) -> (lo(x)=w2403:u8)  [unwired: 1 out]
                      n850 = case shown="63" w2403 {
                        tunnel: ["EBAY 5F" "" "AHU 3F" "AHU 2F"] -> _
                        frame 95 {
                        }
                        frame Default {
                        }
                        frame 63 {
                        }
                        frame 47 {
                        }
                      }
                    }
                  }
                }
                n851 = Enqueue Element(queue=w2379, element=w2380, error in (no error)=w2378) -> (queue out=w2376:refnum<queue>, error out=w2377:errorcluster)  [unwired: 2 out]
              }
              frame True {
                n852 = Increment(x=w2421) -> (x+1=w2420:i32)
                n853 = Greater Or Equal?(x=w2420, y=7) -> (x >= y?=w2418:bool)
                n854 = Not(x=w2418) -> (.not. x?=w2417:bool)
              }
            }
            n855 = property on="CAN Status" class="Bool (strict)"("Value"=w2319) -> ()  [unwired: 2 in, 2 out]
            n856 = control-ref of="ATR"() -> (w2320:refnum<vi>)
            n857 = call <vilib>:"Application Directory.vi"() -> ("Application Directory"=w2313:path)
            n858 = call "PassFailUUT (SubVI).vi"("error in (no error)"=w2305, "Table in"=w2320) -> ("PassFaileUUTresult"=w2309:bool)  [unwired: 7 in, 2 out]
            n859 = Select(t="PASS" ("name or relative path"), s=w2309, f="FAIL" ("name or relative path")) -> (s? t:f=w2306:string)
            n860 = Build Path(base path=w2313, name or relative path="data\\TestResult.ini") -> (appended path=w2317:path)
            n861 = property on="Test Failed" class="Bool (strict)"("Value"=w2309) -> ()  [unwired: 2 in, 2 out]
            n862 = call <vilib>:"Open Config Data.vi"("configuration file path"=w2317) -> ("error out"=w2315:errorcluster, "refnum"=w2316:T12)  [unwired: 2 in, 7 out]
            n863 = property on="Automation" class="Bool (strict)"() -> ("Value"=w2323:bool)  [unwired: 2 in, 2 out]
            n864 = call-poly <vilib>:"Write Key.vi"("section"="Marvin", "error in (no error)"=w2315, "value"=w2306, "key"="Result", "refnum"=w2316) -> ("error out"=w2312:errorcluster, "refnum out"=w2311:T12)  [unwired: 4 in, 1 out]
            n865 = property on="Start" class="Bool (strict)"() -> ("Value"=w2325:bool)  [unwired: 2 in, 2 out]
            n866 = Or(x=w2323, y=w2325) -> (x .or. y?=w2324:bool)
            n867 = call <vilib>:"Close Config Data.vi"("error in (no error)"=w2312, "refnum"=w2311) -> ()  [unwired: 8 in, 2 out]
            n868 = case shown="False" w2324 {
              frame False {
                n869 = property on="Pannel User Message" class="Str"("Value"="You can press start to execute(s) test(s).") -> ()  [unwired: 2 in, 2 out]
              }
              frame True {
              }
            }
          }
          event "SetSN": Value Change {
            n870 = event-data() -> ()  [unwired: 1 in, 6 out]
            n871 = property on="UUT" class="DigNum (strict)"() -> ("Value"=w2435:u8)  [unwired: 2 in, 2 out]
            n872 = Equal?(x=w2435, y=u8 95) -> (x = y?=w2433:bool)
            n873 = control-ref of="ATR"() -> (w2436:refnum<vi>)
            n874 = Select(t=u8 50 ("y"), s=w2433, f=u8 36 ("y")) -> (s? t:f=w2428:u8)
            n875 = property on="Current SN" class="DigNum (strict)"(error in=w2451) -> (error out=w2430:errorcluster, "Value"=w2450:i32)  [unwired: 1 in, 1 out]
            n876 = call "PassFailUUT (SubVI).vi"("error in (no error)"=w2430, "Table in"=w2436) -> ("Total Pass"=w2429:u8)  [unwired: 7 in, 2 out]
            n877 = Equal To 0?(x=w2450) -> (x = 0?=w2447:bool)
            n878 = Equal?(x=w2450, y=-1) -> (x = y?=w2448:bool)
            n879 = Equal?(x=w2429, y=w2428) -> (x = y?=w2427:bool)
            n880 = Or(x=w2448, y=w2447) -> (x .or. y?=w2446:bool)
            n881 = property on="CAN Status" class="Bool (strict)"() -> ("Value"=w2437:bool)  [unwired: 2 in, 2 out]
            n882 = property on="Status" class="Bool (strict)"() -> ("Value"=w2442:bool)  [unwired: 2 in, 2 out]
            n883 = And(x=w2442, y=w2437) -> (x .and. y?=w2438:bool)
            n884 = case shown="True" w2438 {
              tunnel: w2452 -> [_ w2471]
              tunnel: w2446 -> [_ w2460]
              tunnel: w2445 -> [_ w2470]
              tunnel: w2444 -> [_ w2469]
              tunnel: [errorcluster {"status"=FALSE, "code"=0, "source"=""} ("error out") w2468] -> w2441
              tunnel: [w2458 w2467] -> w2443
              tunnel: w2427 -> [_ w2461]
              frame False {
                w2458 = FALSE ("Value")
                n885 = property on="SetSN" class="Bool (strict)"("Value"=w2458) -> ()  [unwired: 2 in, 2 out]
                n886 = call "Display Message to User10"() -> ()  [unwired: 10 in, 2 out]
              }
              frame True {
                n887 = property on="Test Failed" class="Bool (strict)"() -> ("Value"=w2465:bool)  [unwired: 2 in, 2 out]
                n888 = property on="Automation" class="Bool (strict)"() -> ("Value"=w2467:bool)  [unwired: 2 in, 2 out]
                n889 = Not(x=w2465) -> (.not. x?=w2466:bool)
                n890 = Select(t=w2466, s=w2467, f=w2469) -> (s? t:f=w2463:bool)
                n891 = Or(x=w2461, y=w2463) -> (x .or. y?=w2462:bool)
                n892 = And(x=w2460, y=w2462) -> (x .and. y?=w2464:bool)
                n893 = case shown="True" w2464 {
                  tunnel: w2471 -> [_ w2502]
                  tunnel: w2470 -> [_ w2495]
                  tunnel: [w2473 w2487] -> w2468
                  tunnel: w2460 -> [w2472 _]
                  frame False {
                    n894 = case shown="True" w2472 {
                      tunnel: [w2475 w2476] -> w2473
                      frame False {
                        n895 = call "Display Message to User9"() -> ("error out"=w2475:errorcluster)  [unwired: 10 in, 1 out]
                      }
                      frame True {
                        n896 = call "Display Message to User3"() -> ("error out"=w2476:errorcluster)  [unwired: 10 in, 1 out]
                      }
                    }
                    n897 = property on="Automation" class="Bool (strict)"(error in=w2473, "Value"=FALSE ("Automation")) -> ()  [unwired: 1 in, 2 out]
                  }
                  frame True {
                    w2494 = FALSE ("SetSN")
                    n898 = property on="Next SN" class="DigNum (strict)"() -> ("Value"=w2478:i32)  [unwired: 2 in, 2 out]
                    n899 = property on="VISA Tester" class="VISAName"() -> ("Value"=w2485:refnum<visa-resource-name>)  [unwired: 2 in, 2 out]
                    n900 = call "TesterOption (SubVI).vi"("2 Options"=FALSE, "On/Off"=FALSE, "Tester Option"=T13."Venable", "VISA Refnum in"=w2485) -> ("error out"=w2480:errorcluster)  [unwired: 6 in, 1 out]
                    n901 = call <vilib>:"Clear Errors.vi"("error in (no error)"=w2480) -> ("error out"=w2481:errorcluster)  [unwired: 5 in, 1 out]
                    n902 = Number To Decimal String(number=w2478) -> (decimal integer string=w2479:string)  [unwired: 1 in]
                    "UUT SN Report" <- w2479
                    n903 = Search and Replace String(input string="EP=1\r\nSN=0\r\n" ("write buffer"), search string="0", replace string=w2479) -> (result string=w2497:string)  [unwired: 5 in, 3 out]
                    n904 = call "SerialMarvinSendGet.vi"("error in (no error)"=w2481, "Clear Log"=FALSE, "write buffer"=w2497, "VISA resource name"=w2495) -> ("error out"=w2486:errorcluster)  [unwired: 6 in, 1 out]
                    n905 = property on="UUT" class="DigNum (strict)"(error in=w2486) -> ("Value"=w2503:u8)  [unwired: 1 in, 2 out]
                    n906 = case shown="47" w2503 {
                      tunnel: ["AHU R Serial Number" ("key") "AHU L Serial Number" ("key") "EBAY Serial Number" ("key")] -> w2506
                      tunnel: [2 2 1] -> w2477
                      frame 63, Default {
                      }
                      frame 47 {
                      }
                      frame 95 {
                      }
                    }
                    n907 = call <vilib>:"Open Config Data.vi"("create file if necessary (T)"=FALSE, "configuration file path"=w2502) -> ("error out"=w2500:errorcluster, "refnum"=w2501:T12)  [unwired: 1 in, 7 out]
                    n908 = call-poly <vilib>:"Write Key.vi"("section"="Marvin", "error in (no error)"=w2500, "value"=w2479, "key"=w2506, "refnum"=w2501) -> ("error out"=w2490:errorcluster, "refnum out"=w2489:T12)  [unwired: 4 in, 1 out]
                    n909 = call <vilib>:"Close Config Data.vi"("error in (no error)"=w2490, "refnum"=w2489) -> ("error out"=w2488:errorcluster)  [unwired: 8 in, 1 out]
                    n910 = property on="Current SN" class="DigNum (strict)"("Value"=w2478) -> ()  [unwired: 2 in, 2 out]
                    n911 = property on="SetSN" class="Bool (strict)"(error in=w2488, "Value"=w2494) -> (error out=w2493:errorcluster)  [unwired: 1 in, 1 out]
                    n912 = property on="Automation" class="Bool (strict)"(error in=w2493, "Value"=w2494) -> (error out=w2492:errorcluster)  [unwired: 1 in, 1 out]
                    n913 = Add(x=w2478, y=w2477) -> (x+y=w2491:i32)
                    n914 = property on="Next SN" class="DigNum (strict)"(error in=w2492, "Value"=w2491) -> (error out=w2487:errorcluster)  [unwired: 1 in, 1 out]
                  }
                }
              }
            }
            n915 = call <vilib>:"Clear Errors.vi"("error in (no error)"=w2441) -> ("error out"=w2426:errorcluster)  [unwired: 5 in, 1 out]
            n916 = property on="SetSN" class="Bool (strict)"(error in=w2426, "Value"=FALSE ("SetSN")) -> (error out=w2440:errorcluster)  [unwired: 1 in, 1 out]
            n917 = case shown="True" w2443 {
              tunnel: w2440 -> [_ _]
              frame False {
              }
              frame True {
                w2513 = TRUE ("Value (Signaling)")
                n918 = property on="Report" class="Bool (strict)"("Val(Sgnl)"=w2513, "Value"=w2513) -> ()  [unwired: 2 in, 2 out]
              }
            }
          }
          event "ATR": Mouse Enter {
            n919 = event-data() -> ()  [unwired: 1 in, 4 out]
            n920 = call-poly <vilib>:"Set Cursor.vi"("error in (no error)"=w2522, "icon"=u16 1) -> ("error out"=w2523:errorcluster)  [unwired: 8 in, 1 out]
          }
          event "ATR": Mouse Leave {
            n921 = event-data() -> ()  [unwired: 1 in, 4 out]
            n922 = call-poly <vilib>:"Set Cursor.vi"("error in (no error)"=w2534, "icon"=u16 0) -> ("error out"=w2532:errorcluster)  [unwired: 8 in, 1 out]
          }
          event "ATR": Mouse Down? {
            n923 = event-data() -> ("Coords"=w2551:T29)  [unwired: 1 in, 4 out]
            n924 = invoke on="ATR" class="Tbl (strict)" method="Point To Row Column"("Point"=w2551) -> ("InBounds"=w2547:bool, "CellPosition"=w2546:T22)  [unwired: 5 in, 4 out]
            n925 = Greater Than 0?(x=w2546) -> (x > 0?=w2550:cluster{"Row":bool, "Column":bool})
            n926 = Cluster To Array(cluster=w2550) -> (array=w2549:bool[])
            n927 = Or Array Elements(Boolean array=w2549) -> (logical OR=w2548:bool)
            n928 = Or(x=w2547, y=w2548) -> (x .or. y?=w2545:bool)
            n929 = event-data("Discard?"=w2545) -> ()  [unwired: 1 in, 1 out]
          }
          event Panel Close? {
            n930 = event-data() -> ("VIRef"=w2557:refnum<vi>)  [unwired: 1 in, 3 out]
            n931 = Close Reference(reference=w2557) -> ()  [unwired: 1 in, 1 out]
            n932 = disable-structure shown="Disabled" {
              frame Disabled {
                n933 = property on="Stop Button" class="Bool (strict)"("Val(Sgnl)"=TRUE ("Stop Button"), "Value"=FALSE ("Stop Button")) -> ()  [unwired: 2 in, 2 out]
              }
              frame Enabled {
              }
            }
            n934 = event-data("Discard?"=TRUE) -> ()  [unwired: 1 in, 1 out]
            "ClosePanel" <- TRUE ("ClosePanel")
          }
          event "Start": Value Change {
            w2585 = T18 [] items=["Auxiliary", "Temp Sens Cal", "Com Test", "Enable Test", "Speed Command", "Stop Time", "Temp Control", "Burn in", "Visual Inspec", "Empty"]
            n935 = event-data() -> ()  [unwired: 1 in, 2 out]
            n936 = property on="VISA Tester" class="VISAName"() -> ("Value"=w2583:refnum<visa-resource-name>)  [unwired: 2 in, 2 out]
            n937 = property on="UUT" class="Str"(error in=w2597) -> (error out=w2579:errorcluster, "Value"=w2596:string)  [unwired: 1 in, 1 out]
            n938 = control-ref of="Pannel User Message"() -> (w2576:refnum<vi>)
            n939 = control-ref of="Motor Speed RPM"() -> (w2571:refnum<vi>)
            n940 = call "TesterOption (SubVI).vi"("2 Options"=FALSE, "error in (no error)"=w2579, "On/Off"=FALSE, "Tester Option"=T13."Venable", "VISA Refnum in"=w2583) -> ("error out"=w2578:errorcluster)  [unwired: 5 in, 1 out]
            n941 = control-ref of="Stop Burn-in"() -> (w2574:refnum<vi>)
            n942 = control-ref of="Stop Button"() -> (w2575:refnum<vi>)
            n943 = call "Write panel message (SubVI).vi"("Stop BurnIn"=w2574, 4:"rpm"=w2571, 5:"rpm"=FALSE ("rpm"), "PrintTime"=TRUE, "Stop"=w2575, "error in (no error)"=w2578, "Time to wait"=5.0, "Strin"="TESTER BIT TEST OPERATION IN PROCESS", "String in"=w2576) -> ("error out"=w2577:errorcluster)  [unwired: 2 in]
            n944 = while {
              tunnel: w2596 -> [w2625]
              tunnel: [w2624] -> w2592
              tunnel: [w2623] -> w2591
              shift-right: [w2620] -> _
              shift-left: enum16{"Stop", "Tests", "Bit test", "Start"}."Start" -> [w2622]
              tunnel: w2586 -> [w2621]
              tunnel: w2585 -> [w2619]
              tunnel: w2577 -> [w2604]
              tunnel: w2575 -> [w2613]
              tunnel: w2574 -> [w2612]
              tunnel: w2576 -> [w2611]
              tunnel: w2571 -> [w2610]
              tunnel: w2568 -> [w2603]
              stop <- w2618 stop-if-true
              n945 = property class="Clust (strict)"(reference=w2603, error in=w2604) -> ("Value"=w2606:T8)  [unwired: 2 out]
              n946 = Unbundle By Name(w2606) -> ("DevType"=w2608:T3, "CanIndex"=w2607:T2)
              n947 = property on="VISA Tester" class="VISAName"() -> ("Value"=w2616:refnum<visa-resource-name>)  [unwired: 2 in, 2 out]
              n948 = call "VCI_Receive.vi"("CANIndex"=w2607, "DevIndex"=u32 0, "DevType"=w2608) -> ("Recieve"=w2609:T26[])  [unwired: 3 in, 5 out]
              n949 = Empty Array?(array=w2609) -> (empty?=w2602:bool)
              n950 = Not(x=w2602) -> (.not. x?=w2601:bool)
              n951 = property on="CAN Status" class="Bool (strict)"("Value"=w2601) -> (error out=w2600:errorcluster)  [unwired: 2 in, 1 out]
              n952 = property on="CAN Status" class="Bool (strict)"(error in=w2600) -> (error out=w2599:errorcluster, "Value"=w2614:bool)  [unwired: 1 in, 1 out]
              n953 = property on="Status" class="Bool (strict)"(error in=w2599) -> (error out=w2615:errorcluster, "Value"=w2617:bool)  [unwired: 1 in, 1 out]
              n954 = case shown="\"Start\"" w2622 {
                tunnel: w2625 -> [_ w2641 w2774 _]
                tunnel: [w2630 w2640 w2798 w2906] -> w2624
                tunnel: [w2626 w2639 w2772 w2898] -> w2623
                tunnel: w2621 -> [_ _ w2785 w2911]
                tunnel: w2611 -> [_ _ _ w2910]
                tunnel: w2613 -> [_ _ _ w2909]
                tunnel: w2612 -> [_ _ _ w2908]
                tunnel: w2610 -> [_ _ _ w2907]
                tunnel: [w2629 w2638 w2777 w2902] -> w2620
                tunnel: w2619 -> [w2630 _ w2798 w2906]
                tunnel: [w2628 w2637 FALSE FALSE] -> w2618
                tunnel: w2617 -> [_ _ _ w2904]
                tunnel: w2616 -> [_ _ w2768 _]
                tunnel: w2615 -> [w2626 _ _ _]
                tunnel: w2614 -> [_ _ _ w2899]
                frame "Stop", Default {
                  n955 = property on="Start" class="Bool (strict)"(error in=w2626, "Value"=FALSE ("Start")) -> ()  [unwired: 1 in, 2 out]
                  n956 = flat-sequence {
                    tunnel: [enum16{"Stop", "Tests", "Bit test", "Start"}."Stop"] -> w2629
                    tunnel: w2626 -> [_]
                    tunnel: [TRUE] -> w2628
                    frame #0 {
                    }
                  }
                }
                frame "Tests" {
                  w2635 = FALSE ("Stop Burn-in")
                  w2636 = T21."Disabled and Grayed Out" ("Disabled")
                  n957 = case shown="\"EBAY\"" w2641 {
                    tunnel: [w2657 w2706] -> w2640
                    tunnel: [w2656 w2705] -> w2639
                    tunnel: [w2645 w2693] -> w2633
                    frame "AHU", Default {
                      n958 = call "Load Program Process AHU.vi"() -> ("Speed Command Test"=w2650:bool, "Enable Test"=w2651:bool, "Burn-in Test"=w2648:bool, "Auxiliary"=w2646:bool, "Temperature Sensor Calibration Test"=w2653:bool, "Communication Test"=w2652:bool, "Stop Time Test"=w2649:bool, "Visual Inspection"=w2647:bool, "OK"=w2654:bool, "Automation"=w2645:bool, "error out"=w2656:errorcluster)  [unwired: 8 in, 9 out]
                      n959 = Or(x=w2654, y=w2645) -> (x .or. y?=w2655:bool)
                      n960 = case shown="True" w2655 {
                        tunnel: [w2658 w2668] -> w2657
                        tunnel: w2645 -> [_ w2667]
                        tunnel: w2653 -> [_ w2666]
                        tunnel: w2652 -> [_ w2665]
                        tunnel: w2651 -> [_ w2664]
                        tunnel: w2650 -> [_ w2663]
                        tunnel: w2649 -> [_ w2662]
                        tunnel: w2648 -> [_ w2661]
                        tunnel: w2647 -> [_ w2660]
                        tunnel: w2646 -> [_ w2659]
                        frame False {
                          w2658 = T18 [] items=["Auxiliary", "Temp Sens Cal", "Com Test", "Enable Test", "Speed Command", "Stop Time", "Temp Control", "Burn in", "Visual Inspec", "Empty"]
                        }
                        frame True {
                          n961 = case shown="False" w2667 {
                            tunnel: [w2691 w2692] -> w2668
                            tunnel: w2666 -> [w2673 _]
                            tunnel: w2665 -> [w2672 _]
                            tunnel: w2664 -> [w2674 _]
                            tunnel: w2663 -> [w2671 _]
                            tunnel: w2662 -> [w2670 _]
                            tunnel: w2661 -> [w2684 _]
                            tunnel: w2660 -> [w2669 _]
                            tunnel: w2659 -> [_ _]
                            frame False {
                              w2677 = T1."Empty" ("f")
                              n962 = Select(t=T1."Com Test" ("f"), s=w2672, f=w2677) -> (s? t:f=w2683:T1)
                              n963 = Select(t=T1."Temp Sens Cal" ("f"), s=w2673, f=w2677) -> (s? t:f=w2682:T1)
                              n964 = Select(t=T1."Stop Time" ("f"), s=w2670, f=w2677) -> (s? t:f=w2681:T1)
                              n965 = Select(t=T1."Enable Test" ("f"), s=w2674, f=w2677) -> (s? t:f=w2680:T1)
                              n966 = Select(t=T1."Speed Command" ("f"), s=w2671, f=w2677) -> (s? t:f=w2679:T1)
                              n967 = Select(t=T1."Burn in" ("f"), s=w2684, f=w2677) -> (s? t:f=w2678:T1)
                              n968 = Select(t=T1."Visual Inspec" ("f"), s=w2669, f=w2677) -> (s? t:f=w2675:T1)
                              n969 = Build Array(w2683, w2682, w2681, w2680, w2679, w2678, w2675) -> (w2691:T18)
                            }
                            frame True {
                              w2692 = T18 [enum."Com Test", enum."Temp Sens Cal", enum."Stop Time", enum."Enable Test", enum."Speed Command", enum."Burn in", enum."Visual Inspec"] items=["Auxiliary", "Temp Sens Cal", "Com Test", "Enable Test", "Speed Command", "Stop Time", "Temp Control", "Burn in", "Visual Inspec", "Empty"]
                            }
                          }
                        }
                      }
                    }
                    frame "EBAY" {
                      n970 = call "Load Program Process EBAY.vi"() -> ("Speed Command Test"=w2699:bool, "Enable Test"=w2700:bool, "Burn-in Test"=w2697:bool, "Temperature Control Algorithm Test"=w2696:bool, "Auxiliary"=w2694:bool, "Temperature Sensor Calibration Test"=w2702:bool, "Communication Test"=w2701:bool, "Stop Time Test"=w2698:bool, "Visual Inspection"=w2695:bool, "OK"=w2703:bool, "Automation"=w2693:bool, "error out"=w2705:errorcluster)  [unwired: 8 in, 8 out]
                      n971 = Or(x=w2703, y=w2693) -> (x .or. y?=w2704:bool)
                      n972 = case shown="True" w2704 {
                        tunnel: [w2707 w2718] -> w2706
                        tunnel: w2693 -> [_ w2717]
                        tunnel: w2702 -> [_ w2716]
                        tunnel: w2701 -> [_ w2715]
                        tunnel: w2700 -> [_ w2714]
                        tunnel: w2699 -> [_ w2713]
                        tunnel: w2698 -> [_ w2712]
                        tunnel: w2697 -> [_ w2711]
                        tunnel: w2696 -> [_ w2710]
                        tunnel: w2695 -> [_ w2709]
                        tunnel: w2694 -> [_ w2708]
                        frame False {
                          w2707 = T18 [] items=["Auxiliary", "Temp Sens Cal", "Com Test", "Enable Test", "Speed Command", "Stop Time", "Temp Control", "Burn in", "Visual Inspec", "Empty"]
                        }
                        frame True {
                          n973 = case shown="False" w2717 {
                            tunnel: [w2747 w2748] -> w2718
                            tunnel: w2716 -> [w2724 _]
                            tunnel: w2715 -> [w2723 _]
                            tunnel: w2714 -> [w2722 _]
                            tunnel: w2713 -> [w2721 _]
                            tunnel: w2712 -> [w2720 _]
                            tunnel: w2711 -> [w2726 _]
                            tunnel: w2710 -> [w2725 _]
                            tunnel: w2709 -> [w2738 _]
                            tunnel: w2708 -> [w2729 _]
                            frame False {
                              w2727 = T1."Empty" ("f")
                              n974 = Select(t=T1."Com Test" ("f"), s=w2723, f=w2727) -> (s? t:f=w2737:T1)
                              n975 = Select(t=T1."Temp Sens Cal" ("f"), s=w2724, f=w2727) -> (s? t:f=w2736:T1)
                              n976 = Select(t=T1."Stop Time" ("f"), s=w2720, f=w2727) -> (s? t:f=w2735:T1)
                              n977 = Select(t=T1."Enable Test" ("f"), s=w2722, f=w2727) -> (s? t:f=w2734:T1)
                              n978 = Select(t=T1."Speed Command" ("f"), s=w2721, f=w2727) -> (s? t:f=w2733:T1)
                              n979 = Select(t=T1."Temp Control" ("f"), s=w2725, f=w2727) -> (s? t:f=w2732:T1)
                              n980 = Select(t=T1."Burn in" ("f"), s=w2726, f=w2727) -> (s? t:f=w2731:T1)
                              n981 = Select(t=T1."Visual Inspec" ("f"), s=w2738, f=w2727) -> (s? t:f=w2730:T1)
                              n982 = Select(t=T1."Auxiliary" ("f"), s=w2729, f=w2727) -> (s? t:f=w2719:T1)
                              n983 = Build Array(w2737, w2719, w2736, w2735, w2734, w2733, w2732, w2731, w2730) -> (w2747:T18)
                            }
                            frame True {
                              w2748 = T18 [enum."Com Test", enum."Auxiliary", enum."Temp Sens Cal", enum."Stop Time", enum."Enable Test", enum."Speed Command", enum."Temp Control", enum."Burn in", enum."Visual Inspec"] items=["Auxiliary", "Temp Sens Cal", "Com Test", "Enable Test", "Speed Command", "Stop Time", "Temp Control", "Burn in", "Visual Inspec", "Empty"]
                            }
                          }
                        }
                      }
                    }
                  }
                  "Automation" <- w2633
                  n984 = control-ref of="ATR"() -> (w2634:refnum<vi>)
                  n985 = flat-sequence {
                    tunnel: [enum16{"Stop", "Tests", "Bit test", "Start"}."Tests"] -> w2638
                    tunnel: [TRUE] -> w2637
                    frame #0 {
                    }
                  }
                  n986 = case shown="True" w2633 {
                    tunnel: w2634 -> [_ w2642]
                    frame False {
                    }
                    frame True {
                      n987 = call "ResetTable Result (SubVI).vi"("Table in"=w2642) -> ()  [unwired: 11 in]
                    }
                  }
                  n988 = property on="Stop Button" class="Bool (strict)"("Value"=w2635) -> ()  [unwired: 2 in, 2 out]
                  n989 = property on="Stop Burn-in" class="Bool (strict)"("Value"=w2635) -> ()  [unwired: 2 in, 2 out]
                  n990 = property on="Start" class="Bool (strict)"("DisabledEnum"=w2636) -> ()  [unwired: 2 in, 2 out]
                  n991 = property on="Report" class="Bool (strict)"("DisabledEnum"=w2636) -> ()  [unwired: 2 in, 2 out]
                }
                frame "Bit test" {
                  # "Stop"
                  n992 = call "SerialMarvinSendGet.vi"("write buffer"="TA[1]\r\n", "VISA resource name"=w2785) -> ("error out"=w2759:errorcluster, "read buffer"=w2795:string)  [unwired: 8 in]
                  n993 = Fract/Exp String To Number(string=w2795) -> (number=w2758:dbl)  [unwired: 3 in, 1 out]
                  n994 = call "TAs StartTest (SubVI).vi"("error in"=w2759, "Numeric"=w2758, "Enum"=enum16{"TA3", "TA2", "TA1"}."TA1") -> ("error out"=w2757:errorcluster, "String Out"=w2756:string, "Result"=w2755:bool)  [unwired: 6 in]
                  n995 = call "TesterOption (SubVI).vi"("On/Off 2"=FALSE, "Tester Option 2"=T13."Venable", "2 Options"=TRUE, "error in (no error)"=w2757, "On/Off"=TRUE, "Tester Option"=T13."25C", "VISA Refnum in"=w2768) -> ("error out"=w2787:errorcluster)  [unwired: 3 in, 1 out]
                  n996 = call "Time Delay5"("error in (no error)"=w2787) -> ("error out"=w2786:errorcluster)  [unwired: 10 in]
                  n997 = call "SerialMarvinSendGet.vi"("error in (no error)"=w2786, "write buffer"="TA[2]\r\n", "VISA resource name"=w2785) -> ("error out"=w2753:errorcluster, "read buffer"=w2789:string)  [unwired: 7 in]
                  n998 = Fract/Exp String To Number(string=w2789) -> (number=w2752:dbl)  [unwired: 3 in, 1 out]
                  n999 = call "TAs StartTest (SubVI).vi"("error in"=w2753, "Numeric"=w2752, "Enum"=enum16{"TA3", "TA2", "TA1"}."TA2") -> ("error out"=w2751:errorcluster, "String Out"=w2750:string, "Result"=w2749:bool)  [unwired: 6 in]
                  n1000 = call "GetADCTester (SubVI).vi"("error in (no error)"=w2751, "GetADCTester"=T15."Term1", "TimeToGet"=5, "VISA Refnum in"=w2768) -> ("error out"=w2767:errorcluster, "ADCValOutput Single"=w2765:dbl)  [unwired: 5 in, 1 out]
                  n1001 = case shown="\"EBAY\"" w2774 {
                    tunnel: w2768 -> [w2828 _ w2860]
                    tunnel: w2785 -> [_ _ w2863]
                    tunnel: w2767 -> [w2829 w2846 w2862]
                    tunnel: [w2822 w2846 w2859] -> w2776
                    tunnel: [w2819 "" w2856] -> w2782
                    tunnel: [w2818 bool[] [] w2855] -> w2766
                    frame "AHU" {
                      n1002 = call "TesterOption (SubVI).vi"("On/Off 2"=FALSE, "Tester Option 2"=T13."Venable", "2 Options"=TRUE, "error in (no error)"=w2829, "On/Off"=TRUE, "Tester Option"=T13."K17", "VISA Refnum in"=w2828) -> ("error out"=w2831:errorcluster)  [unwired: 3 in, 1 out]
                      n1003 = call "Time Delay7"("error in (no error)"=w2831) -> ("error out"=w2830:errorcluster)  [unwired: 10 in]
                      n1004 = call "GetADCTester (SubVI).vi"("error in (no error)"=w2830, "GetADCTester"=T15."Current", "TimeToGet"=5, "VISA Refnum in"=w2828) -> ("error out"=w2822:errorcluster, "ADCValOutput Single"=w2824:dbl)  [unwired: 5 in, 1 out]
                      n1005 = Less Or Equal?(x=w2824, y=10.0) -> (x <= y?=w2823:bool)
                      n1006 = Build Array(w2823) -> (w2818:bool[])
                      n1007 = for {
                        tunnel: w2818 -> [w2843] mode=indexing
                        tunnel: string[] ["Current sensor not connected!"] -> [w2840] mode=indexing
                        shift-right: [w2841] -> w2819
                        shift-left: "" -> [w2838]
                        n1008 = Concatenate Strings(w2840, "\r\n") -> (w2837:string)
                        n1009 = Select(t=w2838, s=w2843, f=w2837) -> (s? t:f=w2842:string)
                        n1010 = Concatenate Strings(w2838, w2842) -> (w2841:string)
                      }
                    }
                    frame Default {
                    }
                    frame "EBAY" {
                      w2861 = T30 [enum."Fan", enum."Current"] items=["Term1", "Term2", "Current", "Fan", "TempCPU"]
                      n1011 = call "TesterOption (SubVI).vi"("On/Off 2"=FALSE, "Tester Option 2"=T13."Venable", "2 Options"=TRUE, "error in (no error)"=w2862, "On/Off"=TRUE, "Tester Option"=T13."K17", "VISA Refnum in"=w2860) -> ("error out"=w2865:errorcluster)  [unwired: 3 in, 1 out]
                      n1012 = call "Time Delay6"("error in (no error)"=w2865) -> ("error out"=w2864:errorcluster)  [unwired: 10 in]
                      n1013 = call "SerialMarvinSendGet.vi"("error in (no error)"=w2864, "write buffer"="TA[3]\r\n", "VISA resource name"=w2863) -> ("error out"=w2850:errorcluster, "read buffer"=w2867:string)  [unwired: 7 in]
                      n1014 = Fract/Exp String To Number(string=w2867) -> (number=w2851:dbl)  [unwired: 3 in, 1 out]
                      n1015 = call "TAs StartTest (SubVI).vi"("error in"=w2850, "Numeric"=w2851, "Enum"=enum16{"TA3", "TA2", "TA1"}."TA3") -> ("error out"=w2847:errorcluster, "String Out"=w2849:string, "Result"=w2848:bool)  [unwired: 6 in]
                      n1016 = for {
                        tunnel: w2861 -> [w2890] mode=indexing
                        tunnel: w2860 -> [w2889]
                        tunnel: w2847 -> [w2887]
                        tunnel: [w2886] -> w2859
                        tunnel: [w2883] -> w2858 mode=indexing
                        i -> [w2884]
                        n1017 = call "GetADCTester (SubVI).vi"("error in (no error)"=w2887, "GetADCTester"=w2890, "TimeToGet"=5, "VISA Refnum in"=w2889) -> ("error out"=w2886:errorcluster, "ADCValOutput Single"=w2885:dbl)  [unwired: 5 in, 1 out]
                        n1018 = case shown="1" w2884 {
                          tunnel: w2885 -> [w2893 w2896 _]
                          tunnel: [w2891 w2894 FALSE] -> w2883
                          frame 1 {
                            n1019 = Less Or Equal?(x=w2893, y=10.0) -> (x <= y?=w2891:bool)
                          }
                          frame 0 {
                            n1020 = Greater Or Equal?(x=w2896, y=2200.0) -> (x >= y?=w2894:bool)
                          }
                          frame Default {
                          }
                        }
                      }
                      n1021 = Build Array (concatenate)(w2848, w2858) -> (w2855:bool[])
                      n1022 = Build Array (concatenate)(w2849, string[] ["AUX Fan not connected!", "Current sensor not connected!"]) -> (w2853:string[])
                      n1023 = for {
                        tunnel: w2855 -> [w2873] mode=indexing
                        tunnel: w2853 -> [w2876] mode=indexing
                        shift-right: [w2878] -> w2856
                        shift-left: "" -> [w2877]
                        n1024 = Concatenate Strings(w2876, "\r\n") -> (w2874:string)
                        n1025 = case shown="False" w2873 {
                          tunnel: [w2881 w2882] -> w2878
                          tunnel: w2877 -> [w2880 w2882]
                          tunnel: w2874 -> [w2879 _]
                          frame False {
                            n1026 = Concatenate Strings(w2880, w2879) -> (w2881:string)
                          }
                          frame True {
                          }
                        }
                      }
                    }
                  }
                  n1027 = Less Or Equal?(x=w2765, y=100.0) -> (x <= y?=w2763:bool)
                  n1028 = Build Array(w2756, w2750, "Failure - check 28V or GND signals. Pin28 or Pin2") -> (w2762:string[])
                  n1029 = Build Array(w2755, w2749, w2763) -> (w2781:bool[])
                  n1030 = for {
                    tunnel: w2781 -> [w2807] mode=indexing
                    tunnel: w2762 -> [w2811] mode=indexing
                    shift-right: [w2813] -> w2783
                    shift-left: "" -> [w2812]
                    tunnel: w2776 -> [w2808]
                    tunnel: [w2808] -> w2775
                    n1031 = Concatenate Strings(w2811, "\r\n") -> (w2809:string)
                    n1032 = case shown="False" w2807 {
                      tunnel: [w2816 w2817] -> w2813
                      tunnel: w2812 -> [w2815 w2817]
                      tunnel: w2809 -> [w2814 _]
                      frame False {
                        n1033 = Concatenate Strings(w2815, w2814) -> (w2816:string)
                      }
                      frame True {
                      }
                    }
                  }
                  n1034 = Build Array (concatenate)(w2781, w2766) -> (w2780:bool[])
                  n1035 = And Array Elements(Boolean array=w2780) -> (logical AND=w2771:bool)
                  n1036 = case shown="False" w2771 {
                    tunnel: w2783 -> [w2805 _]
                    tunnel: w2782 -> [w2804 _]
                    tunnel: w2775 -> [w2802 w2806]
                    tunnel: [w2802 w2806] -> w2773
                    frame False {
                      n1037 = Concatenate Strings(w2805, w2804) -> (w2803:string)
                      n1038 = One Button Dialog(message=w2803) -> ()  [unwired: 1 in, 1 out]
                    }
                    frame True {
                    }
                  }
                  n1039 = case shown="False" w2771 {
                    tunnel: w2773 -> [w2800 w2801]
                    tunnel: [w2799 w2801] -> w2772
                    frame False {
                      n1040 = call "Display Message to User6"("error in (no error)"=w2800) -> ("error out"=w2799:errorcluster)  [unwired: 9 in, 1 out]
                    }
                    frame True {
                    }
                  }
                  n1041 = Select(t=enum16{"Stop", "Tests", "Bit test", "Start"}."Tests", s=w2771, f=enum16{"Stop", "Tests", "Bit test", "Start"}."Stop") -> (s? t:f=w2777:enum16{"Stop", "Tests", "Bit test", "Start"})
                }
                frame "Start" {
                  n1042 = And(x=w2899, y=w2904) -> (x .and. y?=w2900:bool)
                  n1043 = case shown="True" w2900 {
                    tunnel: w2911 -> [_ w2938]
                    tunnel: w2910 -> [_ w2929]
                    tunnel: w2909 -> [_ w2925]
                    tunnel: w2908 -> [_ w2923]
                    tunnel: w2907 -> [_ w2922]
                    tunnel: [FALSE w2921] -> w2903
                    tunnel: [w2917 w2920] -> w2898
                    tunnel: [FALSE TRUE] -> w2901
                    frame False {
                      n1044 = call "Display Message to User5"() -> ("error out"=w2917:errorcluster)  [unwired: 10 in, 1 out]
                    }
                    frame True {
                      n1045 = property on="VISA Tester" class="VISAName"() -> (error out=w2936:errorcluster, "Value"=w2935:refnum<visa-resource-name>)  [unwired: 2 in, 1 out]
                      n1046 = call "TesterOption (SubVI).vi"("2 Options"=FALSE, "error in (no error)"=w2936, "On/Off"=FALSE, "Tester Option"=T13."Venable", "VISA Refnum in"=w2935) -> ("error out"=w2931:errorcluster)  [unwired: 5 in, 1 out]
                      n1047 = call "Write panel message (SubVI).vi"("Stop BurnIn"=w2923, 4:"rpm"=w2922, 5:"rpm"=FALSE ("rpm"), "PrintTime"=FALSE, "Stop"=w2925, "error in (no error)"=w2931, "Time to wait"=3.0, "Strin"="TESTER BIT TEST OPERATION IN PROCESS\nPlease wait...", "String in"=w2929) -> ("error out"=w2930:errorcluster)  [unwired: 2 in]
                      n1048 = property on="UUT SoftwareVer" class="Str"() -> ("Value"=w2919:string)  [unwired: 2 in, 2 out]
                      n1049 = call "SerialMarvinSendGet.vi"("error in (no error)"=w2930, "write buffer"="VR\r\n", "VISA resource name"=w2938) -> ("error out"=w2920:errorcluster, "read buffer"=w2937:string)  [unwired: 7 in]
                      n1050 = Equal?(x=w2937, y=w2919) -> (x = y?=w2921:bool)
                    }
                  }
                  n1051 = case shown="False" w2903 {
                    tunnel: [enum16{"Stop", "Tests", "Bit test", "Start"}."Stop" enum16{"Stop", "Tests", "Bit test", "Start"}."Bit test"] -> w2902
                    tunnel: w2901 -> [w2912 _]
                    frame False {
                      n1052 = case shown="True" w2912 {
                        frame False {
                        }
                        frame True {
                          n1053 = call "Display Message to User4"() -> ()  [unwired: 10 in, 2 out]
                        }
                      }
                    }
                    frame True {
                    }
                  }
                }
              }
            }
            n1054 = Bundle By Name(cluster=T9 {"VISA"="COM1", "Array Test"=[]}, "VISA"=w2586, "Array Test"=w2592) -> (w2588:T9)
            n1055 = Enqueue Element(queue=w2594, element=w2588, error in (no error)=w2591) -> (queue out=w2589:refnum<queue>, error out=w2590:errorcluster)  [unwired: 2 out]
          }
          event "Report", "Stop Button": Value Change {
            w2955 = T31 1 items=["User Home"=0, "User Desktop"=1, "User Documents"=2, "User Application Data"=3, "User Preferences"=4, "User Temporary"=5, "Public Documents"=6, "Public Application Data"=7, "Public Preferences"=8, "Public Cache"=13, "System Core Libraries"=9, "System Installed Libraries"=10, "Application Files"=11, "Boot Volume Root"=12] ("system directory type")
            w2987 = "Marvin" ("section")
            n1056 = event-data() -> ("CtlRef"=w2979:refnum<vi>)  [unwired: 1 in]
            n1057 = local read "UUT"() -> (w2952:string)
            n1058 = call <vilib>:"Get System Directory.vi"("system directory type"=w2955) -> ("system directory"=w2954:path)  [unwired: 10 in]
            n1059 = Build Path(base path=w2954, name or relative path="MarvinReports") -> (appended path=w3016:path)
            n1060 = property on="CAN Status" class="Bool (strict)"() -> ("Value"=w2958:bool)  [unwired: 2 in, 2 out]
            n1061 = property on="Status" class="Bool (strict)"() -> ("Value"=w2959:bool)  [unwired: 2 in, 2 out]
            n1062 = case shown="\"AHU\"" w2952 {
              tunnel: ["REV EBAY" ("key") "REV AHU" ("key")] -> w2985
              frame "EBAY", Default {
              }
              frame "AHU" {
              }
            }
            n1063 = call <vilib>:"Check if File or Folder Exists.vi"("path"=w3016) -> ("error out"=w3014:errorcluster, "file or folder exists?"=w3017:bool, "dup path"=w3015:path)  [unwired: 8 in]
            n1064 = And(x=w2959, y=w2958) -> (x .and. y?=w2960:bool)
            n1065 = case shown="False" w3017 {
              tunnel: w3014 -> [w3081 w3082]
              tunnel: w3015 -> [w3080 w3083]
              tunnel: [w3079 w3083] -> w2957
              tunnel: [w3078 w3082] -> w3019
              frame False {
                n1066 = Create Folder(path (use dialog)=w3080, error in=w3081) -> (created path=w3079:path, error out=w3078:errorcluster)  [unwired: 1 in, 1 out]
              }
              frame True {
              }
            }
            n1067 = case shown="True" w2960 {
              tunnel: [w3026 w3046] -> w3003
              tunnel: [w3026 w3045] -> w2945
              tunnel: w2980 -> [_ w3034]
              tunnel: [w3026 w3039] -> w2950
              tunnel: [w3026 w3038] -> w2947
              tunnel: [w3026 w3042] -> w2973
              tunnel: [w3026 w3041] -> w2949
              tunnel: [w3026 w3030] -> w2946
              frame False {
                (unwired) "47"
                (unwired) " 413-8005_47_AHU"
                (unwired) "413-8005-1-47"
                (unwired) "5.3.9" ("read buffer")
                (unwired) "95"
                (unwired) "414-8005_95_EBAY_"
                (unwired) "414-8005-95"
                (unwired) "414-8005-95   "
                w3026 = "N_A" ("read buffer")
                n1068 = disable-structure shown="Disabled" {
                  frame Disabled {
                    n1069 = call "Display Message to User7"() -> ()  [unwired: 10 in, 2 out]
                  }
                  frame Enabled {
                  }
                }
                n1070 = Decimal String To Number(string="1" ("Value")) -> (number=w3027:i32)  [unwired: 2 in, 1 out]
                n1071 = Number To Decimal String(number=w3027, width (-)=i16 4) -> ()  [unwired: 1 out]
              }
              frame True {
                n1072 = call "SerialMarvinSendGet.vi"("write buffer"="SN\r\n", "VISA resource name"=w3034) -> ("error out"=w3033:errorcluster, "read buffer"=w3036:string)  [unwired: 8 in]
                n1073 = call "Time Delay2"("error in (no error)"=w3033) -> ("error out"=w3032:errorcluster)  [unwired: 10 in]
                n1074 = Decimal String To Number(string=w3036) -> (number=w3035:i32)  [unwired: 2 in, 1 out]
                n1075 = Number To Decimal String(number=w3035, width (-)=i16 4) -> (decimal integer string=w3039:string)
                n1076 = call "SerialMarvinSendGet.vi"("error in (no error)"=w3032, "write buffer"="VR\r\n", "VISA resource name"=w3034) -> ("error out"=w3043:errorcluster, "read buffer"=w3038:string)  [unwired: 7 in]
                n1077 = property on="UUT" class="DigNum (strict)"(error in=w3043) -> ("Value"=w3031:u8)  [unwired: 1 in, 2 out]
                n1078 = call "SentenceFromFile (SubVI).vi"("UUT"=w3031) -> ("Sentence"=w3030:string)  [unwired: 9 in, 1 out]
                n1079 = case shown="95, Default" w3031 {
                  tunnel: ["414-8005_95_EBAY_" " 413-8005_47_AHU" " 413-8005_63_AHU"] -> w3046
                  tunnel: ["414-8005-95   " w3052 w3055] -> w3045
                  tunnel: ["414-8005-95" w3052 w3055] -> w3042
                  tunnel: ["95" "47" "63"] -> w3041
                  frame 95, Default {
                  }
                  frame 47 {
                    w3052 = "413-8005-1-47"
                    (unwired) "AHU-L (47) 413-8005-1"
                  }
                  frame 63 {
                    w3055 = "413-8005-2-63"
                    (unwired) "AHU-R (63) 413-8005-2"
                  }
                }
              }
            }
            n1080 = Get Date/Time String(want seconds? (F)=TRUE) -> (date string=w3018:string)  [unwired: 2 in, 1 out]
            n1081 = call <vilib>:"Open Config Data.vi"("create file if necessary (T)"=FALSE, "configuration file path"=w2982) -> ("refnum"=w2994:T12)  [unwired: 1 in, 8 out]
            n1082 = property on="POWER Board S/N" class="Str"() -> ("Value"=w2944:string)  [unwired: 2 in, 2 out]
            n1083 = property on="Logger Path" class="Path"(error in=w3019, "Value"=w2957, "StartPath"=w2957) -> (error out=w2997:errorcluster)  [unwired: 1 in, 1 out]
            n1084 = Search and Replace String(replace all?=TRUE ("replace all? (F)"), input string=w3018, search string="/") -> (result string=w3000:string)  [unwired: 5 in, 3 out]
            n1085 = call-poly <vilib>:"Read Key.vi"("section"=w2987, "key"=w2985, "refnum"=w2994) -> ("error out"=w2989:errorcluster, "value"=w2992:string, "refnum out"=w2991:T12)  [unwired: 5 in, 1 out]
            n1086 = property on="DSP Board S/N" class="Str"() -> ("Value"=w2943:string)  [unwired: 2 in, 2 out]
            n1087 = call-poly <vilib>:"Read Key.vi"("section"=w2987, "error in (no error)"=w2989, "key"="Tester Software Ver", "refnum"=w2991) -> ("error out"=w2986:errorcluster, "value"=w2948:string, "refnum out"=w2990:T12)  [unwired: 4 in, 1 out]
            n1088 = Concatenate Strings("ATR" ("string"), w3003, w2950, "_", w3000, ".docx" ("string")) -> (w2998:string)
            n1089 = call <vilib>:"Close Config Data.vi"("error in (no error)"=w2986, "refnum"=w2990) -> ()  [unwired: 8 in, 2 out]
            n1090 = Build Path(base path=w2957, name or relative path=w2998) -> (appended path=w2999:path)
            n1091 = Concatenate Strings("  Rev-" ("string"), w2992) -> (w2981:string)
            n1092 = while {
              tunnel: w2998 -> [w3063]
              tunnel: w2957 -> [w3060]
              shift-right: [w3062] -> w2996
              shift-left: w2999 -> [w3061]
              shift-right: [w3058] -> w2983
              shift-left: w2984 -> [w3059]
              tunnel: w2997 -> [w3064]
              tunnel: [w3065] -> w2956
              stop <- w3057 continue-if-true
              n1093 = call <vilib>:"Check if File or Folder Exists.vi"("error in (no error)"=w3064, "path"=w3061) -> ("error out"=w3065:errorcluster, "file or folder exists?"=w3057:bool)  [unwired: 7 in, 1 out]
              n1094 = case shown="True" w3057 {
                tunnel: w3063 -> [_ w3077]
                tunnel: w3059 -> [_ w3069]
                tunnel: [w3067 w3074] -> w3062
                tunnel: w3061 -> [w3067 _]
                tunnel: w3060 -> [_ w3075]
                tunnel: [1 w3068] -> w3058
                frame False {
                }
                frame True {
                  w3070 = ".docx" ("search string")
                  n1095 = Search and Replace String(input string=w3077, search string=w3070) -> (result string=w3076:string)  [unwired: 6 in, 3 out]
                  n1096 = Number To Decimal String(number=w3069) -> (decimal integer string=w3072:string)  [unwired: 1 in]
                  n1097 = call <vilib>:"Space Constant.vi"() -> ("String"=w3071:string)
                  n1098 = Concatenate Strings(w3076, w3071, w3072, w3070) -> (w3073:string)
                  n1099 = Build Path(base path=w3075, name or relative path=w3073) -> (appended path=w3074:path)
                  n1100 = Increment(x=w3069) -> (x+1=w3068:i32)
                }
              }
            }
            n1101 = call "HeaderBis.vi"("UUTHeader"=w2952, "UA"=w2949, "POWER SN"=w2944, "Revision Param"=w2946, "P/N UUT"=w2945, "DSP SN"=w2943, "Driver S/N"=w2950, "VR"=w2947, "Oper."=w2951, "Tester Software Ver"=w2948) -> ("table header"=w2942:string, "Array"=w2941:string[][])  [unwired: 3 in, 1 out]
            n1102 = Open/Create/Replace File(file path (use dialog)=w2996, error in=w2956, operation (0:open)=T25."create") -> (error out=w3009:errorcluster)  [unwired: 3 in, 2 out]
            n1103 = control-ref of="ATR"() -> (w3021:refnum<vi>)
            n1104 = property class="Tbl (strict)"(reference=w3021, error in=w3009) -> ("Value"=w3022:string[][])  [unwired: 2 out]
            n1105 = call "MarvinReport.vi"("HEADER1"=w2942, "ATR Or"=w3021, "Steps   pfull"=w3022, "Footer UUT"=w2973, "pageNum"=3, "InputHeaderArray"=w2941, "FILE NAME"=w2998, "Report Folder"=w2996, "REV"=w2981, "Test-Conductor"=w2951) -> ("error out"=w2968:errorcluster)  [unwired: 4 in, 1 out]
            n1106 = call <vilib>:"Clear Errors.vi"("error in (no error)"=w2968) -> ("error out"=w2967:errorcluster)  [unwired: 5 in, 1 out]
            n1107 = property class="Bool (strict)"(reference=w2979, error in=w2967) -> ("BoolText.Text"=w2978:string)  [unwired: 2 out]
            n1108 = Equal?(x=w2978, y="Report") -> (x = y?=w2972:bool)
            n1109 = Select(t=T11."MainProgram", s=w2972, f=T11."Stop") -> (s? t:f=w2975:T11)
            n1110 = Select(t="Save Report...", s=w2972, f="Program Stopped...\r\nPlease turn OFF All Power sinks") -> (s? t:f=w2970:string)
            n1111 = property on="Report" class="Bool (strict)"(error in=w2967, "Value"=FALSE ("Report")) -> (error out=w2961:errorcluster)  [unwired: 1 in, 1 out]
            n1112 = property on="VISA Tester" class="VISAName"() -> ("Value"=w2965:refnum<visa-resource-name>)  [unwired: 2 in, 2 out]
            n1113 = property on="Pannel User Message" class="Str"("Value"=w2970) -> ()  [unwired: 2 in, 2 out]
            n1114 = call "TesterOption (SubVI).vi"("2 Options"=FALSE, "error in (no error)"=w2961, "On/Off"=FALSE, "Tester Option"=T13."Venable", "VISA Refnum in"=w2965) -> ()  [unwired: 5 in, 2 out]
          }
          event "Help Button": Value Change {
            n1115 = event-data() -> ()  [unwired: 1 in, 6 out]
            n1116 = vi-ref "Help.vi"() -> (w3097:refnum<vi>)
            n1117 = invoke class="VI" method="FP.Open"(reference=w3097, error in=w3095, "Activate"=TRUE ("Activate?"), "State"=T23."Standard") -> (error out=w3096:errorcluster)  [unwired: 1 in, 4 out]
            n1118 = call "Help.vi"("error in"=w3096, "TesterSWVersion"=w3087) -> ("error out"=w3094:errorcluster)  [unwired: 6 in]
            n1119 = property on="Help Button" class="Bool (strict)"("Value"=FALSE ("Help Button")) -> ()  [unwired: 2 in, 2 out]
          }
          event "Serial Com": Value Change {
            n1120 = event-data() -> ()  [unwired: 1 in, 6 out]
            n1121 = property on="Serial Com" class="Bool"(error in=w3108, "Visible"=FALSE) -> (error out=w3112:errorcluster)  [unwired: 1 in, 1 out]
            n1122 = property on="VISA Marvin" class="VISAName"(error in=w3112, "Visible"=TRUE) -> (error out=w3109:errorcluster)  [unwired: 1 in, 1 out]
          }
          event "VISA Marvin": Value Change {
            n1123 = event-data() -> ()  [unwired: 1 in, 6 out]
            n1124 = property on="Serial Com" class="Bool"(error in=w3117, "Visible"=FALSE) -> (error out=w3116:errorcluster)  [unwired: 1 in, 1 out]
            n1125 = control-ref of="This VI"() -> (w3128:refnum<vi>)
            n1126 = property on="Pannel User Message" class="Str"(error in=w3117, "Value"="Serial connection in process" ("Pannel User Message")) -> ()  [unwired: 1 in, 2 out]
            n1127 = call "Serial InitMarvin.vi"("error in (no error)"=w3116, "VI reference (current VI)"=w3128, "VISA Refnum in"="VISA Marvin") -> ("error out"=w3120:errorcluster, "Boolean"=w3118:bool)  [unwired: 7 in]
            n1128 = property on="VISA Marvin" class="VISAName"(error in=w3120, "Visible"=FALSE) -> (error out=w3131:errorcluster)  [unwired: 1 in, 1 out]
            n1129 = property on="Serial Com" class="Bool"(error in=w3131, "Visible"=TRUE) -> (error out=w3127:errorcluster)  [unwired: 1 in, 1 out]
            n1130 = case shown="True" w3118 {
              tunnel: w3127 -> [w3134 w3146]
              tunnel: "VISA Marvin" -> [w3135 w3143]
              tunnel: [w3135 w3142] -> w3122
              tunnel: [w3134 w3141] -> w3121
              frame False {
              }
              frame True {
                n1131 = call "SerialMarvinSendGet.vi"("error in (no error)"=w3146, "Clear Log"=FALSE, "write buffer"="VC\r\n", "VISA resource name"=w3143) -> ("error out"=w3145:errorcluster, "read buffer"=w3139:string)  [unwired: 6 in]
                n1132 = Decimal String To Number(string=w3139) -> (number=w3138:i32)  [unwired: 2 in, 1 out]
                n1133 = Less Or Equal?(x=w3138, y=50) -> (x <= y?=w3136:bool)
                n1134 = property on="Status" class="Bool (strict)"("Value"=w3136) -> ()  [unwired: 2 in, 2 out]
                n1135 = case shown="True" w3136 {
                  tunnel: w3145 -> [w3147 w3176]
                  tunnel: w3143 -> [w3148 w3175]
                  tunnel: [w3148 w3166] -> w3142
                  tunnel: [w3147 w3149] -> w3141
                  frame False {
                  }
                  frame True {
                    n1136 = call <vilib>:"Clear Errors.vi"("error in (no error)"=w3176) -> ("error out"=w3177:errorcluster)  [unwired: 5 in, 1 out]
                    n1137 = control-ref of="ATR"() -> (w3163:refnum<vi>)
                    n1138 = VISA Flush I/O Buffer(VISA resource name=w3175, error in (no error)=w3177) -> (VISA resource name out=w3166:refnum<visa-resource-name>, error out=w3174:errorcluster)  [unwired: 1 in]
                    n1139 = call "Display Message to User2"("error in (no error)"=w3174) -> ("error out"=w3173:errorcluster, "Yes"=w3172:bool)  [unwired: 9 in]
                    n1140 = case shown="True" w3172 {
                      tunnel: w3173 -> [w3178 w3200]
                      tunnel: [w3178 w3179] -> w3171
                      tunnel: w3166 -> [_ w3197]
                      frame False {
                      }
                      frame True {
                        w3185 = FALSE ("2 Options")
                        n1141 = property on="UUT" class="DigNum (strict)"() -> ("Value"=w3199:u8)  [unwired: 2 in, 2 out]
                        n1142 = call "SetParam.vi"("RS"=TRUE, "error in (no error)"=w3200, "Param to Set in"=w3199, "Visa"=w3197) -> ("error out"=w3180:errorcluster)  [unwired: 7 in]
                        n1143 = control-ref of="Pannel User Message"() -> (w3196:refnum<vi>)
                        n1144 = control-ref of="Stop Burn-in"() -> (w3194:refnum<vi>)
                        n1145 = control-ref of="Stop Button"() -> (w3195:refnum<vi>)
                        n1146 = control-ref of="Motor Speed RPM"() -> (w3193:refnum<vi>)
                        n1147 = property on="VISA Tester" class="VISAName"() -> ("Value"=w3189:refnum<visa-resource-name>)  [unwired: 2 in, 2 out]
                        n1148 = call "TesterOption (SubVI).vi"("2 Options"=w3185, "error in (no error)"=w3180, "On/Off"=FALSE, "Tester Option"=T13."Power", "VISA Refnum in"=w3189) -> ("error out"=w3190:errorcluster, "VISA Refnum out"=w3192:refnum<visa-resource-name>)  [unwired: 5 in]
                        n1149 = call "Write panel message (SubVI).vi"("Stop BurnIn"=w3194, "rpm"=w3193, "PrintTime"=TRUE, "Stop"=w3195, "error in (no error)"=w3190, "Time to wait"=20.0, "Strin"="Restart the UUT\nPlease wait...", "String in"=w3196) -> ("error out"=w3191:errorcluster)  [unwired: 3 in]
                        n1150 = call "TesterOption (SubVI).vi"("2 Options"=w3185, "error in (no error)"=w3191, "On/Off"=FALSE, "Tester Option"=T13."Venable", "VISA Refnum in"=w3192) -> ("error out"=w3179:errorcluster)  [unwired: 5 in, 1 out]
                      }
                    }
                    n1151 = call "Find_Number_LineMARVIN.vi"("Test Paragraph"="Sensor Reading Analog Offset", "TableIn"=w3163) -> ("Line number"=w3164:i32)  [unwired: 3 in, 3 out]
                    n1152 = call "SerialMarvinSendGet.vi"("error in (no error)"=w3171, "write buffer"="SN\r\n", "VISA resource name"=w3166) -> ("error out"=w3167:errorcluster, "read buffer"=w3156:string)  [unwired: 7 in]
                    n1153 = call "SerialMarvinSendGet.vi"("error in (no error)"=w3167, "write buffer"="AO[1]\r\n", "VISA resource name"=w3166) -> ("error out"=w3161:errorcluster, "read buffer"=w3162:string)  [unwired: 7 in]
                    n1154 = Fract/Exp String To Number(string=w3162) -> (number=w3158:dbl)  [unwired: 3 in, 1 out]
                    n1155 = In Range and Coerce(upper limit=0.1 ("x"), x=w3158, lower limit=-0.1) -> (In Range?=w3157:bool)  [unwired: 1 out]
                    n1156 = call "PassOrFail (SubVI).vi"("Test#"="2", "index (row)"=w3164, "error in (no error)"=w3161, "Data in"=w3158, "Pass?Fail"=w3157, "Table in"=w3163) -> ("error out"=w3150:errorcluster)  [unwired: 5 in]
                    n1157 = property on="VISA Marvin" class="VISAName"(error in=w3150) -> (error out=w3153:errorcluster, "Value"=w3154:refnum<visa-resource-name>)  [unwired: 1 in, 1 out]
                    n1158 = call "SerialMarvinSendGet.vi"("error in (no error)"=w3153, "Clear Log"=FALSE, "write buffer"="EP=1\r\nMD[1]=1\r\n", "VISA resource name"=w3154) -> ("error out"=w3149:errorcluster)  [unwired: 6 in, 1 out]
                    n1159 = property on="UUT SN Report" class="Str"("Value"=w3156) -> ()  [unwired: 2 in, 2 out]
                    n1160 = Decimal String To Number(string=w3156) -> (number=→"Current SN":i32)  [unwired: 2 in, 1 out]
                  }
                }
              }
            }
          }
          event "Refresh Button": Value Change {
            n1161 = event-data() -> ()  [unwired: 1 in, 6 out]
          }
          event "Settings": Value Change {
            n1162 = event-data() -> ()  [unwired: 1 in, 6 out]
            n1163 = control-ref of="VISA Tester"() -> (w3214:refnum<vi>)
            n1164 = control-ref of="UUT"() -> (w3212:refnum<vi>)
            n1165 = property on="Status" class="Bool (strict)"() -> ("Value"=w3216:bool)  [unwired: 2 in, 2 out]
            n1166 = case shown="True" w3216 {
              tunnel: w3222 -> [_ w3234]
              tunnel: [w3223 w3229] -> w3217
              tunnel: w3215 -> [_ w3228]
              tunnel: w3214 -> [_ w3227]
              tunnel: w3213 -> [_ w3226]
              tunnel: w3212 -> [_ w3225]
              frame False {
                n1167 = call "Display Message to User8"() -> ("error out"=w3223:errorcluster)  [unwired: 10 in, 1 out]
              }
              frame True {
                n1168 = vi-ref "Calibration (SubVI).vi"() -> (w3233:refnum<vi>)
                n1169 = invoke class="VI" method="FP.Open"(reference=w3233, error in=w3234, "Activate"=TRUE ("Activate?"), "State"=T23."Standard") -> (error out=w3230:errorcluster)  [unwired: 1 in, 4 out]
                n1170 = call "Calibration (SubVI).vi"("VISA UUT"=w3228, "error constant"=w3230, "UUT"=w3225, "CAN Cluster in"=w3226, "Visa Tester"=w3227) -> ("error constant 2"=w3229:errorcluster, "AO[1]Meas"=→"Cal":dbl)  [unwired: 5 in]
              }
            }
          }
        }
      }
      frame "Initialize" {
        w3235 = 0
        w3240 = FALSE ("Visible")
        w3241 = FALSE ("Visible")
        w3242 = FALSE ("Visible")
        w3243 = FALSE ("Visible")
        w3254 = refnum<visa-resource-name> "COM1" ("VISA resource name")
        w3245 = FALSE ("Visible")
        w3238 = FALSE ("Serial Status")
        n1171 = property on="ComTestResult" class="Bool (strict)"("Value"=w3243) -> ()  [unwired: 2 in, 2 out]
        n1172 = property on="VenableResult" class="Bool (strict)"("Value"=w3243) -> ()  [unwired: 2 in, 2 out]
        n1173 = property on="VenableDirectionResult" class="Bool (strict)"("Value"=w3243) -> ()  [unwired: 2 in, 2 out]
        n1174 = property on="SpeedResult" class="Bool (strict)"("Value"=w3243) -> ()  [unwired: 2 in, 2 out]
        n1175 = property on="Serial Com" class="Bool"(error in=errorcluster {"status"=FALSE, "code"=0, "source"=""} ("error out"), "Visible"=TRUE) -> (error out=w3256:errorcluster)  [unwired: 1 in, 1 out]
        n1176 = property on="AuxiOFFResult" class="Bool (strict)"("Value"=w3242) -> ()  [unwired: 2 in, 2 out]
        n1177 = property on="AuxiONResult" class="Bool (strict)"("Value"=w3242) -> ()  [unwired: 2 in, 2 out]
        n1178 = property on="VisualInspectionResult" class="Bool (strict)"("Value"=w3242) -> ()  [unwired: 2 in, 2 out]
        n1179 = property on="SensCalResult" class="Bool (strict)"("Value"=w3242) -> ()  [unwired: 2 in, 2 out]
        n1180 = property on="VISA Marvin" class="VISAName"(error in=w3256, "Visible"=w3245, "Value"=w3254) -> (error out=w3246:errorcluster)  [unwired: 1 in, 1 out]
        n1181 = property on="Stop Burn-in" class="Bool (strict)"(error in=w3246, "Visible"=w3245) -> (error out=w3239:errorcluster)  [unwired: 1 in, 1 out]
        n1182 = property on="BurnDC" class="Bool (strict)"("Value"=w3241) -> ()  [unwired: 2 in, 2 out]
        n1183 = property on="BurnTemp" class="Bool (strict)"("Value"=w3241) -> ()  [unwired: 2 in, 2 out]
        n1184 = property on="BurnSpeed" class="Bool (strict)"("Value"=w3241) -> ()  [unwired: 2 in, 2 out]
        n1185 = property on="BurnResult" class="Bool (strict)"("Value"=w3241) -> ()  [unwired: 2 in, 2 out]
        n1186 = property on="Refresh Button" class="Bool (strict)"(error in=w3239, "Value"=FALSE ("Refresh Button")) -> ()  [unwired: 1 in, 2 out]
        n1187 = property on="StopTimeResult" class="Bool (strict)"("Value"=w3240) -> ()  [unwired: 2 in, 2 out]
        n1188 = property on="MotorTempResult" class="Bool (strict)"("Value"=w3240) -> ()  [unwired: 2 in, 2 out]
        n1189 = property on="TempControlResult" class="Bool (strict)"("Value"=w3240) -> ()  [unwired: 2 in, 2 out]
        n1190 = property on="Automation" class="Bool (strict)"("Value"=w3240) -> ()  [unwired: 2 in, 2 out]
        n1191 = flat-sequence {
          tunnel: w3239 -> [w3258]
          tunnel: [w3258] -> w3236
          tunnel: [w3260] -> w3252
          tunnel: w3236 -> [w3260]
          tunnel: [w3272] -> w3251
          tunnel: w3252 -> [w3273]
          tunnel: [w3273] -> w3250
          frame #0 {
          }
          frame #1 {
            w3263 = u32 4294967295  # AccMask
            w3259 = T5 0 items=["使用Flash参数", "使用界面设置参数"] ("InitFlag")
            w3261 = T7 0 items=["normal operation", "Listen-only mode", "test mode"]  # Mode
            w3262 = T6 3 items=["接收所有类型"=1, "只接收标准帧"=2, "只接收扩展帧"=3] ("Fliter")
            w3267 = u8 10 items=["5k bps"=1, "10k bps"=2, "20k bps"=3, "40k bps"=4, "50k bps"=5, "80k bps"=6, "100k bps"=7, "125k bps"=8, "200k bps"=9, "250k bps"=10, "400k bps"=11, "500k bps"=12, "666k bps"=13, "800k bps"=14, "1000k bps"=15, "33.33k bps"=16, "66.66k bps"=17, "83.33k bps"=18]  # kBaudRate
            w3264 = u32 0  # AccCode
            w3265 = T3 4 items=["USB-CAN"=3, "USB-CAN2"=4] ("DevType")
            w3266 = T8 {"DevType"=3, "DevIndex"=0, "CanIndex"=0, "VCI_INIT_CONFIG"={"AccCode"=0, "AccMask"=0, "InitFlag"=1, "Fliter"=7, "Timing0"=0, "Timing1"=0, "Mode"=0}}  # Config
            # "CANalystII"
            n1192 = call "Demo_GetT0T1.vi"("kBaudRate"=w3267) -> ("Timing0"=w3269:u8, "Timing1"=w3270:u8)
            n1193 = Bundle By Name(cluster=w3266, "DevType"=w3265, "CanIndex"="Channel 2", "VCI_INIT_CONFIG.AccCode"=w3264, "VCI_INIT_CONFIG.AccMask"=w3263, "VCI_INIT_CONFIG.InitFlag"=w3259, "VCI_INIT_CONFIG.Fliter"=w3262, "VCI_INIT_CONFIG.Timing0"=w3269, "VCI_INIT_CONFIG.Timing1"=w3270, "VCI_INIT_CONFIG.Mode"=w3261) -> (→"Config_CANAT":T8)
          }
          frame #2 {
            w3274 = u16 284 items=["1M"=20, "500K"=28, "250K"=284, "125K"=796, "100K"=17199, "50K"=18223, "20K"=21295, "10K"=26415, "5K"=32639] ("baud in")
            n1194 = control-ref of="Config_CANAT"() -> (w3272:refnum<vi>)
            n1195 = call "InitCAN_ATII.vi"("Config"=w3272) -> ("Sts"=→"CAN Status":bool)
            n1196 = call "ChangeCANBaud.vi"("baud in"=w3274, "reference"=w3272) -> ()
          }
        }
        "Status" <- w3238
        "Test Failed" <- w3238
      }
    }
  }
  n1197 = property on="Settings" class="Bool (strict)"("Visible"=w20) -> ()  [unwired: 2 in, 2 out]
  n1198 = property on="Cal" class="DigNum (strict)"("Visible"=w20) -> ()  [unwired: 2 in, 2 out]
  n1199 = disable-structure shown="Disabled" {
    frame Disabled {
      w3276 = T21."Disabled and Grayed Out" ("Disabled")
      w3277 = FALSE ("Start")
      n1200 = property on="VISA Tester" class="VISAName" props=["Value"]() -> ()  [unwired: 2 in, 3 out]
      n1201 = property on="Current SN" class="DigNum (strict)" props=["Value"]() -> ()  [unwired: 2 in, 3 out]
      n1202 = property on="UUT" class="DigNum (strict)" props=["Value"]() -> ()  [unwired: 2 in, 3 out]
      n1203 = property on="Status" class="Bool (strict)" props=["Value"]() -> ()  [unwired: 2 in, 3 out]
      n1204 = property on="UUT SoftwareVer" class="Str" props=["Value"]() -> ()  [unwired: 2 in, 3 out]
      n1205 = property on="Next SN" class="DigNum (strict)" props=["Value"]() -> ()  [unwired: 3 in, 2 out]
      n1206 = property on="Start" class="Bool (strict)"("Value"=w3277, "DisabledEnum"=w3276) -> ()  [unwired: 2 in, 2 out]
      n1207 = property on="Report" class="Bool (strict)"("Value"=w3277, "DisabledEnum"=w3276) -> ()  [unwired: 2 in, 2 out]
    }
    frame Enabled {
    }
  }
  n1208 = disable-structure shown="Disabled" {
    frame Disabled {
      (unwired) 0.02003173828125 ("x")
      n1209 = control-ref of="Stop Burn-in"() -> ()  [unwired: 1 out]
      n1210 = control-ref of="Stop Button"() -> ()  [unwired: 1 out]
      n1211 = control-ref of="Motor Speed RPM"() -> ()  [unwired: 1 out]
      n1212 = control-ref of="Config_CANAT"() -> ()  [unwired: 1 out]
      n1213 = control-ref of="UUT"() -> ()  [unwired: 1 out]
      n1214 = call "GetADCTester (SubVI).vi"() -> ()  [unwired: 9 in, 3 out]
      n1215 = call "CANSendMotorSpeed.vi"() -> ()  [unwired: 11 in, 1 out]
      n1216 = control-ref of="Config_CANAT"() -> ()  [unwired: 1 out]
      n1217 = call "Find_Number_LineMARVIN.vi"() -> ()  [unwired: 5 in, 4 out]
      n1218 = property on="UUT" class="DigNum (strict)" props=["Value"]() -> ()  [unwired: 2 in, 3 out]
      n1219 = control-ref of="UUT"() -> ()  [unwired: 1 out]
      n1220 = call "DegToDAC (SubVI).vi"() -> ()  [unwired: 10 in, 2 out]
      n1221 = call "Write panel message (SubVI).vi"() -> ()  [unwired: 11 in, 1 out]
      n1222 = property on="VISA Tester" class="VISAName" props=["Value"]() -> ()  [unwired: 2 in, 3 out]
      n1223 = control-ref of="ATR"() -> ()  [unwired: 1 out]
      n1224 = call "TesterOption (SubVI).vi"() -> ()  [unwired: 10 in, 2 out]
      n1225 = call "TesterOption (SubVI).vi"() -> ()  [unwired: 10 in, 2 out]
      n1226 = call "PassOrFail (SubVI).vi"() -> ()  [unwired: 11 in, 1 out]
    }
    frame Enabled {
    }
  }
  n1227 = disable-structure shown="Disabled" {
    frame Disabled {
      n1228 = flat-sequence {
        frame #0 {
          n1229 = call "CANSendMotorSpeed.vi"("Remote"=TRUE, "Motor Speed RPM"=u16 0) -> ("error out"=w3279:errorcluster, "UUT"=w3282:refnum<vi>)  [unwired: 8 in]
          n1230 = property on="VISA Tester" class="VISAName"() -> ("Value"=w3278:refnum<visa-resource-name>)  [unwired: 2 in, 2 out]
          n1231 = call "TesterOption (SubVI).vi"("error in (no error)"=w3279, "On/Off"=FALSE, "Tester Option"=T13."Power", "VISA Refnum in"=w3278) -> ()  [unwired: 6 in, 2 out]
        }
      }
    }
    frame Enabled {
    }
  }
  "Pannel User Message" <- w19
